vi "results_interface.vi"() -> ()   [LabVIEW 2015]
panel:
  out "Exerimement List by Group":string[](array[string])
  out "List of experiments":string[](array[string])
  out "Exeperiments names":string[](array[string])
  out "Experiment Group Names List":string[](array[string])
  out "Batch List by Material":string[](array[string])
  out "Batch list without IDs":string[](array[string])
  out "List of material IDs":string[](array[string])
  out "Material Name List":string[](array[string])
  out "Delimited Input String":string
  in  "Tab Control":enum32{"Controls", "Insights", "Debug"}(tab)
  in  "Create Heatmap":bool
  in  "Maxiumum Mass (kg)":dbl=1.0000000000000113e-10 format="%#_4e"
  in  "Minimum Mass (kg)":dbl=1.000000000000002e-30 step=1.0 format="%#_6e"
  in  "Batches list":i32[](listbox)
  in  "Confirm Experiments":bool
  in  "Experiment Listbox":i32[](listbox)
  in  "Show expeirments":bool
  in  "Experiment ID":string="All"
  in  "Confirm Selection":bool
  out "Authentication Failure":bool
  in  "Authenticate":bool
  out "Numeric":dbl
  in  "Password":string="dust"
  in  "Username":string="root"
  in  "Server IP Address":string="localhost"
  out "Poor Rate":string
  out "Optimal Rate":string
  out "User warnings":string
  in  "Calculate Results":bool
  in  "End Program":bool
  in  "Velocity Minimun  (km/s)":dbl min=0.0 max=100.0
  in  "Dust Material":string(combo)="Any Material"
  in  "Estimate Session Quality":cluster{i32, i32}(slide)={3, 5} scale=0.0..5.0
  out "Valid Path":bool
  out "Finished Sessions":bool
  out "Calculating":bool
  in  "Estimate Dust Quality":cluster{i32, i32}(slide)={3, 5} scale=0.0..5.0
  in  "Dust ID":string="Any"
  in  "Lower Integer Timestamp":i64=1375737549000 min=1340137854565 max=2062085784667 step=10000000
  in  "Upper Integer Timestamp":i64=2225999960000 min=1340137854565 max=2040137854565 step=10000000
  in  "Upper Timestamp":timestamp=timestamp(4308844760.779092 s since 1904-01-01)
  in  "Lower Timestamp":timestamp=timestamp(3458582349.4224453 s since 1904-01-01)
  in  "Velocity Maximum (km/s)":dbl=100.0 min=0.0 max=100.0
  out "Average Rate of Particle Detection":string
  out "Calculating Sessions":bool
  out "Cleaning Up":bool
  out "Working Directory":path
  in  "List Batches":bool
  in  "Experiment Group":string(combo)
  out "Results Output":string
  in  "Tab Control 2":T1(tab)
  in  "Tab Control 4":T2(tab)
  out "avg rate":picture
  out "avg count":picture
  out "avg runtime":picture
  in  "Tab Control 5":T2(tab)
  out "optimal rates":picture
  out "optimal count":picture
  out "optimal runtime":picture
  in  "Tab Control 6":T2(tab)
  out "poor rates":picture
  out "poor counts":picture
  out "poor runtimes":picture
  in  "Tab Control 7":T3(tab)
  out "2D rates":picture
  out "2D particle distribution":picture
  out "2D runtime":picture
  in  "Tab Control 3":T4(tab)
  out "Session Quality Breakdown":picture
  out "Session Particle Quality Breakdown":picture
  out "Session Duration Breakdown":picture
  out "Session Dust Event Count Breakdown":picture
  out "Session Generator Output":string
  out "Results Error/Debug":string
  out "Rate Results Request":string
  # "Note: takes upwards of two minutes, placed in heatmap folder"
  # "To calculate the rate of dust detection over a velocty range, a set of histograms is made, with bins for each .1km/s. The total runtime, detections, and rate over each bin are then calculated. Keep in mind the graphs here while maintaining the trends seen, their values reflect the bin size."
  # "The sessions are designated a quality:\n1: Maintenance session\n2: Low number of particle detections <10\n3: Low runtime < 20 min\n4: Standard sessions\n5: High dust event count (productive session)"
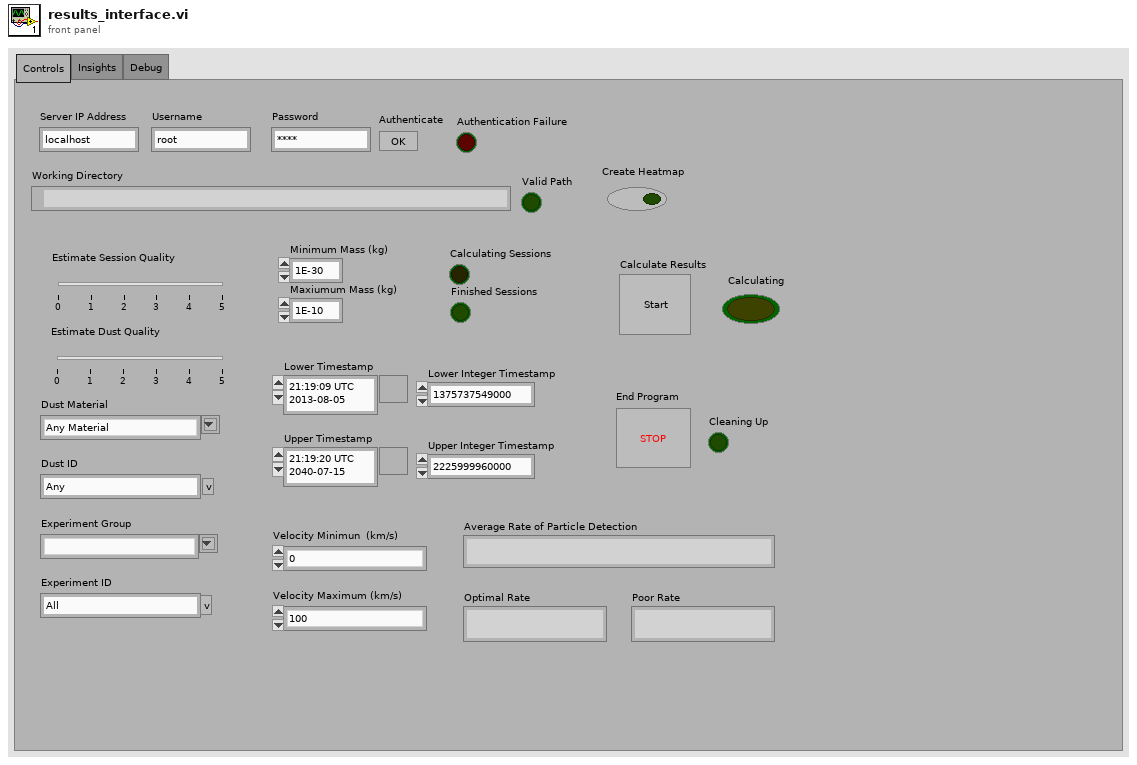
[diagram p1: front panel]
types:
  T1 = enum32{"Rate Insights - Average Results", "Rate Insights - Optimal Results", "Rate Insights - Poor Results", "Heatmaps", "Results Breakdown"}
  T2 = enum32{"Average Rates", "Average  Events", "Average Runtime"}
  T3 = enum32{"Particle Distribution", "Rate Distribution", "Runtime Distribution"}
  T4 = enum32{"Session Quality ", "Particle Quality", "Session Duration", "Session Event Counts"}
  T5 = cluster{string, string, string, string, string, string, string, string, string, string, string, string, string}
  T6 = cluster{"Velocity Minimun  (km/s)":dbl, "Velocity Maximum (km/s)":dbl}
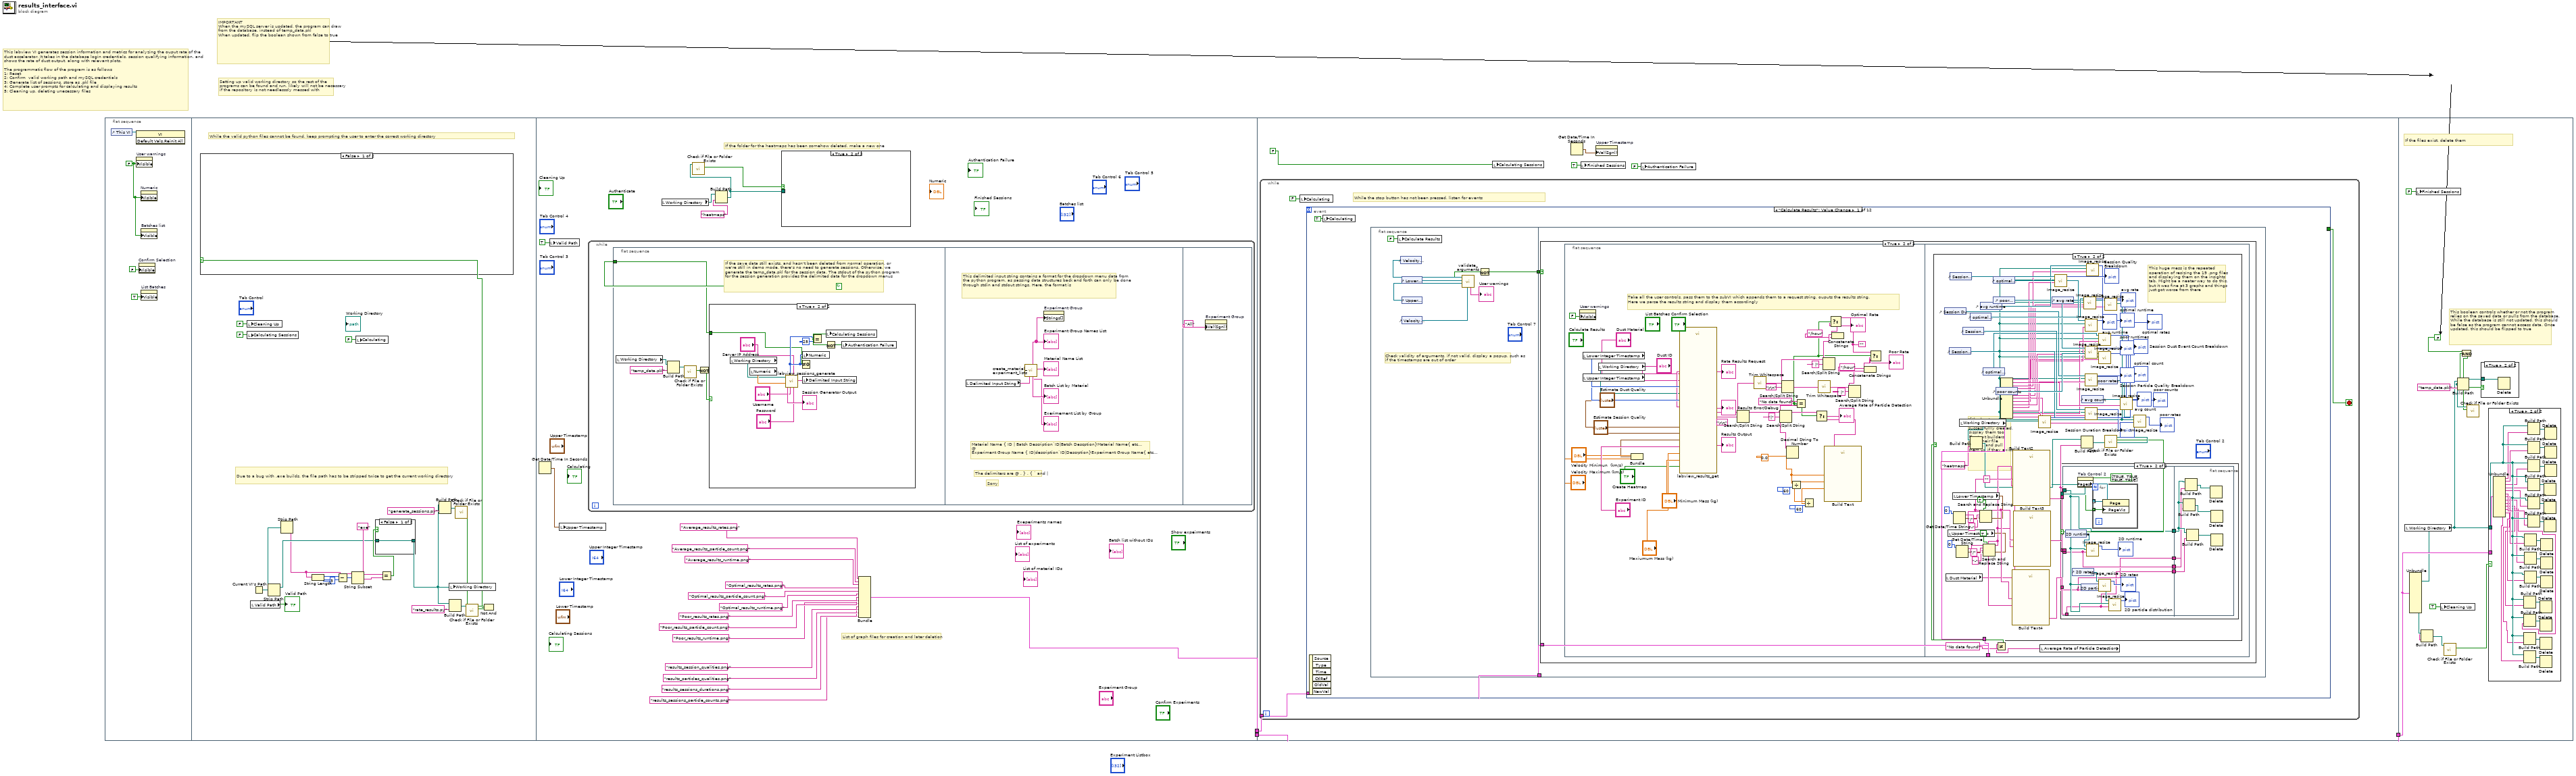
[diagram p0: block diagram]
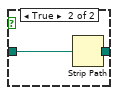
[diagram p2: hidden frame]
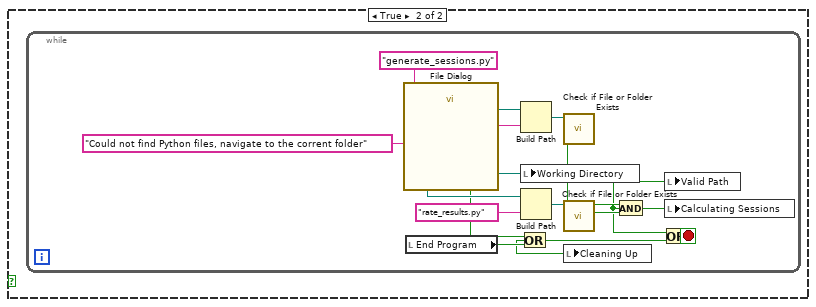
[diagram p3: hidden frame]
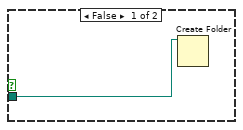
[diagram p4: hidden frame]
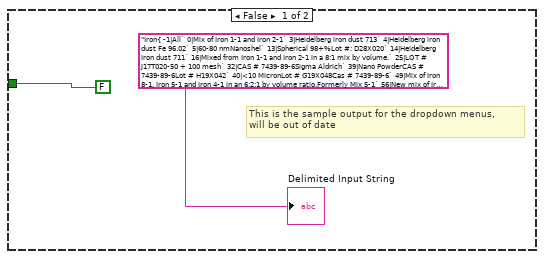
[diagram p5: hidden frame]
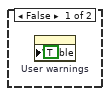
[diagram p6: hidden frame]
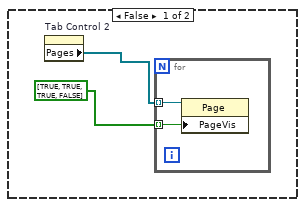
[diagram p8: hidden frame]
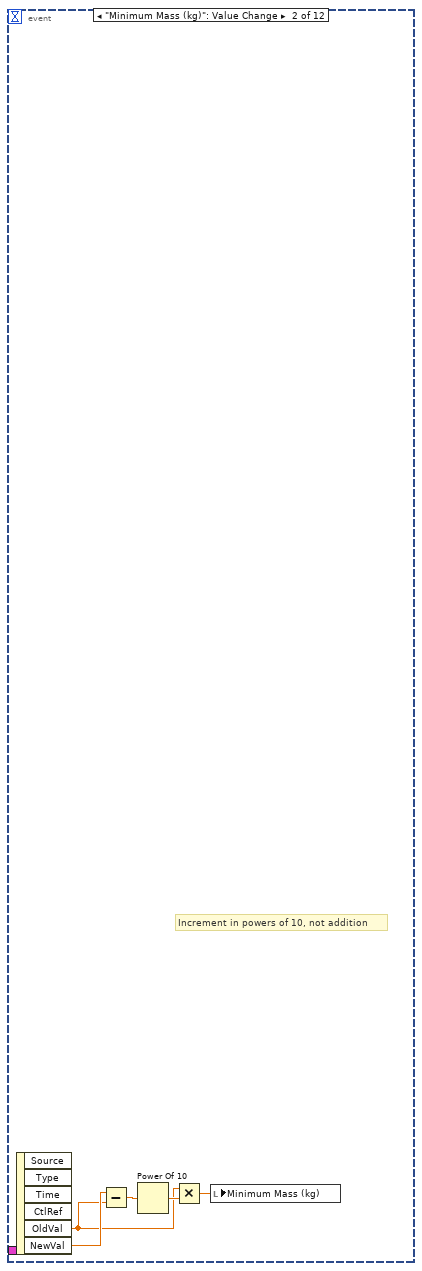
[diagram p9: hidden frame]
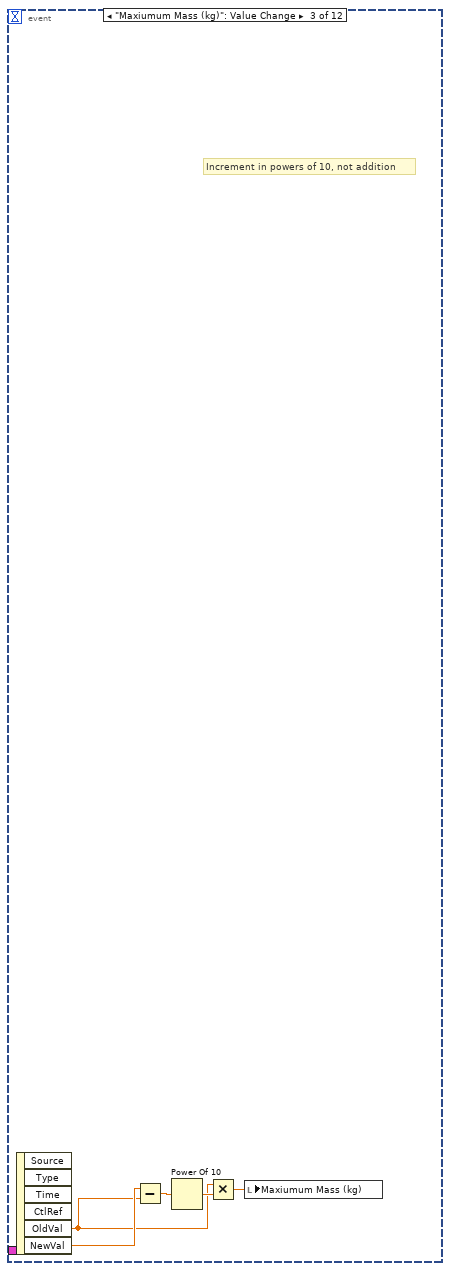
[diagram p10: hidden frame]
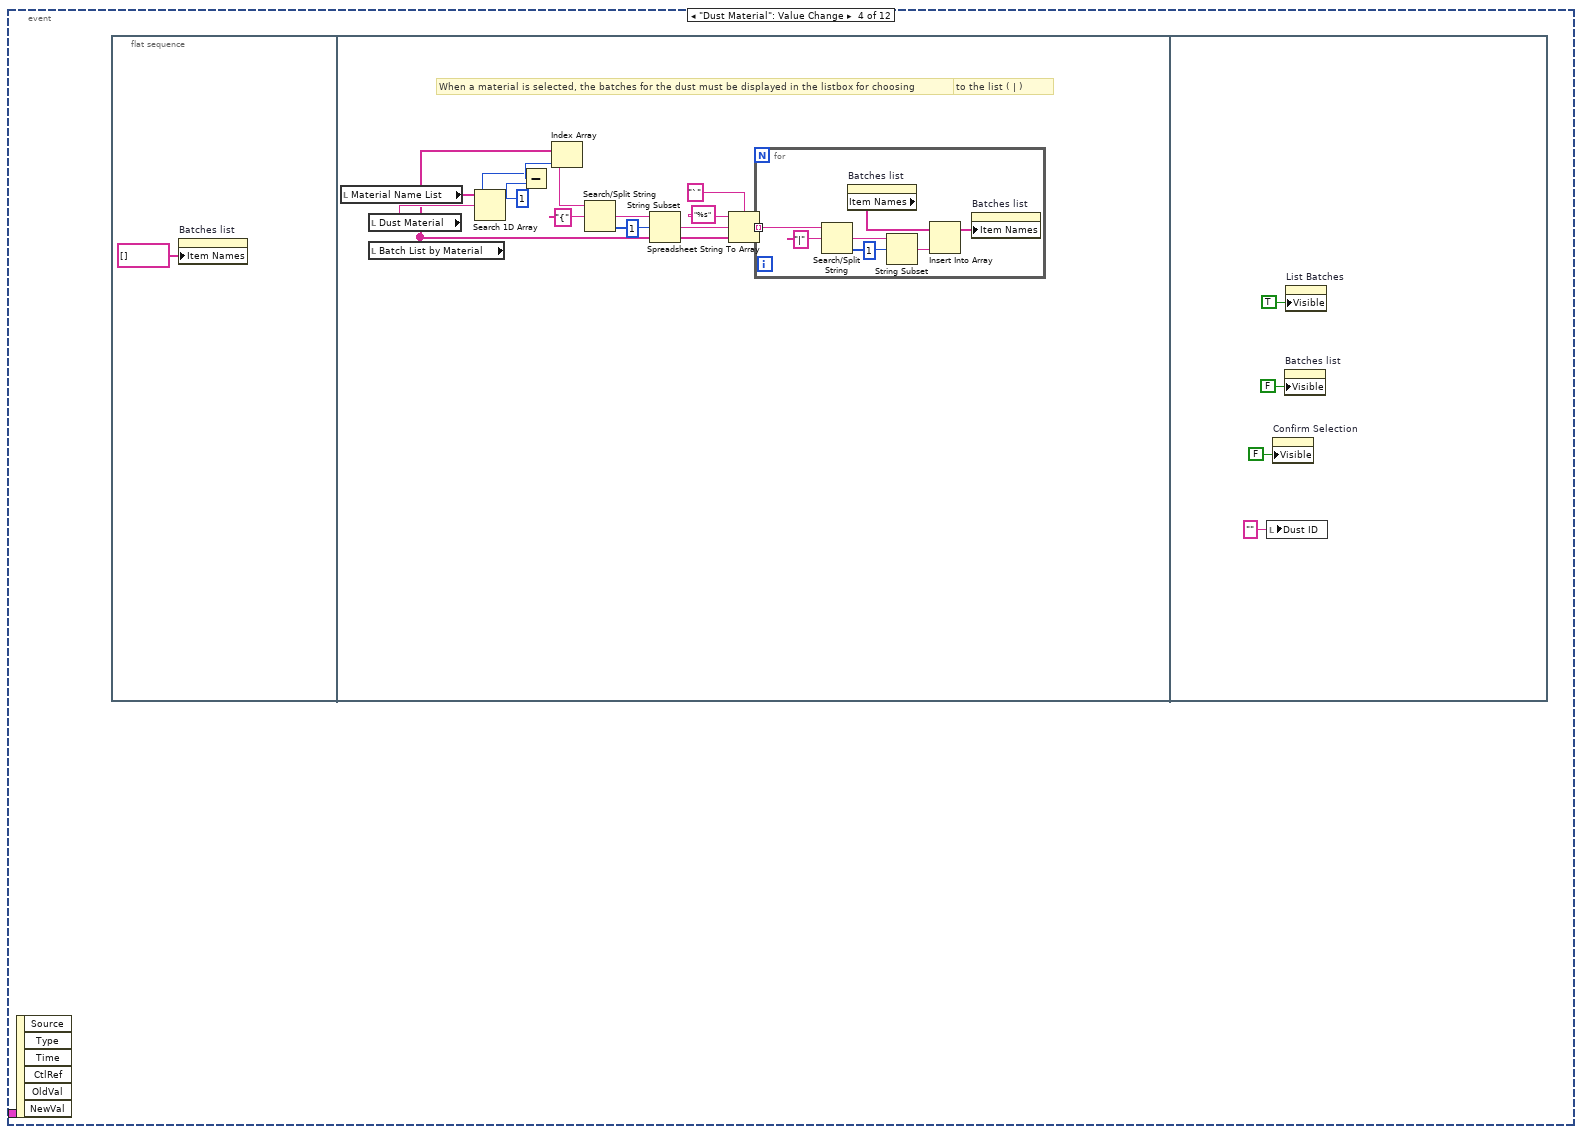
[diagram p11: hidden frame]
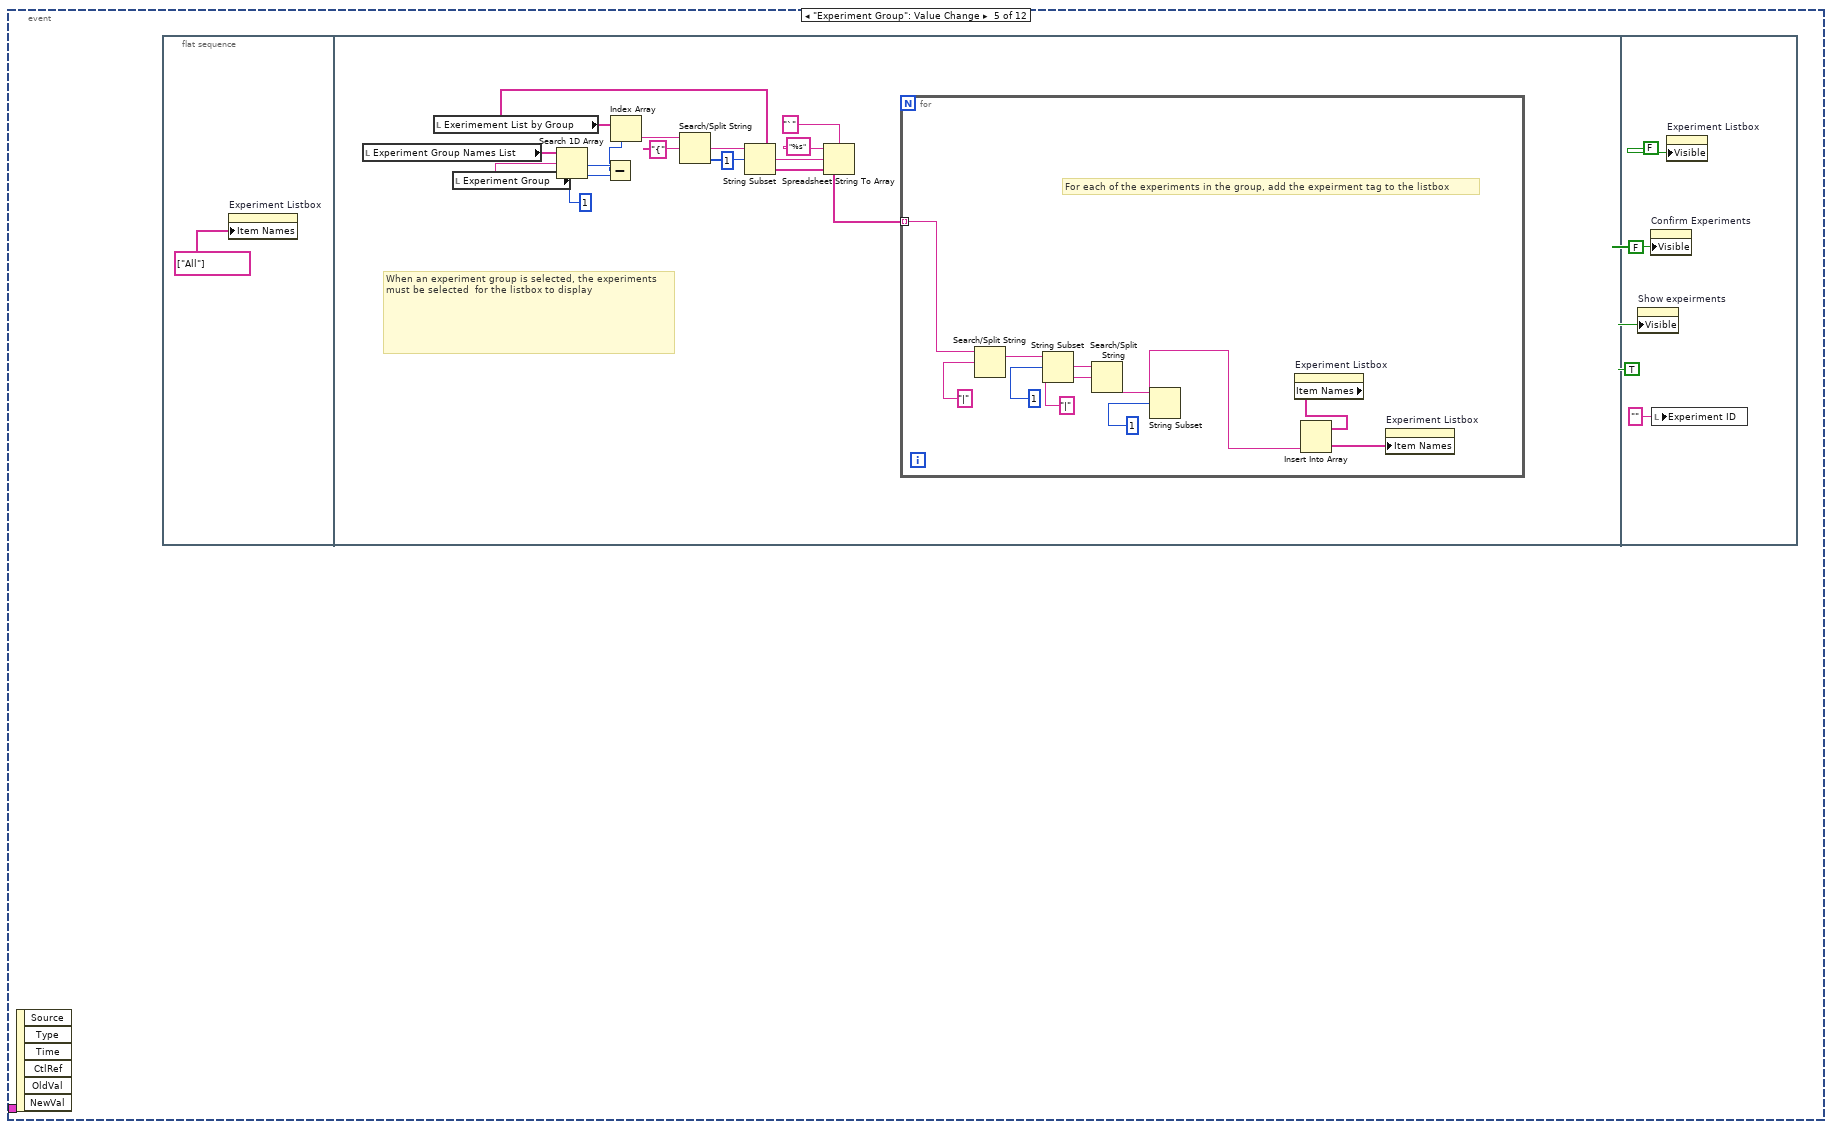
[diagram p12: hidden frame]
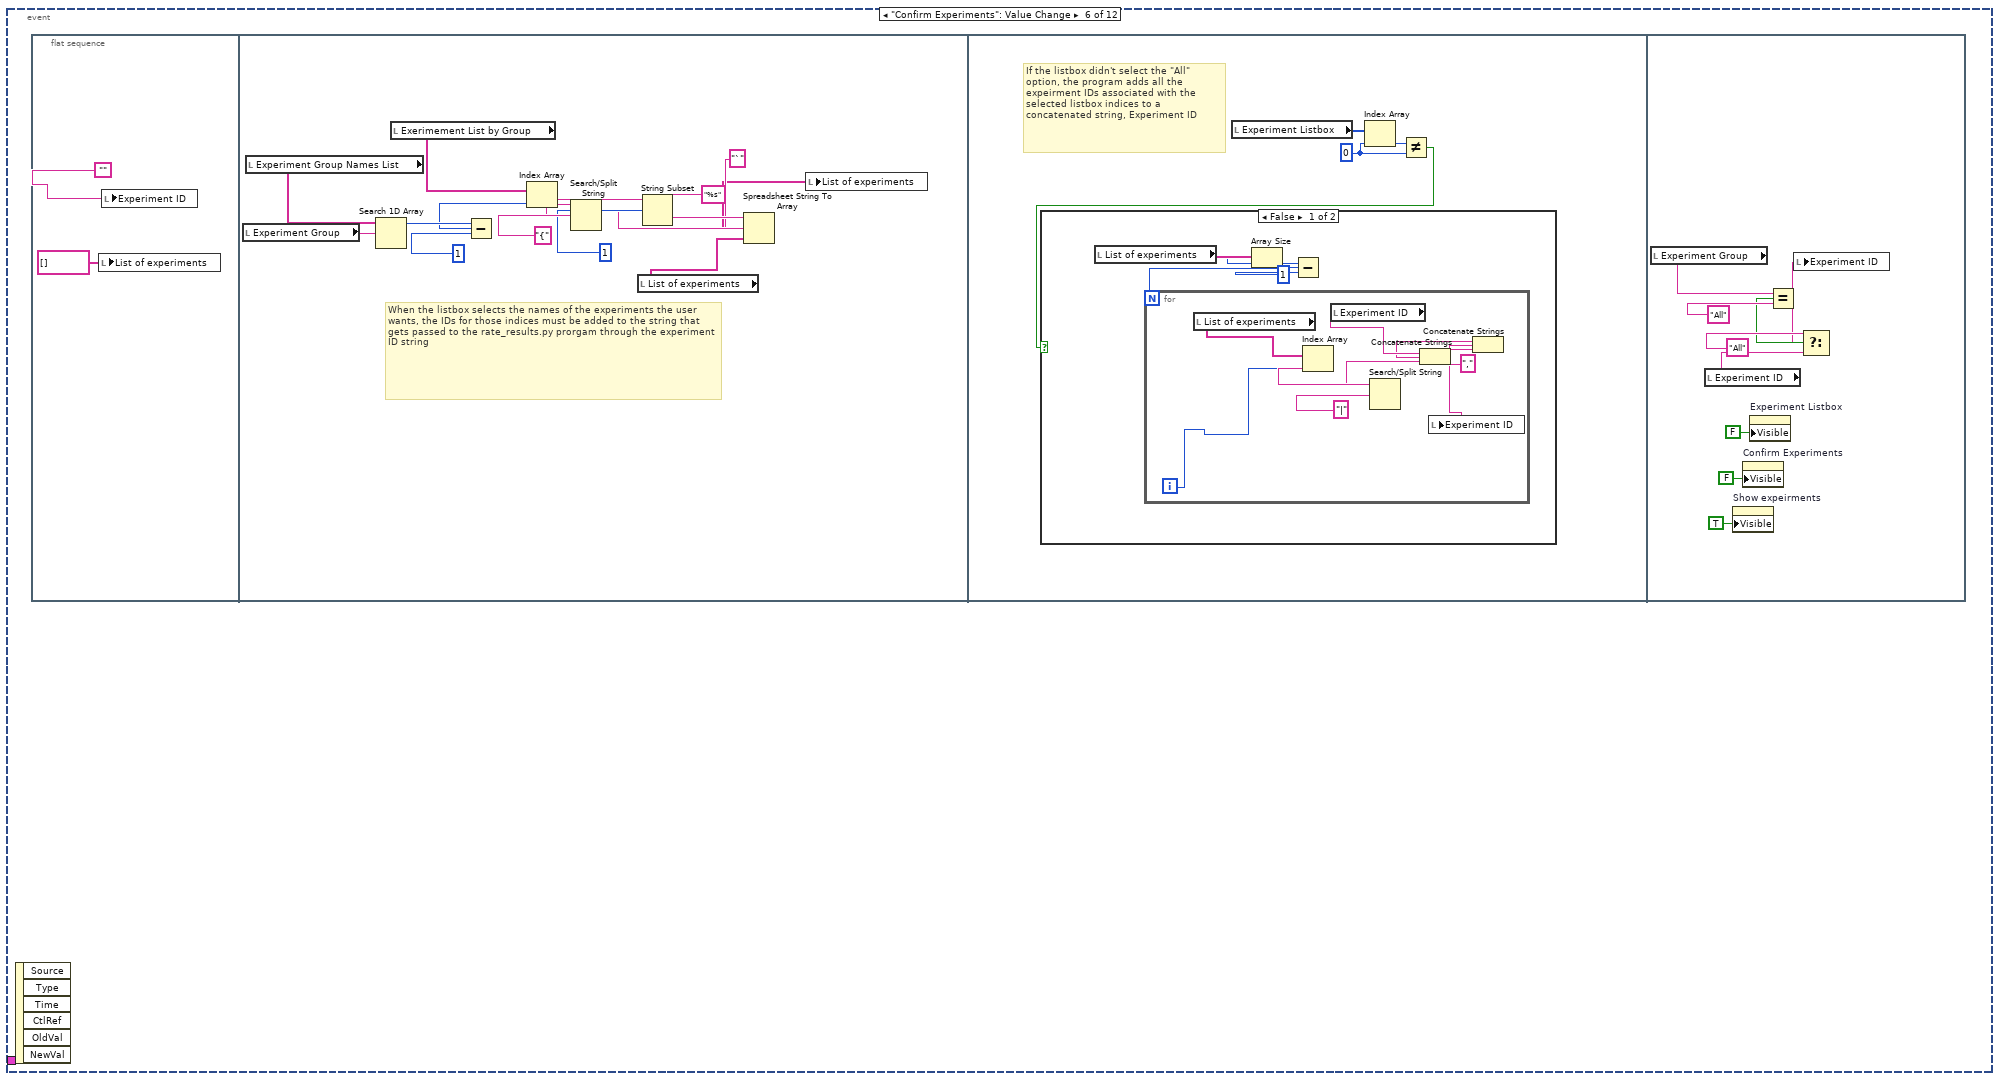
[diagram p13: hidden frame]
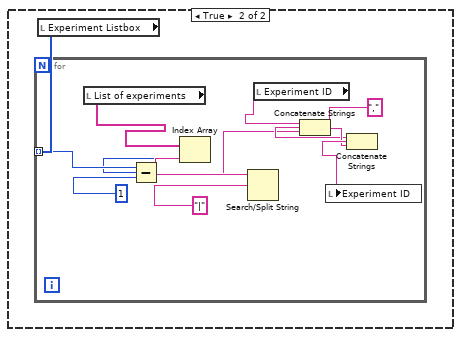
[diagram p14: hidden frame]
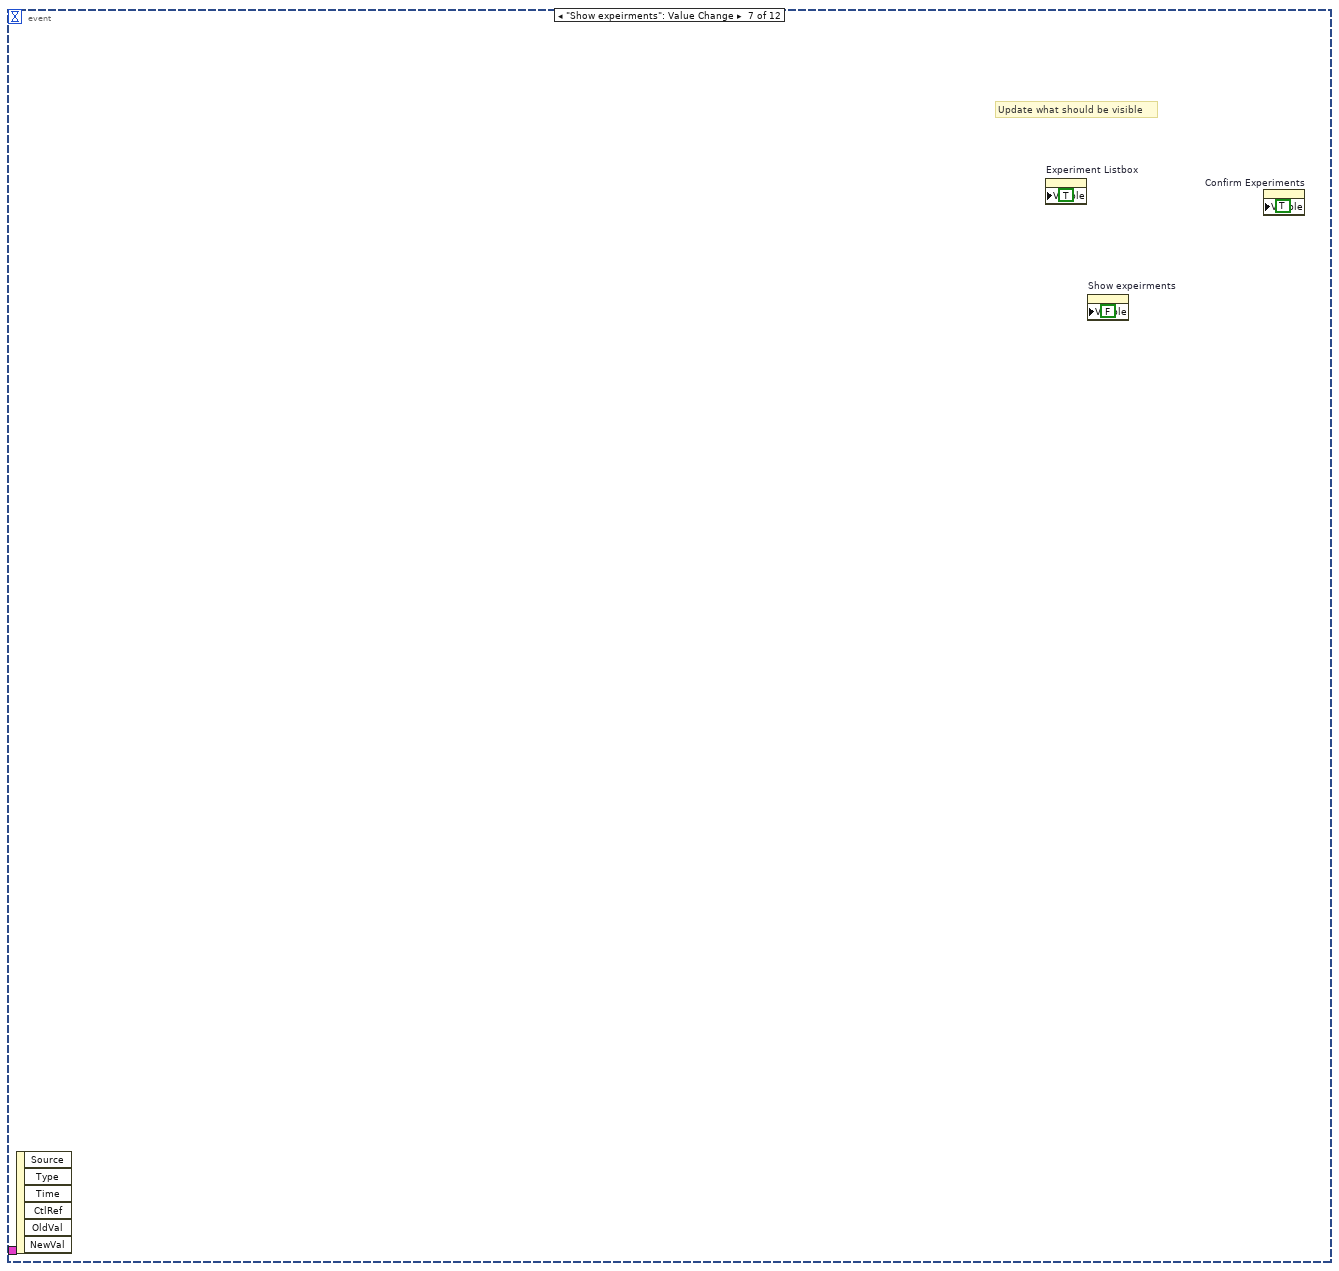
[diagram p15: hidden frame]
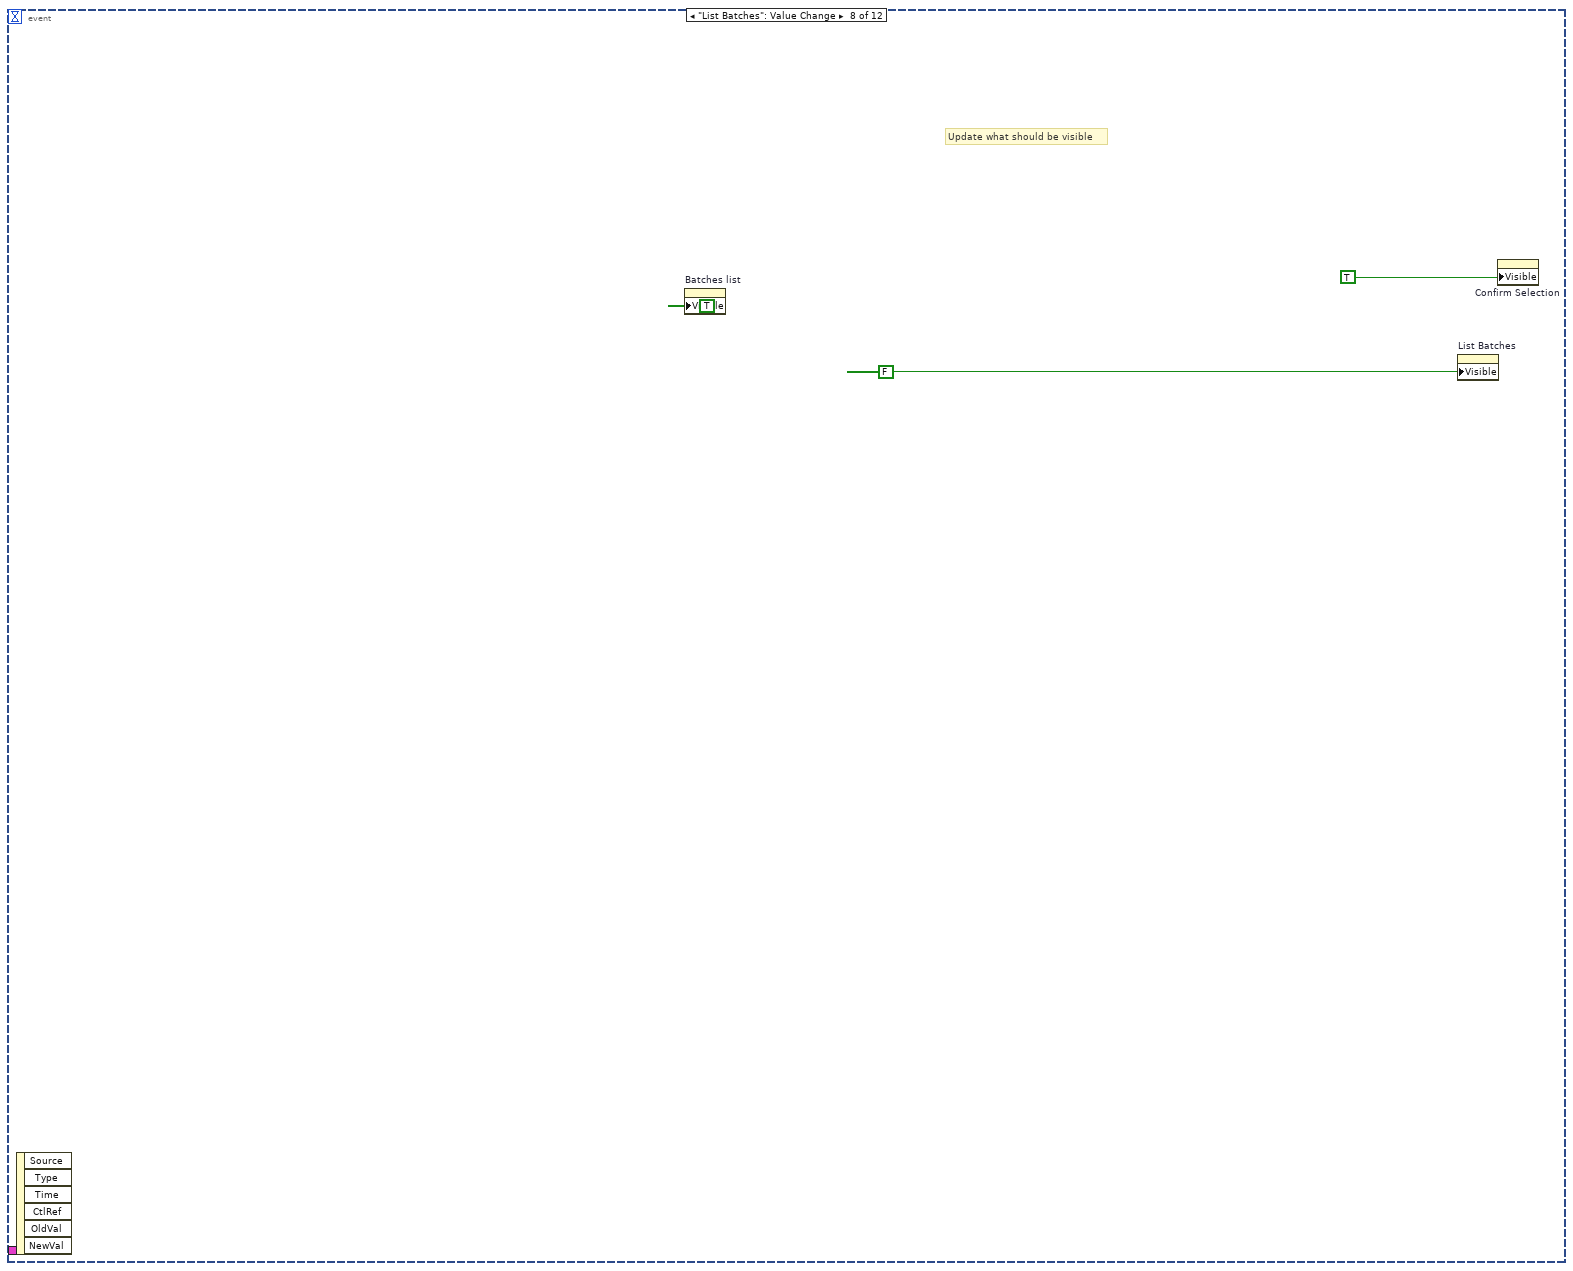
[diagram p16: hidden frame]
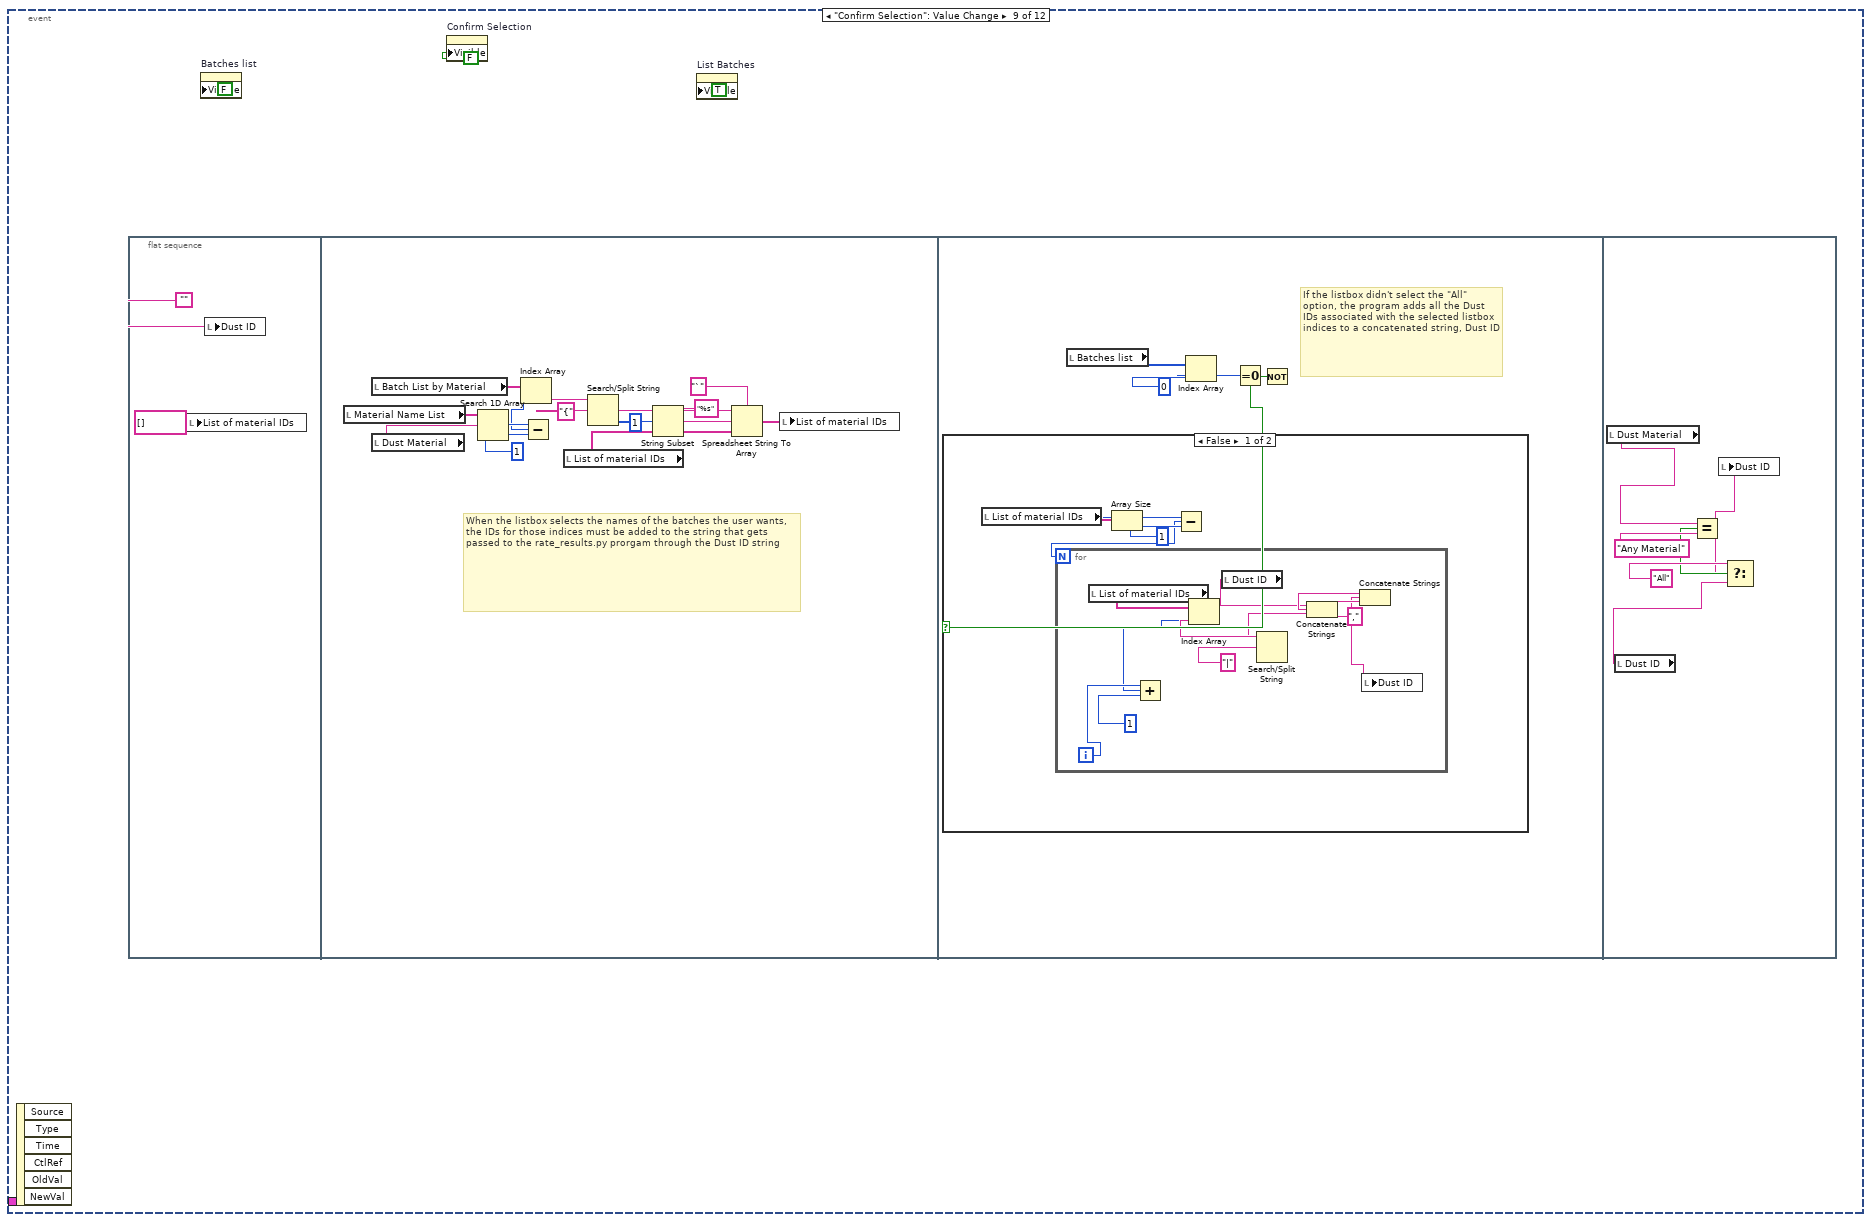
[diagram p17: hidden frame]
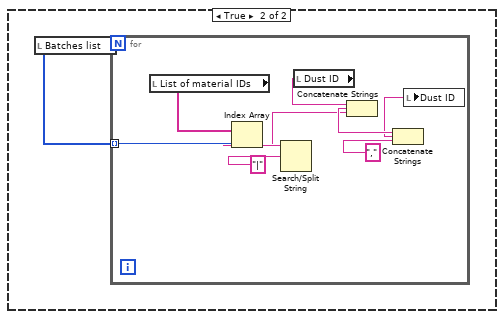
[diagram p18: hidden frame]
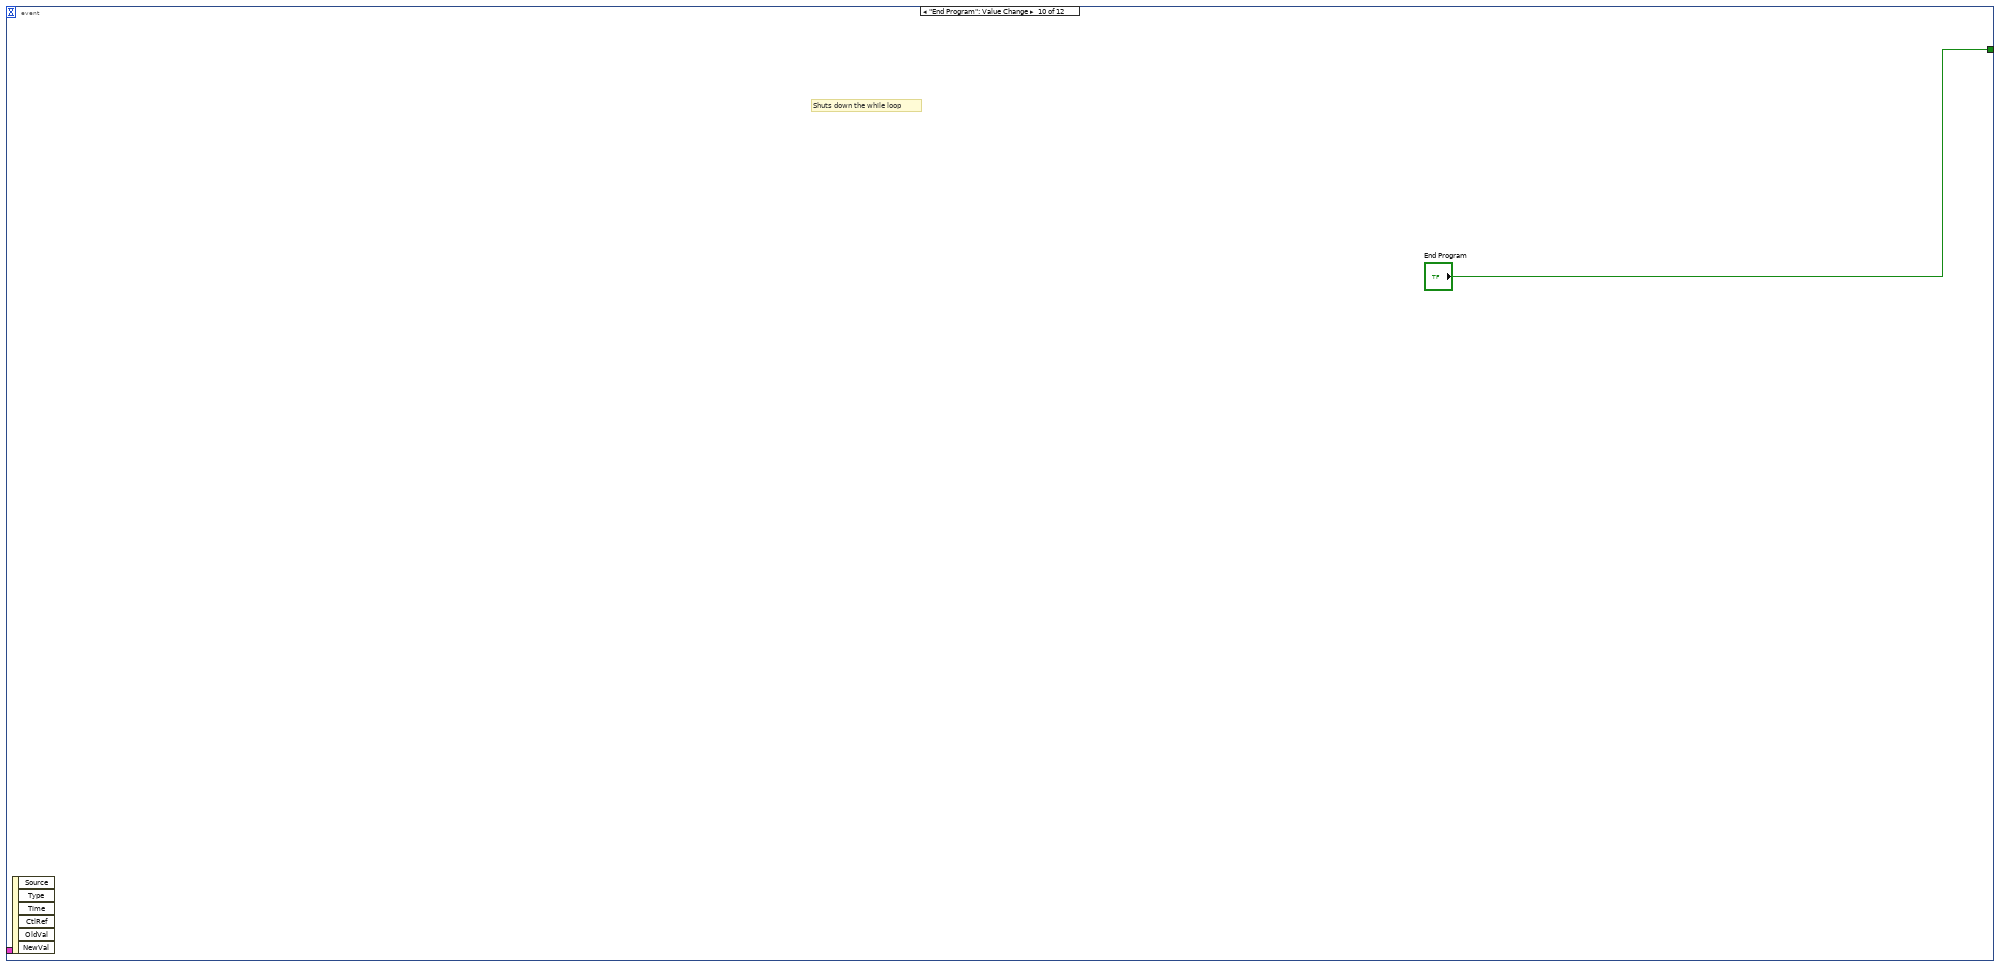
[diagram p19: hidden frame]
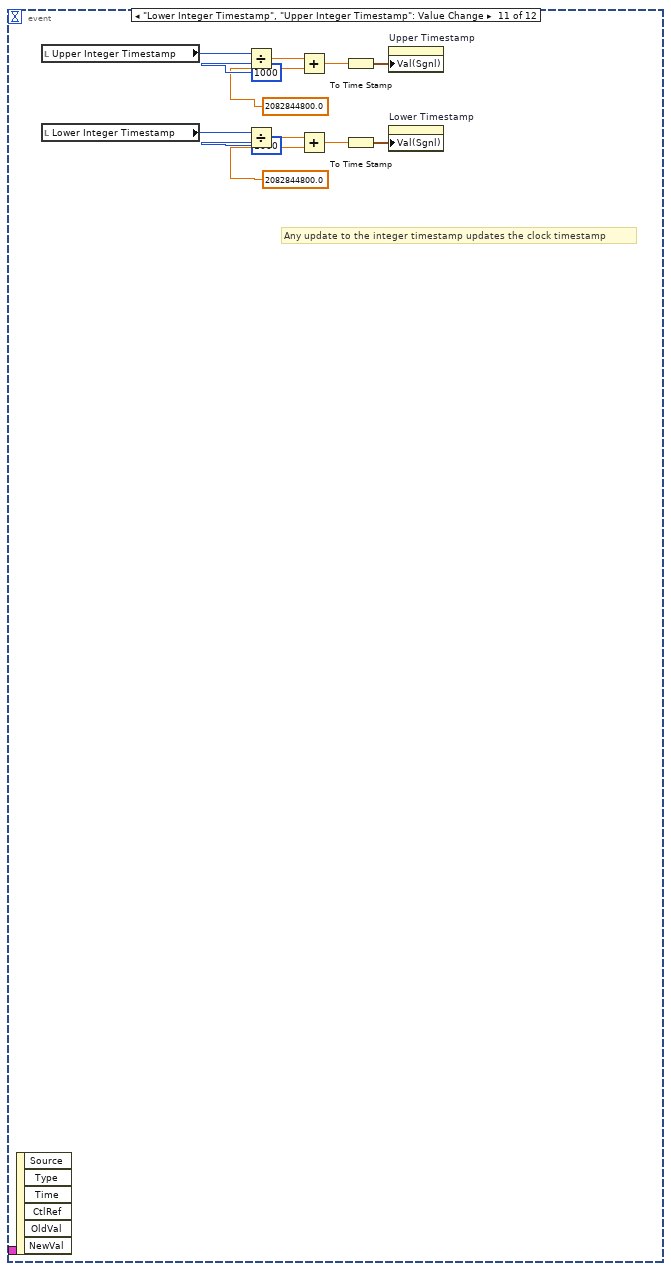
[diagram p20: hidden frame]
diagram:
  # "IMPORTANT\nWhen the mySQL server is updated, the program can draw from the database, instead of temp_data.pkl\nWhen updated, flip the boolean shown from false to true"
  # "Setting up valid working directory so the rest of the programs can be found and run, likely will not be necessary if the repository is not needlesssly messed with"
  # "This labview VI generates session information and metrics for analyzing the ouput rate of the dust accelerator. It takes in the database login credentials, session qualifying information, and shows the rate of dust output, along with relevant plots. \n\nThe programmatic flow of the program is as follows\n1: Reset\n2: Confirm  valid working path and mySQL credentials\n3: Generate list of sessions, store as .pkl file\n4: Complete user prompts for calculating and displaying results\n5: Cleaning up, deleting unecessary files"
  n1 = flat-sequence {
    tunnel: [w60] -> w3
    tunnel: [w60] -> w1
    tunnel: w3 -> [w98]
    tunnel: [w97] -> w2
    tunnel: w1 -> [w97]
    tunnel: w2 -> [w480]
    frame #0 {
      w6 = FALSE
      n2 = control-ref of="This VI"() -> (w7:refnum<vi>)
      n3 = invoke class="VI" method="Default Vals.Reinit All"(reference=w7) -> ()  [unwired: 2 in, 3 out]
      n4 = property on="User warnings" class="Str"("Visible"=w6) -> ()  [unwired: 2 in, 2 out]
      n5 = property on="Confirm Selection" class="Bool (strict)"("Visible"=FALSE) -> ()  [unwired: 2 in, 2 out]
      n6 = property on="Numeric" class="DigNum (strict)"("Visible"=w6) -> ()  [unwired: 2 in, 2 out]
      n7 = property on="Batches list" class="LstBox (strict)"("Visible"=w6) -> ()  [unwired: 2 in, 2 out]
      n8 = property on="List Batches" class="Bool (strict)"("Visible"=TRUE) -> ()  [unwired: 2 in, 2 out]
    }
    frame #1 {
      # "While the valid python files cannot be found, keep prompting the user to enter the correct working directory"
      # "Due to a bug with .exe builds, the file path has to be stripped twice to get the current working directory"
      n9 = local write "Cleaning Up"(FALSE ("Cleaning Up")) -> ()
      n10 = local write "Calculating Sessions"(FALSE ("Calculating Sessions")) -> ()
      n11 = local read "Valid Path"() -> (→"Valid Path":bool)
      n12 = Current VI's Path() -> (path=w18:path)
      n13 = Strip Path(path=w18) -> (stripped path=w13:path)  [unwired: 1 out]
      n14 = Strip Path(path=w13) -> (name=w8:string)  [unwired: 1 out]
      n15 = String Length(string=w8) -> (length=w11:i32)
      n16 = Subtract(x=w11, y=3) -> (x-y=w9:i32)
      n17 = String Subset(string=w8, offset (0)=w9) -> (substring=w16:string)  [unwired: 1 in]
      n18 = local write "Calculating"(FALSE) -> ()
      n19 = Equal?(x="exe", y=w16) -> (x = y?=w14:bool)
      n20 = case shown="False" w14 {
        tunnel: w13 -> [w29 w31]
        tunnel: [w29 w30] -> w12
        frame False {
        }
        frame True {
          n21 = Strip Path(path=w31) -> (stripped path=w30:path)  [unwired: 1 out]
        }
      }
      n22 = Build Path(base path=w12, name or relative path="generate_sessions.py") -> (appended path=w20:path)
      n23 = local write "Working Directory"(w12) -> ()
      n24 = Build Path(base path=w12, name or relative path="rate_results.py") -> (appended path=w19:path)
      n25 = call <vilib>:"Check if File or Folder Exists.vi"("path"=w20) -> ("file or folder exists?"=w24:bool)  [unwired: 8 in, 2 out]
      n26 = call <vilib>:"Check if File or Folder Exists.vi"("path"=w19) -> ("file or folder exists?"=w23:bool)  [unwired: 8 in, 2 out]
      n27 = Not And(1:w23, 2:w24) -> (0:w22:bool)
      n28 = case shown="False" w22 {
        frame False {
        }
        frame True {
          n29 = while {
            stop <- w38 stop-if-true
            n30 = call "File Dialog"("prompt"="Could not find Python files, navigate to the corrent folder") -> ("selected path"=w36:path, "cancelled"=w34:bool)  [unwired: 11 in, 2 out]
            n31 = local read "End Program"() -> (w35:bool)
            n32 = Or(x=w34, y=w35) -> (x .or. y?=w33:bool)
            n33 = Build Path(base path=w36, name or relative path="generate_sessions.py") -> (appended path=w43:path)
            n34 = local write "Working Directory"(w36) -> ()
            n35 = Build Path(base path=w36, name or relative path="rate_results.py") -> (appended path=w42:path)
            n36 = call <vilib>:"Check if File or Folder Exists.vi"("path"=w43) -> ("file or folder exists?"=w40:bool)  [unwired: 8 in, 2 out]
            n37 = call <vilib>:"Check if File or Folder Exists.vi"("path"=w42) -> ("file or folder exists?"=w39:bool)  [unwired: 8 in, 2 out]
            n38 = local write "Cleaning Up"(w33) -> ()
            n39 = And(x=w40, y=w39) -> (x .and. y?=w37:bool)
            n40 = Or(x=w37, y=w33) -> (x .or. y?=w38:bool)
            n41 = local write "Valid Path"(w37) -> ()
            n42 = local write "Calculating Sessions"(w37) -> ()
          }
        }
      }
    }
    frame #2 {
      # "List of graph files for creation and later deletion"
      # "If the folder for the heatmaps has been somehow deleted, make a new one"
      n43 = Get Date/Time In Seconds() -> (seconds since 1Jan1904=w59:timestamp)
      n44 = local write "Valid Path"(TRUE) -> ()
      n45 = local write "Upper Timestamp"(w59) -> ()
      n46 = while {
        stop <- w66 continue-if-true
        n47 = flat-sequence {
          tunnel: [w72] -> w66
          frame #0 {
            # "If the save data still exists, and hasn't been deleted from normal operation, or we're still in demo mode, there's no need to generate sessions. Otherwise, we generate the temp_data.pkl for the session data. The stdout of the python program for the session generation provides the delimited data for the dropdown menus"
            n48 = local read "Working Directory"() -> (w70:path)
            n49 = Build Path(base path=w70, name or relative path="temp_data.pkl") -> (appended path=w69:path)
            n50 = call <vilib>:"Check if File or Folder Exists.vi"("path"=w69) -> ("file or folder exists?"=w67:bool)  [unwired: 8 in, 2 out]
            n51 = Not(x=w67) -> (.not. x?=w68:bool)
            n52 = case shown="True" w68 {
              tunnel: [FALSE w76] -> w72
              frame False {
                # "This is the sample output for the dropdown menus, \nwill be out of date"
                "Delimited Input String" <- "Iron{ -1|All` 0|Mix of Iron 1-1 and Iron 2-1` 3|Heidelberg iron dust 713` 4|Heidelberg iron dust Fe 96.02` 5|60-80 nmNanoshel` 13|Spherical 98+%Lot #: D28X020` 14|Heidelberg Iron dust 711` 16|Mixed from Iron 1-1 and Iron 2-1 in a 8:1 mix by volume.` 25|LOT # J17T020-50 + 100 mesh` 32|CAS # 7439-89-6Sigma Aldrich` 39|Nano PowderCAS # 7439-89-6Lot # H19X042` 40|<10 MicronLot # G19X048Cas # 7439-89-6` 49|Mix of Iron 8-1, Iron 5-1 and Iron 4-1 in an 6:2:1 by volume ratio.Formerly Mix 5-1` 56|New mix of Iron 10` 59|First time we have used the big scoop.` 97|Large Iron, 6-10 micron.`}Olivine{ -1|All` 1|Shot very well and got fastest particle seen so far at 69 km/s` 67|PPY-Coated Olivine. (lee Fielding V. Shezzield) 8/2014` 68|PPY-Coated SYNTHETIC Olivine.  (Lee Fielding V. Shezzield)` 78|Unlabed blue lid bottle` 79|PPy coated (20%) olivine` 80|PPy (2%) coated Olivine` 81|Olivine Powder, not ground. Natural History museum, UK` 87|Pt coated Olivine. From John Hillier  from England. Freeze dried`}Nickel{ -1|All` 2|NanoshelIs very clumpy.  After shooting, much of the dust was stuck together in sheets.  Particle size range appears to be much larger than indicated, but could be caused by clumped together dust.` 33|CAS # 7440-02-0` 45|NanoshelNanoPowder` 46|Alfa Aesar Nickel PowderLot: D06X023` 47|Alfa Aesar Nickel PowderLot: H10X012`}Graphite{ -1|All` 6|` 7|` 18|`}Silver{ -1|All` 8|` 60|Silver Nanopowder from Nanoshell. 80-100nm. NS6130-01-101  7440-22-4` 84|Silver coated SiO2 particles. From: Jung-Hyun Lee & Carson Meredith. ~300nm`}Latex{ -1|All` 9|Coated with PolypyrroleSample 3` 10|PPY Coated, SP Armes` 22|PPY coated sulfur rich PMPV` 52|PEDOT coated Latex` 53|Polyaniline Coated` 54|PPY Coated` 55|PPY coated: PBnS` 70|PPy coated sulfur rich (PMPV) latex,  9/2008`}Mix{ -1|All` 11|Mix 5:8 ratio of Graphite 1-1 and 2-1.` 12|Mix 3:8 ratio of Graphite 1-1 and 2-1.` 37|8:1 mix of Iron-8-1 and Iron-4-1.  Seems to have a lack of large and/or slow particles` 41|Mix of 711 and 96.02 (6-1 and 2-1)Does not form homogenous mix` 42|Now FE 10-1Mix of Iron 8-1, Iron 5-1 and Iron 4-1 in an 6:2:1 by volume ratio.` 48|8:1 Mixture of Ni 1-1 and 3-1 respectivly`}Moly{ -1|All` 15|`}Tungsten{ -1|All` 17|WC 59/6`}Silica{ -1|All` 19|PPY coated nanocomposite APS` 20|PPY coated nanocomposite FeCl3` 36|PPY coated SIlicaVeerle's Dust` 38|PPY coated silica made by Prof. Armes for Zoltan` 43|PPY coated Silica made by Prof. Armes` 44|PPU coated silica made with APS by Prof. ArmesNano-composites` 69|PEDOT coated silica particles made with APS. 100nm. 9/2008` 71|PPY nanocomposites made with FeCl3` 74|PPy coated, 5% PPy giving a shell of 12nm thickness`}PvA{ -1|All` 21|PPY coated` 72|PVA stabilized PPY coated` 75|PvA (9000) PPy coated CL doped` 76|` 77|PvA(9000) PPy coated Tosylate doped.`}Pyrhotite{ -1|All` 23|PPY coated`}JSC 1{ -1|All` 24|25 um`}ACS{ -1|All` 26|Cas # 100-97-0`}Stainless Steel{ -1|All` 27|53-63` 29|` 30|45-53`}Flurothane{ -1|All` 28|CAS # 206-44-0`}Perylene{ -1|All` 31|Batch# 04215PY`}Anthracene{ -1|All` 34|LOT # G4455A`}Meteor Simulant{ -1|All` 35|`}Carbon Aerogel{ -1|All` 50|Carbon Aerogel from Veerle` 85|New Carbon Aerogel from Veerle, waiting to see if she is coming back to boulder.`}Polystyrene{ -1|All` 51|PPY coated: 20 nm coating thickness` 103|SAW 3T \"5.04um\" 7.3% PPy coated polystyrene.  John Mathies.  Looks more like 2-9um diameter particles`}Carbon Nanotube{ -1|All` 57|Avg. Length: 1-10 MicronAvg. Diam: 3.5 nmPN#: 755168` 58|Avg. Length: 3 micronAvg. Diam: 3.5 nmPN# 755141`}Calcium Carbonate (Albaglos){ -1|All` 61|ALBAGLOS calcum carbonate. PPY coated. mean particle size: .8 micron. 4% PPY coated.` 62|ALBAGLOS calcum carbonate. PPY coated. mean particle size: .8 micron. 8% PPY coated.` 63|ALBAGLOS calcum carbonate. PPY coated. mean particle size: .8 micron. 12% PPY coated.` 64|ALBAFIL calcum carbonate. PPY coated. median particle size: .7 micron. 4% PPY coated.` 65|ALBAFIL calcum carbonate. PPY coated. median particle size: .7 micron. 8% PPY coated.` 66|ALBAFIL calcum carbonate. PPY coated. median particle size: .7 micron. 12% PPY coated.`}PMMA{ -1|All` 73|PPy coated PMMA`}Pyrrhotite{ -1|All` 82|PPy Coated`}Alumina{ -1|All` 83|PPy coated (21%) Alumina`}Orthopyrexene{ -1|All` 86|Pt coated Orthopyresene dust for Ralf Srama, from Heidelberg`}Aluminum{ -1|All` 88|Mix AL 1-1: parts: (1-2-1-1) <5micron, 800nm, 500nm, 60-80nm (spherical)` 89|Mix AL 1-2: parts: (1-3-2) 10-14 micron, 3-4.5 micron, 4.5-7 micron` 90|50 50 mix, did not work` 91|mix 4: 90% mix 2, 5% 40-60nm, 10% 80-100nm` 102|mix 4: 90% mix 2, 5% 40-60nm, 10% 80-100nm`}San Carlos Olivine{ -1|All` 92|From Anton Kearsley, formerly of the natural history muesum, London`}Antigorite{ -1|All` 93|from Jon Hillier. Sample A from Mario. Rock forming hydrous magnesium ironphyllosilicate`}Saponite{ -1|All` 94|From Jon Hillier. Sample A from Mario.`}Saponite Iron Mix{ -1|All` 95|65% Iron (10>micron) 35% Saponite by volume. 10% Saponite by weight`}San Carlos Olivine Iron Mix{ -1|All` 96|San Carlos Olivine from John Huller. Olivine from Anton Kearsley, formerly NHMuseum, London. 1g Iron (10>um), 0.1g Olivine. Volume: 2:1 Iron to Olivne.`}Carbon Nanotube Mix{ -1|All` 98|Mix of double walled carbon nanotubes and large iron. Iron is 6-10 micron. Mix (weight) Iron: .51g, CnT: .04g 1:1 volume.`}Iron Sulfide{ -1|All` 99|SigAld: 268704: Iron Sulfide. cas-no: 1317-37-9. PPY coated by Armes for B. Farcy: NASA-GSFC`}Caco3 Cc2{ -1|All` 100|CaCo3 Iron mix. 1g iron (6-10um spherical) .25g CaCo3 (8% PPy coated ABAFIL)`}Tin{ -1|All` 101|Tin mix 1-1. 5g (45um) 1.3g (150um) Stock #US5001`}Indium Tin Oxide{ -1|All` 104|Less than 50 nm ITO. Greenish/plastic bottle`}@June Lightflash{3|1340137854565|Run 4.1`4|1340371855957|Run 12`}Anna Spectrometer{5|1349981735953|10-11`6|1349985613309|10-11 (10 and above)`7|1349985953948|10-11 (5 and above)`8|1350320678212|Open`9|1350324177150|5+ kms`10|1350399106565|open2`11|1350658222228|Alignment Testing`12|1350659007269|Alignment Testing 5+`13|1350675260142|Alignment Testing 5+ v2`14|1350675915189|Alignment Testing v2`15|1350919929794|Open 3`16|1350920178699|1.5+`17|1350920389614|5+ km/s 2`18|1350924305552|1+ km/s `19|1350924904821|5+ km/s `20|1350934504803|5+ km/s  3`21|1350938373024|1+ km/s  3`22|1350939192742|5+ km/s  4`23|1351003950828|5+ km/s 5`24|1351017706010|1+ km/s 5`25|1351092614663|Test6`26|1351111812025|Test7`27|1351113588699|Test8`28|1351177408411|Test9`29|1351181836487|Test10`30|1351183903829|Test11`31|1351198020885|Test12`32|1351198186258|Test12`33|1351266651057|Test12`34|1351270300998|Test13`35|1351271914223|Test14`36|1351277620410|Test15`37|1351524747978|Test16`38|1351626222403|Test1`79|1353348115144|Run 1 11/19`80|1353355731177|Run 2 11/19`81|1353434169850|Run 3 11/20`185|1361987988557|ANNA`189|1362158072692|ANNA2`190|1362170143460|ANNA2 MANANA`192|1362592740488|ANNA4 MANANA`193|1362674949243|ANNA5 MANANA`}NDA{39|1351626891706|Test1`40|1351627047629|Test1`41|1351873055449|Test1`42|1351874245476|Test1`139|1357582333966|test1`140|1357668281927|test2`141|1357845624455|test3`401|1385573319415|2013_11_27_test1`402|1385583531861|2013_11_27_test2`403|1385588567674|2013_11_27_test3`404|1385997950292|2013_12_02_test4`405|1386011221532|2013_12_02_test5`407|1386265180242|2013_12_05_test6`408|1386272505532|2013_12_05_test7`409|1386274806702|2013_12_05_test8`486|1396638344190|2014_04_04-NDA`487|1396641250299|2014_04_04-NDA2`488|1396642346896|2014_04_04-NDA3`489|1396644475531|2014_04_04-NDA4`490|1396647411727|2014_04_04-NDA5`491|1396647966793|2014_04_04-NDA6`492|1396648271002|2014_04_04-NDA7`493|1396650078010|2014_04_04-NDA7`494|1396650146339|2014_04_04-NDA8`687|1424194400637|2015_02_17-Test1`688|1424280410490|2015_02_18-Test2`689|1424284608723|2015_02_18-Test3`690|1424373702888|2015_02_19-Test1`691|1424547456909|2015_02_21-Test1`}Throop Foils{43|1352148187456|Test1`44|1352157954229|Test2`45|1352214744457|Test3`46|1352214831451|Test3`47|1352214866099|Test3`48|1352219122359|Test3`49|1352219186751|Test4`50|1352219202651|Test4`51|1352247672178|Test5`52|1352301848320|Test6`53|1352306010826|Test7`54|1352306045899|Test7`55|1352310272403|Test8`56|1352311799119|Test8`57|1352391736109|Test8`58|1352391793553|Test9`59|1352395335123|Test10`60|1352395368180|Test10`61|1352395377853|Test10`342|1381266809306|2013_10_09_test0`343|1381757233978|2013_10_14_test1`344|1381766221040|2013_10_14_test2`345|1381777410501|2013_10_14_test3`346|1381940722656|2013_10_16_test1`347|1381960904570|2013_10_16_test2`348|1382020385028|2013_10_17_test1`627|1416248172821|2014_11_17_test0`628|1416262110938|2014_11_17_test1`629|1416338814684|2014_11_18_test0`630|1416424093655|2014_11_19_test0`631|1416427877351|2014_11_19_test1`632|1416505749844|2014_11_20_test1`633|1416523363953|2014_11_20_test2`634|1416595704834|2014_11_21_test1`1408|1475967180450|2016_10_08_First_Foil_1`1409|1476117658204|2016_10_08_First_Foil_2`1411|1476241184618|10_08_2016_Throop_3`}November Lightflash{62|1352828561104|Source Testing`63|1352829245042|Source Testing`64|1352829315596|Source Testing (5+)`65|1352829964046|Source Testing (5+2)`66|1352830671032|Run1`67|1352836327304|Run2`68|1352839790796|Run3`69|1352844695231|Run4`70|1352911058990|Iridium initial tests`71|1352911217088|run5`72|1352916718809|Run6`73|1352926182955|Run7`74|1352932537538|Run8`75|1352933159018|Run9`76|1352999357125|Run10`77|1353012692164|Run11`78|1353085050742|Run12`}David Malaspina{82|1353948203208|Run1`83|1353952089669|Run2`84|1353966288977|Run3`85|1353969771586|Run4`86|1354035652963|Run5`87|1354046539507|Run6`88|1354119766986|Run7`89|1354132811267|Run8`90|1354207033284|Run9`91|1354215706374|Run10`92|1354227376014|Run11`}Keith the Drake{93|1354560941900|test1`94|1354574268279|test2`95|1354638563912|test3`96|1354644758848|test4`97|1354645526155|test5`98|1354725051316|test1`99|1354728602205|test6`100|1354731262190|test7`101|1354827506595|test8`102|1354906291376|test9`103|1355420090756|test10`104|1355860976101|test11`105|1355871301949|test12`106|1355873187514|test13`107|1355873434669|test14`108|1355876013804|test15`109|1355876507055|test99no`110|1355876733392|test16`111|1355939068132|test17`115|1355951742992|test18`116|1355965694602|test19`117|1355968209266|test20`118|1355968471078|test21`119|1355968861064|test22`120|1355969109587|test23`121|1355969450544|test24`122|1355969683618|test25`123|1356030886324|test26`124|1356036859810|test27`125|1356037791915|test28`126|1356038172458|test29`127|1356040666921|test30`128|1356115072590|test31`129|1356144314407|test32`165|1360859939436|Foil1`166|1360867928287|Foil2`194|1362788249977|ANNA5 test546`}Evans little thingy{112|1355944071932|FPGA1to3`113|1355945886508|FPGA3to5`114|1355947872834|FPGA5plus`164|1360605733467|Test1`167|1361209223972|FPGAcheck`168|1361297572405|NDA check`169|1361384083594|1_3kms at threshold 3`170|1361391901124|1_3kms at threshold 2`171|1361394846387|database test`172|1361399476301|1_3kms at threshold 2`173|1361400097188|test database error`174|1361402240795|1_3thres2_second`175|1361406242429|1_3thres1_5`176|1361465218455|3_5thres3`177|1361466469675|MCPtest`178|1361467305171|3_5thres3_second`179|1361469756270|3_5thres3_nomcp`180|1361483560648|5plusthres3`181|1361557433130|5plusthres2`182|1361567149399|5plusthres1_5`183|1361633260967|3_5thres2_nomcp`184|1361639750530|3_5thres1_5_nomcp`186|1362090150122|1_3thres3_nomcp`187|1362093527364|1_3thres2_nomcp`188|1362094994752|1_3thres1_5_nomcp`233|1369237649447|FPGAcheck_5plus_thres1_5`234|1369242965905|FPGAcheck_5plus_thres2`235|1369245345802|FPGAcheck_5plus_thres3`236|1369258862410|FPGAcheck_3_5_thres1_5`237|1369262187352|FPGAcheck_3_5_thres2`244|1369344194134|FPGAcheck_3_5_thres2`245|1369345846869|FPGAcheck_3_5_thres3`246|1369348300285|FPGAcheck_1_3_thres1_5`247|1369349310970|FPGAcheck_1_3_thres2`248|1369350101251|FPGAcheck_1_3_thres3`304|1375370530794|08_01_2013_masstest1`305|1375372551834|08_01_2013_masstest2`317|1378219975785|FPGA_masstest1_9_03_13`318|1378222125079|FPGA_masstest2_9_03_13`319|1378223179327|FPGA_masstest3_9_03_13`530|1401984924265|Testing Delay Trigger (Inital position)`531|1402006356571|Testing Delay Trigger (Inital position 2)`532|1402069659401|Testing Delay Trigger (Inital position 3)`533|1402073603402|Testing Delay Trigger (modified mult)`534|1402075309995|Testing Delay Trigger (modified beamlin measurements)`535|1402075970240|Testing Delay Trigger (modified beamlin measurements 2)`536|1402076346550|Testing Delay Trigger (playing around with divisor)`538|1403553004148|Delay Testing with delays output`539|1403559457391|Delay Testing with 0.5m delay`540|1403559826719|Delay Testing with 1.4m delay`541|1403560135382|Delay Testing with 1.5m delay`542|1403560360652|Delay Testing with 50m delay`543|1403891949645|Delay Testing (updated code)`544|1404234306082|Delay Testing 1-2 kms 0.945`545|1404236384643|Delay Testing 2-4 kms 0.945`546|1404237354012|Delay Testing 4-6 kms 0.945`547|1404237988742|Delay Testing 6-10 kms 0.945`548|1404238671277|Delay Testing 10+ kms 0.945`550|1404336410272|Delay Testing (fine tuing divisor)`551|1404339845563|Delay Testing 1-2 kms 093`552|1404341340851|Delay Testing 2-4 kms 093`553|1404341665626|Delay Testing 4-6 kms 093`554|1404341944936|Delay Testing 6-10 kms 093`555|1404342387492|Delay Testing 10+ kms 093`556|1404424356384|Testing New One Shot Mode`}Maintenance{130|1357145974437|Counter Testing`131|1357149510577|Counter Testing 2`132|1357150030152|Counter Testing 3`133|1357150480988|Counter Testing 4`134|1357150708758|Counter Testing 5`135|1357151087530|Counter Testing 6`136|1357151673351|Counter Testing 7`137|1357152013348|Counter Testing 8`138|1357153106752|Counter Testing 9`142|1358447643297|testing dust`195|1363203396199|Counter1`196|1363207832693|Counter2`197|1363208216846|Counter3`198|1363209389005|Focus1`199|1363211664302|Focus2`200|1363812044888|Counter_database1`201|1363812841521|Counter_database2`202|1363894076748|Counter_database3`203|1363895067167|Counter_database4`204|1363895921974|Counter_database5`205|1363896999698|Counter_database6`206|1364482410289|Source Testing1`207|1364488419864|Source Testing2`208|1364490275357|Source Testing3`212|1364493595938|Source Testing5`213|1367246475029|DCS Testing1`214|1367855782912|DCS Testing2`215|1367878364893|DCS Testing3`216|1367879176806|DCS Testing4`217|1367879993406|DCS Testing5`218|1367959784540|DCS Testing6`219|1368028542281|DCS Testing7`220|1368049130812|DCS Testing8`221|1368052951873|DCS Testing9`222|1368219672789|Program Testing 1`223|1368477578618|Program Testing 2`224|1369069797415|Aiming 01`225|1369085979597|Aiming 02`226|1369086342941|Aiming 03`227|1369148440606|Aiming 04`228|1369155665259|Aiming 05`229|1369158362144|Aiming 06`230|1369166392141|Aiming 07`231|1369170588662|Aiming 08`232|1369171161279|Aiming 09`238|1369326038912|Aiming 10`239|1369329749474|Aiming 11`240|1369334723786|Aiming 12`241|1369336371241|Aiming 13`242|1369340055237|Aiming 14`243|1369341682548|Aiming 15`249|1369416781590|Aiming 15`250|1369416888191|Aiming 16`251|1369419288881|Aiming 17`252|1369426105594|Aiming 18`253|1369426775796|Aiming 19`254|1369428457045|Aiming 20`255|1369429119488|Aiming 21`256|1369429450933|Aiming 22`257|1369429664403|Aiming 23`268|1370036419622|Query test`400|1385406561707|2013_11_25_test0`406|1386263120267|2013_12_05_test0`410|1389299137936|2014_01_09-small graphite test`411|1389634313837|2014_01_13-small graphite test`412|1389718238402|2014_01_14-small graphite test`485|1394492568067|2014_03_10_test0`507|1398178686154|2014_04_22_Mix3-1_test1`508|1398182165459|2014_04_22_Mix3-1_test2`526|1400086815884|2014_05_14_test0`560|1405437454463|2014_0715-Test0`561|1408396439261|2014_0818 - Test0`566|1409676607293|2014_09_02-DCS_I_Test`578|1411060150100|2014_09_18_DCS`581|1412116026579|FPGA Testing`620|1415031927488|2014_11_03_Batch_Processor_testing`622|1415650494135|2014_11_10_test0`623|1415660506968|2014_11_10_test1`624|1415991762683|2014_11_10_test1`625|1415995571824|2014_11_14_test1`626|1415996817471|2014_11_14_test2`636|1417029541215|2014_11_26_test0`637|1417112132612|2014_11_27_test0`638|1417195717188|2014_11_28_test0`639|1417198491583|2014_11_28_test1`640|1417380945782|2014_11_30_test0`641|1417469616540|2014_12_01_test0`642|1417471425280|2014_12_01_test1`643|1417626513761|2014_12_03_test0`644|1417628955048|2014_12_03_test1`645|1417632154080|2014_12_03_test2`646|1417632518923|2014_12_03_test3`647|1417885808793|2014_12_06_test0`648|1417886376709|2014_12_06_test1`649|1417886840907|2014_12_06_test2`650|1417978793410|2014_12_07_test0`651|1418048080797|2014_12_08_test0`654|1418921907093|2014_12_18_test1`655|1418933424585|2014_12_18_test2`656|1418952749170|2014_12_18_test3`663|1421028563489|2015_01_11`664|1421249440831|2015_01_14`665|1421272181969|2015_01_14_test1`683|1423063206208|2015_02_04_test1`686|1424014941546|2_15_2015_Mirror_pre_ND2_15_2015_Mirror_pre_NDA`701|1425934916817|DCS Testing March 9`702|1426007788554|Beam Allignment March 10`703|1426112438556|Beam Allignment March 11`727|1429048970200|Testing CAMAC and database 3rd detector`728|1429054334238|Testing CAMAC and database 3rd detector (2)`731|1429216335809|test1_4_16_2015`732|1429544649336|test1_4_20_2015`733|1429549552415|test2_4_20_2015`734|1429550869164|test3_4_20_2015`735|1429562102400|test4_4_20_2015`736|1429562721236|test5_4_20_2015`740|1430412719249|2015_0430 - test1`763|1433285557201|Mirror Test 6_02_2015`765|1433449373283|DAQ Iron 6_04_2015`766|1433531706077|DAQ Iron 6_05_2015`767|1433780082195|DAQ Iron 6_08_2015`768|1433974234145|Batch_testing_6_10_2015`770|1434403406334|Test_6_15_2015`772|1434639574892|Data_Test0_6_18_2015`773|1435009045279|Data_Test0_6_22_2015`774|1435165273470|2015_06_24_test0`775|1435597475590|2015_06_29_test0`776|1436200774816|2015_07_06_test0`777|1436204371575|2015_07_06_test1`778|1436978407014|2015_07_15_test1`791|1438448736370|Riley_Detector_Test`792|1438452079334|Riley_Detector_Test`803|1438956743163|8_7_2015 DCS Test`805|1439239925046|2015_08_09_test1`809|1440192467677|2015_8_21_Alignment`812|1440534107824|2015_8_25_test1`838|1441313919094|2015_9_03_Run0`846|1441723832191|2015_09_08_run1`847|1441726615208|2015_09_08_run2`848|1441807147490|2015_09_09_run1`849|1441828265095|2015_09_09_run2`850|1441904208977|2015_09_10_run1`851|1441907742000|2015_09_10_run2`852|1441910545911|2015_09_10_run3`853|1441914252008|2015_09_10_run4`854|1441925467375|2015_09_10_run5`855|1441981605699|2015_09_11_run1`856|1441985830448|2015_09_11_run2`857|1441990662728|2015_09_11_run3`858|1442008098330|2015_09_11_run4`859|1442239928306|2015_09_14_run1`860|1442244004165|2015_09_14_run2`861|1442249644910|2015_09_14_run3`862|1442254768028|2015_09_14_run4`863|1442261294172|2015_09_14_run5`864|1442265404953|2015_09_14_run6`865|1442326150688|2015_09_15_run1`866|1442330062533|2015_09_15_run2`867|1442340779980|2015_09_15_run3`868|1442348222034|2015_09_15_run4`869|1442354454808|2015_09_15_run5`870|1442356450916|2015_09_15_run6`871|1442411901532|2015_09_16_run1`872|1442417244702|2015_09_16_run2`873|1442419298688|2015_09_16_run3`874|1442421201881|2015_09_16_run4`875|1442423429745|2015_09_16_run5`876|1442426914689|2015_09_16_run6`877|1442431631161|2015_09_16_run7`878|1442434936106|2015_09_16_run8`879|1442442096773|2015_09_16_run9`880|1442503929839|2015_09_17_run1`881|1442509606487|2015_09_17_run2`882|1442513316198|2015_09_17_run3`883|1442514354263|2015_09_17_run4`884|1442522624844|2015_09_17_run5`885|1442522866768|2015_09_17_run`886|1442523048595|2015_09_17_run6`887|1442525752182|2015_09_17_run7`888|1442536139753|2015_09_17_run8`889|1442853892363|2015_09_20_run1`890|1442859147131|2015_09_20_run2`891|1442859612370|2015_09_20_run3`892|1442860162321|2015_09_20_run4`935|1446153602207|10_29_2015_DCS_New_Filter`943|1447180218151|11_10_2015_run_1`944|1449768644351|12_10_2015_run_1`946|1449877376456|12_11_2015_run_1`947|1451421589965|12_29_2015_test_0`948|1451427740154|12_29_2015_test_1`955|1453493635027|2015_01_22_TestingAlignment`956|1453748621682|2015_01_25_TestingAlignment2`960|1454265112713|2016_01_31_slow_tests`966|1455150194810|2016_02_10_light_test1`967|1455575452831|2016_02_10_light_test2`968|1455576800215|2016_02_10_light_test3`969|1455820169012|2016_02_18_DCS_FPGATest`973|1456173891755|2016_2_22_test0`974|1456176491188|2016_2_22_test1`975|1456178161765|2016_2_22_test2`976|1456179275373|2016_2_22_test3`977|1456181099681|2016_2_22_test4`1009|1456773058799|2016_2_29_test0`1010|1456777475151|2016_2_29_test1`1011|1456779920191|2016_2_29_test2`1012|1456780966854|2016_2_29_test3`1013|1456782026812|2016_2_29_test4`1014|1456784049151|2016_2_29_test5`1015|1456851425909|2016_3_1`1016|1456851588750|2016_03_01test1`1017|1456875778001|2016_03_01mirrorTest1`1018|1456937021614|2016_03_02MirrorTest1`1019|1456958113382|2016_03_02_SlowParticles`1020|1457129860574|2016_03_04_SlowParticles`1021|1457287632758|2016_03_06_SlowParticles`1022|1457291559458|2016_03_06_Wafer`1061|1458660275329|2016_03_22_Pre_acc`1085|1459438796673|2016_3_30_CPD_test0`1086|1459870400177|2016_4_5_Steerer_Test`1135|1462900955198|2016_5_10_test0`1175|1463698960137|2016_5_19_run_10`1201|1464817011005|2016_6_1`1207|1464890578969|2016_6_2_run_0`1305|1468965528550|2016_07_19_test0`1318|1470339594226|2016_08_04_test1`1369|1471973182087|2016_08_23_test0`1370|1472220830421|2016_08_26_test0`1395|1473955963512|2016_09_15_ConstExpRun0`1396|1473957917441|2016_09_15_ConstExpRun1`1397|1473981873621|2016_09_15_aniya_impact_test0`1398|1474059965255|2016_09_16_FPGAtest1`1401|1474645044445|2016_09_23_test0`1402|1474649446422|2016_09_23_test1`1407|1475878527103|2016_10_07_Mirror_test`1410|1476203871957|2016_11_08_mirror_2`1414|1477002683382|10_20_2016_test_0`1478|1479151165166|11_14_2016_test0`1510|1483031401024|12_29_2016_Carbon_NanaTube_IronMix`1511|1483043050723|12_29_2016_Carbon_NanaTube_IronMix_run2`1512|1483114464730|12_30_2016_Carbon_NanaTube_IronMix_run3`1513|1484688088463|1_17_2017_Iron`1514|1485811852014|1_30_2017_Iron`1564|1490888829455|3_30_2017_Run0`1575|1492536924804|4_18_2017_Run0`1576|1492544412823|4_18_2017_Run1`1577|1492545340023|4_18_2017_Run2`1578|1492545937502|4_18_2017_Run3`1579|1492546768655|4_18_2017_Run4`1580|1492547329886|4_18_2017_Run5`1581|1492547792168|4_18_2017_Run6`1582|1492549465098|4_18_2017_Run7`1583|1492550048056|4_18_2017_Run8`1584|1492550580547|4_18_2017_Run9`1585|1492551035542|4_18_2017_Run10`1586|1492704296895|4_20_2017_Run0`1587|1492706471631|4_20_2017_Run1`1588|1492707650835|4_20_2017_Run2`1589|1492708434611|4_20_2017_Run3`1590|1492709614148|4_20_2017_Run4`1591|1492712917471|4_20_2017_Run5`1592|1492714390305|4_20_2017_Run6`1593|1492715325067|4_20_2017_Run7`1594|1492716183403|4_20_2017_Run8`1595|1492717600761|4_20_2017_Run9`1596|1492719531712|4_20_2017_Run10`1597|1492720547345|4_20_2017_Run11`1598|1492721846156|4_20_2017_Run12`1599|1493222457266|4_26_2017_Run0`1623|1495819187068|5_26_2017_Run0`1642|1500313529019|2017_07_17_Run_0`1643|1500319972812|2017_07_17_Run_1`1644|1500401186213|2017_07_18_test1`1645|1500406875023|2017_07_18_test2`1646|1500410426443|2017_07_18_test3`1647|1500412989980|2017_07_18_test4`1648|1500415025264|2017_07_18_test5`1649|1500418069305|2017_07_18_test6`1650|1500475509858|2017_07_18_test0`1651|1500478302402|2017_07_18_test01`1652|1500482422312|2017_07_19_test2`1653|1500483627204|2017_07_19_test3`1654|1500484782848|2017_07_19_test4`1655|1500486189988|2017_07_19_test5`1656|1500491294184|2017_07_19_test6`1657|1500493780100|2017_07_19_test7`1658|1500495271127|2017_07_19_test8`1659|1500496554393|2017_07_19_test9`1660|1500497499625|2017_07_19_test10`1661|1500498615900|2017_07_19_test11`1662|1500499666811|2017_07_19_test02`1663|1500563640792|2017_07_20_test1`1664|1500569364765|2017_07_20_test2`1665|1500578478950|2017_07_20_test3`1666|1500998200159|2017_07_25_test0`1667|1501002574181|2017_07_25_test1`1668|1501005402089|2017_07_25_test2`1669|1501007421549|2017_07_25_test3`1670|1501011482007|2017_07_25_test4`1671|1502398213352|2017_08_10_test0`1676|1503608429908|2017_08_24_Run0`1704|1505768052598|2017_09_18_`1756|1509563031605|2017_11_1_run0`1857|1514917809467|2018_01_02_run0`1929|1518462533188|2018_02_12_run1`1959|1519317451929|2018_02_22_test0`1960|1519324842175|2018_02_22_test1`1961|1519329950191|2018_02_22_test2`1962|1519333863426|2018_02_22_test3`1963|1519671547918|2018_02_26_test0`1964|1519675366140|2018_02_26_test1`1965|1519749650631|2018_02_27_test0`1966|1519753976057|2018_02_27_test1`2022|1527270985634|2018_05_25_test0`2023|1527272938559|2018_05_25_test1`2024|1527273229780|2018_05_25_test2`2025|1527274116276|2018_05_25_test3`2026|1527274767068|2018_05_25_test4`2027|1527275953146|2018_05_25_test5`2028|1527276765228|2018_05_25_test6`2029|1527277398414|2018_05_25_test7`2030|1527278313369|2018_05_25_test8`2031|1527278857303|2018_05_25_test9`2032|1527279452026|2018_05_25_test10`2033|1527279876258|2018_05_25_test11`2034|1527280086703|2018_05_25_test12`2035|1527281081506|2018_05_25_test13`2036|1527615354325|2018_05_29_test0`2037|1527616611170|2018_05_29_test1`2038|1527617752436|2018_05_29_test2`2039|1527619637414|2018_05_29_test3`2040|1527621356547|2018_05_29_test4`2041|1527622138857|2018_05_29_test5`2042|1527622850495|2018_05_29_test6`2043|1527623682313|2018_05_29_test7`2044|1527624362223|2018_05_29_test8`2045|1527625062558|2018_05_29_test9`2046|1527625580576|2018_05_29_test10`2047|1527784073179|2018_05_31_test0`2048|1527789844223|2018_05_31_test1`2049|1527792416055|2018_05_31_test2`2050|1527794145270|2018_05_31_test3`2051|1527795192616|2018_05_31_test4`2052|1527797094910|2018_05_31_test5`2053|1527798111033|2018_05_31_test6`2054|1527798730856|2018_05_31_test7`2055|1527799749808|2018_05_31_test8`2056|1527862302627|2018_06_01_test0`2145|1531765302862|2018_07_16`2148|1532448695580|2018_07_24`2162|1533851613278|2018_08_9_alex`2185|1536088957631|2018_09_04_run0`2186|1536090100367|2018_09_04_run1`2191|1536257392562|2018_09_06_run0`2247|1542662932170|2018_11_19_run0`2248|1542663655326|2018_11_19_run1`2249|1542663860923|2018_11_19_run2`2250|1542664198857|2018_11_19_run3`2361|1553013885483|2019_03_19_run0`2362|1553018572090|2019_03_19_run1`2363|1553020220762|2019_03_19_run2`2368|1553881964099|2019_03_29_run0`2390|1555344825862|2019_04_15_run0`2394|1555431978302|2019_04_16_run0`2444|1557767340727|2019_05_13_run0`2445|1557872983492|2019_05_14_run0`2446|1557875098637|2019_05_14_run1`2447|1557929373228|2019_05_15_runA1`2451|1557960450810|2019_05_15_charge_test`2452|1557960841297|2019_05_15_charge_test2`2453|1558019827505|2019_05_16_charge_test3`2459|1558124030448|source problems`2492|1558549996212|2019_05_22_run0`2524|1558654349454|2019_05_23_run0`2538|1559245269256|2019_05_30_test0`2539|1559246320949|2019_05_30_test1`2540|1559668629693|2019_06_04_test0`2564|1561590072521|2019_06_26_run2`2568|1561993060296|2019_07_01_testing`}Neutral Gas{143|1359149327372|Setup Testing`144|1359151278463|Run1`145|1359157953586|Run2`146|1359395484659|Run3`147|1359410008410|Run4`148|1359411750175|Run4`149|1359411899950|Run4`150|1359481725574|Run5`151|1359486241588|Run6`152|1359497086951|Run7`153|1359565130147|Run8`154|1359655321294|Run9`155|1360002606243|Run10`156|1360012770971|Run11`157|1360020048138|Run12`158|1360087086547|Run13`159|1360168099439|Run14`160|1360181677261|Run15`161|1360188501583|Run16`162|1360259455725|Run17`163|1360278118980|Run18`191|1362588888068|ANNA3 MANANA`209|1364491803098|Source Testing4`210|1364492150535|Source Testing4`211|1364493438668|Source Testing5`562|1408554902871|2014_0820 - Initial`563|1409166097247|2014_0827 - Iron`564|1409249991598|2014_0828 -Testing`565|1409329723497|2014_0829 - Gold`601|1412971190105|2014_10_10_test`602|1413399547497|2014_10_15_gold`603|1413403289506|2014_10_15_align`604|1413577108038|2014_10_17_iron`605|1413582822995|2014_10_17_iron_control`606|1413585714841|2014_10_17_O2`607|1413587873832|2014_10_17_O`608|1413590074906|2014_10_17_Ti`609|1413591119381|2014_10_17_FeO`}STEREO{258|1369759830522|Test0`259|1369761633567|Test1`260|1369762722506|Test0_1`261|1369763303114|Test1`262|1369764160079|Test0_1`263|1369764471170|Test1`264|1369773738244|Test2`265|1369775218091|Test3`266|1369777143278|Test4`267|1369781517265|Test5`269|1370463157197|test0_2`270|1370464191145|test0_3`271|1370464999933|test0_4`272|1370465336852|test0_5`273|1370468878892|test0_6`274|1370549706872|newsetuptest1`275|1370552152132|newsetuptest1_1`276|1370552448332|06_06_test1`277|1370554190720|06_06_test2`278|1370559407081|06_06_test2_0`279|1370970511249|06_11_TEST1`280|1371154868086|06_13_TEST0`281|1371155541330|06_13_TEST1`282|1371158796490|06_13_TEST2`283|1371160890191|06_13_TEST3`284|1371162572299|06_13_TEST4`285|1371229618145|06_14_TEST0`286|1371490646207|06_17_TEST0`287|1371506980562|06_17_TEST1`288|1371596329372|06_18_TEST0`289|1371686426959|06_19_TEST0`290|1371745380752|06_20_TEST0`291|1371759845826|06_20_TEST1`292|1371833194953|06_21_TEST0`293|1371853942185|06_21_TEST1`294|1372347369678|06_27_TEST0`295|1372355323579|06_27_TEST1`296|1372436243866|06_28_TEST1`297|1372439599534|06_28_TEST0`298|1373928552424|07_15_TEST0`299|1374002951905|07_16_TEST0`300|1374079841308|07_17_TEST0`301|1374102023454|07_17_TEST1_ionon`302|1374103278184|07_17_TEST1_ionoff`303|1374264097296|07_19_TEST0`306|1375384387881|08_01_2013_TEST0`307|1377027809824|08_20_2013_TEST0`308|1377098473042|08_20_2013_TEST1`309|1377113925609|08_20_2013_TEST2`310|1377271377433|08_23_2013_TEST0`311|1377545325412|08_23_2013_TEST0`349|1382369309729|2013_10_21_test0`350|1382373967629|2013_10_21_test1`351|1382629906710|2013_10_24_test0`352|1382636503727|2013_10_24_test1`353|1382642621582|2013_10_24_test2`354|1382642752376|2013_10_24_test3`355|1382722884019|2013_10_25_test`356|1382732845177|2013_10_25_run_1_2`357|1382734374430|2013_10_25_run_2_5`358|1382734870012|2013_10_25_run_5_10`359|1382738001028|2013_10_25_run_10+`360|1382970944413|2013_10_28_test1`361|1382971262586|2013_10_28_10_plus_2`362|1383058042976|2013_10_29_silver_normal`363|1383063978433|2013_10_29_silver_angle_test1`364|1383064362364|2013_10_29_silver_angle_60`365|1383079474556|2013_10_29_silver_angle_40`366|1383145276987|2013_10_30_silver_angle_20`367|1383162219022|2013_10_30_mli_test`368|1383162753538|2013_10_30_mli_2_5`369|1383163912515|2013_10_30_mli_test1`370|1383164177175|2013_10_30_mli_5_10`371|1383168157381|2013_10_30_mli_hispeed_test`372|1383168746915|2013_10_30_mli_10_plus`373|1383249115599|2013_10_30_mli_angle_60`374|1383251886950|2013_10_30_mli_angle_40`375|1383254154493|2013_10_30_mli_angle_20`376|1383315934147|2013_10_31_BeCu_test`377|1383316402785|2013_10_31_becu_2_5`378|1383317357138|2013_10_31_becu_5_10`379|1383321105942|2013_10_31_becu_10_plus`380|1383578728175|2013_11_5_kapton_test`381|1383579350015|2013_11_5_kapton_2_5`382|1383580018092|2013_11_5_kapton_5_10`383|1383582818642|2013_11_5_kapton_10_plus`384|1383666193966|2013_11_5_solarcell_test`385|1383666675751|2013_11_5_solarcell_2_5`386|1383667810090|2013_11_5_solarcell_5_10`387|1383671504902|2013_11_5_solarcell_10_plus`388|1383753532638|2013_11_6_energy_tests`389|1383756663385|2013_11_6_energy_10V`390|1383762317524|2013_11_6_energy_5V`391|1383771831214|2013_11_6_energy_1V`392|1383777926358|2013_11_6_energy_0.5V`393|1383842184670|2013_11_6_energy_2V`394|1383855805980|2013_11_6_energy_0.25V`395|1383862609473|2013_11_6_energy_1V_B`396|1383866941815|2013_11_6_energy_5V_B`469|1393260443828|2014_02_24-test`470|1393261370451|2014_02_24-MLI-2-5-test`471|1393263617156|2014_02_24-MLI-2-5`472|1393265956620|2014_02_24-MLI-5-10`473|1393272496716|2014_02_24-MLI-10-plus`474|1393359981659|2014_02_24-MLI-angle-0`475|1393361706520|2014_02_24-MLI-angle-20`476|1393363434681|2014_02_24-MLI-angle-40-broken`477|1393364976043|2014_02_24-MLI-angle-40`478|1393366803691|2014_02_24-MLI-angle-60`479|1393433075050|2014_02_24-kapton-angle-0`480|1393437278549|2014_02_24-kapton-angle-20`481|1393445686927|2014_02_24-kapton-angle-40`482|1393448028260|2014_02_24-kapton-angle-60`483|1393543542663|2014_02_24-antenna-test-1`484|1393608247730|2014_02_24-antenna-test-2`496|1397502088746|2014_4_14_grounded`497|1397577564932|2014_4_14_bias_pos_10`498|1397588594018|2014_4_14_bias_neg_10`499|1397662153865|2014_4_14_bias_pos_2`500|1397680624068|2014_4_14_bias_neg_2`518|1398808099960|2014_04_29_grid_minus_50`612|1413839129338|2014_10_20_test`613|1414434999334|2014_10_27_run1`614|1414436681385|2014_10_27_run2`615|1414437795645|2014_10_27_run3`616|1414438013448|2014_10_27_allruns`617|1414603342254|2014_10_29_allruns`618|1414685087926|2014_10_30_allruns`619|1414769367327|2014_10_31_allruns`621|1415294094671|2014_11_06_reverse`660|1420566116398|Georg_1_6`661|1420739149768|Georg_1_8`662|1420819252588|Georg_1_9`725|1428338441851|tests_4_6_15`779|1437426021106|2015_07_20_tests`780|1437431680913|2015_07_20_tests2`781|1437435289080|2015_07_20_tests3`782|1437495836570|2015_07_20_tests4`783|1437496762213|2015_07_20_mli`784|1437675031562|2015_07_23_mli2`785|1437682088636|2015_07_23_mli`893|1442861481097|2015_09_21_test`928|1445459979271|10_21_2015_test`1134|1462899673005|2016_5_10_run0`1136|1462908745727|2016_5_10_test1`1137|1462909516911|2016_5_10_test2`1138|1462912636845|2016_5_10_test3`1139|1462913697799|2016_5_10_test4`1140|1462916520861|2016_5_10_test5`1141|1462918453788|2016_5_10_test6`1142|1462983315045|2016_5_11_run0`1143|1462985915549|2016_5_11_run1`1144|1462988890680|2016_5_11_run2`1145|1462991611167|2016_5_11_run3`1146|1462995533593|2016_5_11_run4`1147|1463162019850|2016_5_13_run0`1148|1463164808583|2016_5_13_run1`1149|1463426661872|2016_5_16_run0`1150|1463430585257|2016_5_16_run1`1151|1463502438142|2016_5_17_run 0`1152|1463518834124|2016_5_17_run 1`1153|1463521737499|2016_5_17_run 2`1154|1463524545795|2016_5_17_run 3`1155|1463526081736|2016_5_17_run 4`1156|1463583820196|2016_5_18_run 0`1157|1463586769102|2016_5_18_run 1`1158|1463599844752|2016_5_18_run 2`1159|1463603402777|2016_5_18_run 3`1160|1463606265606|2016_5_18_run 4`1161|1463608070155|2016_5_18_run 5`1162|1463609833171|2016_5_18_run 6`1163|1463610393295|2016_5_18_run 7`1164|1463611320956|2016_5_18_run 8`1165|1463687599555|2016_5_19_run_0`1166|1463688538085|2016_5_19_run_1`1167|1463689782066|2016_5_19_run_2`1168|1463690974670|2016_5_19_run_3`1169|1463692871933|2016_5_19_run_4`1170|1463693918145|2016_5_19_run_5`1171|1463695268125|2016_5_19_run_6`1172|1463696260754|2016_5_19_run_7`1173|1463697253941|2016_5_19_run_8`1174|1463698391234|2016_5_19_run_9`1176|1463768762941|2016_5_20_run_0`1177|1463771243036|2016_5_20_run_1`1178|1463772672830|2016_5_20_run_2`1179|1463774143123|2016_5_20_run_3`1180|1463775146158|2016_5_20_run_4`1181|1463776404748|2016_5_20_run_5`1182|1463778155684|2016_5_20_run_6`1183|1463779421311|2016_5_20_run_7`1184|1463780910896|2016_5_20_run_8`1185|1463782626756|2016_5_20_run_9`1186|1463783862588|2016_5_20_run_10`1187|1463784728176|2016_5_20_run_11`1188|1464108577099|2016_5_24_run_0`1189|1464112112245|2016_5_24_run_1`1190|1464116181643|2016_5_24_run_2`1191|1464121423844|2016_5_24_run_3`1192|1464125572377|2016_5_24_run_4`1193|1464129698321|2016_5_24_run_5`1194|1464297624133|2016_5_26_run_0`1195|1464362402835|2016_5_27_run_0`1196|1464372708606|2016_5_27_run1`1197|1464378170981|2016_5_27_run2`1198|1464382283778|2016_5_27_run3`1199|1464385296440|2016_5_27_run4`1200|1464388911461|2016_5_27_run5`}Eric Christian{312|1377617872196|Aiming Test`313|1377789613489|Sample 2`314|1377795249711|Sample 1`315|1377803713832|Sample 3`316|1377875500700|Sample 3_2`592|1412782552190|2014_10_08_pre_test`593|1412788869057|2014_10_08_test1`594|1412792215674|2014_10_08_test2`595|1412797834764|2014_10_08_test3`596|1412800893465|2014_10_08_test4`597|1412802988055|2014_10_08_test5`598|1412868212349|2014_10_09_test1`599|1412870344362|2014_10_09_test2`600|1412873772538|2014_10_09_test3`}Solar Cell{320|1379426002245|2013_09_17_test1`}LDEX{321|1379959877155|2013_09_23_test1`322|1380127002836|2013_09_25_test1`323|1380131385841|2013_09_25_test2`324|1380140753844|2013_09_25_test0`325|1380554282569|2013_09_30_test`326|1380569224638|2013_09_30_test1`327|1380572269337|2013_09_30_test3`328|1380573080182|2013_09_30_test4`329|1380575727685|2013_09_30_test5`330|1380637339279|2013_10_01_test1`331|1380650188247|2013_10_01_test2`332|1380723689671|2013_10_02_test1`333|1380726650606|2013_10_02_test2`334|1380728111358|2013_10_02_test3`335|1380745385355|2013_10_02_test4`336|1380809896388|2013_10_03_test1`337|1380812704015|2013_10_03_test2`338|1380896719238|2013_10_04_test`339|1380896806977|2013_10_04_test1`340|1380902776947|2013_10_04_test2`341|1380908903798|2013_10_04_test3`413|1390238400054|2014_01_20 test0`414|1390242439748|2014_01_20_test1`415|1390322107639|2014_01_21_test3`416|1390328314558|2014_01_21_test4`417|1390345649131|2014_01_21_test5`418|1390492635063|2014_01_23_test1`419|1390509271693|2014_01_23_test2`420|1390578953917|2014_01_24_test1`421|1390581320320|2014_01_24_test2`422|1390584341491|2014_01_24_test3`423|1390588084520|2014_01_24_test4`424|1390839244730|2014_01_27_test1`425|1390843631582|2014_01_27_test2`426|1390845733402|2014_01_27_test3`427|1390853845003|2014_01_27_test4`428|1390855284152|2014_01_27_test5`429|1390923721505|2014_01_28_test1`430|1390929198936|2014_01_28_test2`431|1390940860822|2014_01_28_test3`432|1390944289053|2014_01_28_test4`433|1390947593397|2014_01_28_test5`434|1391095454062|2014_01_30_test1`435|1391098808598|2014_01_30_test2`436|1391106767436|2014_01_30_test3`437|1391122731843|2014_01_30_test4`438|1391445515889|2014_02_03_test1`439|1391452289261|2014_02_03_test2`440|1391458448590|2014_02_03_test3`441|1391461517447|2014_02_03_test4`442|1391466383375|2014_02_03_test5`443|1391469342831|2014_02_03_test6`444|1391530898282|2014_02_04_test1`445|1391535294825|2014_02_04_test2`446|1391539554045|2014_02_04_test3`447|1391555438336|2014_02_04_test4`448|1391558246419|2014_02_04_test5`449|1391615074256|2014_02_05_test1`450|1391617907954|2014_02_05_test2`451|1391620422443|2014_02_05_test3`452|1391623487055|2014_02_05_test4`453|1391626782955|2014_02_05_test5`454|1391638892548|2014_02_05_test6`455|1391641316388|2014_02_05_test7`456|1391704800761|2014_02_06_test1`457|1391706500017|2014_02_06_test2`458|1391709425568|2014_02_06_test3`459|1391712489902|2014_02_06_test4`460|1391724104836|2014_02_06_test4`461|1391724195338|2014_02_06_test5`462|1391726560232|2014_02_06_test6`463|1391785977094|2014_02_07_test1`464|1391788198696|2014_02_07_test2`465|1391789812697|2014_02_07_test3`519|1399492127261|2014_05_07_test1`520|1399500885923|2014_05_07_test2`521|1399656657690|2014_05_09_test1`522|1399670015629|2014_05_09_test2`523|1399915372876|2014_05_12_test1`524|1399929313193|2014_05_12_test2`525|1400013912817|2014_05_13_test1`557|1404589105296|test0`558|1404743676435|test0`559|1404833204910|test0`}Mehoke Foils{397|1384214819661|2013_11_11_test0`398|1384268757108|2013_11_12_test0`399|1384440555822|2013_11_14_test1`466|1392074469237|2014_02_10-Pointing test`467|1392842587396|2014_02_19-Foil A`468|1392936011565|2014_02_20-Foil A 2`}Ejecta Experiments 2014{495|1397247607500|2014_4_11_testing`509|1398184283647|2014_04_22_initial`510|1398186141100|2014_04_22_initial_1500`511|1398186495383|2014_04_22_initial_2500_2`512|1398270625858|2014_04_22_grids_test`513|1398354982054|2014_04_22_grid_window`514|1398368003731|2014_04_22_grid_window_2`515|1398439600446|2014_04_22_angle_22_5`516|1398459993655|2014_04_22_angle_45_closer`517|1398785509153|2014_04_22_angle_45_closer_window`}ODINSun{501|1397745104933|2014_4_17_test1`502|1397750441848|2014_4_17_test2`503|1397753795053|2014_4_17_test3`504|1397754652973|2014_4_17_test4`505|1397770088324|2014_4_17_test5`506|1397771150370|2014_4_17_test6`}HyperSuda{527|1401308553750|2014_05_28_test0`528|1401369947318|2014_05_29_test0`529|1401854643753|2014_06_03_testrun`549|1404245445252|Testing Mass Spectra with Darren`610|1413729877426|2014_10_19_test1`611|1413737391066|2014_10_19_test2`692|1424803067999|2015_02_24-Test0`693|1424876228832|2015_02_25-Test0`694|1425055136250|2015_02_27-Test0`760|1432846817427|test0_suda_5_24_2015`761|1432926565269|test1_5_29_2015`762|1433169440791|test1_6_01_2015`764|1433344977301|SUDA Iron 6_03_2015`940|1446585981253|11_03_2015_run1`941|1446831042077|11_06_2015_run1`942|1446836417430|11_06_2015_run2`970|1455899842948|2016_2_19_test0`971|1455916102436|2016_2_19_test1`972|1455926544674|2016_2_19_test2`}Todd Bradley Florida Group{537|1403017709394|Labradorite test 1`}Zoltan Dust Detectors{567|1410277374050|2014_09_09-Piezo_test1`568|1410278843152|2014_09_09-Piezo_test2`569|1410279058323|2014_09_09-Piezo_test3`570|1410279992099|2014_09_09-pvdf_loop_test1`571|1410280999086|2014_09_09-pvdf_loop_test2`572|1410448785565|2014_09_11_piezo_test1`573|1410451249334|2014_09_11_pvdf_test1`574|1410453604535|2014_09_11_pvdf2_test1`575|1410464900037|2014_09_11_pvdf2_test2`576|1410880982725|2014_09_16-pvdf1_test1`577|1410883364670|2014_09_16-pvdf1_test2`1492|1479847102520|11_22_2016_test0`1493|1479851279726|11_22_2016_test1`1494|1480437097514|11_29_2016_test0`1495|1480441559122|11_29_2016_test1_p50v_3kmsAbove`1496|1480444728948|11_29_2016_test2_p50v_8kmsAbove`1497|1480457617186|11_29_2016_test3_p50v_15kmsAbove`1498|1480459479919|11_29_2016_test4_N50v_1kmsAbove`1499|1480460863377|11_29_2016_test5_N50v_3kmsAbove`1500|1480461726254|11_29_2016_test6_N50v_8kmsAbove`1501|1480462976198|11_29_2016_test7_N50v_15kmsAbove`1502|1480541839574|11_30_2016_test8_N50v_1kmsAbove`1503|1480543796874|11_30_2016_test9_N50v_3kmsAbove`1504|1480544724746|11_30_2016_test10_N50v_8kmsAbove`1505|1480545955433|11_30_2016_test11_N50v_15kmsAbove`1506|1480546337071|11_30_2016_test12_P50v_1kmsAbove`1507|1480547643402|11_30_2016_test13_P50v_3kmsAbove`1508|1480548090772|11_30_2016_test14_P50v_8kmsAbove`1509|1480548511168|11_30_2016_test15_P50v_15kmsAbove`}Ablation Exp{579|1412103065751|First run`580|1412111574909|Testing Impact`582|1412190287266|Image Charge testing`583|1412264919202|2014_10_02_Image_Charge_setup`587|1412358032777|2014_10_03_Gas_test4`588|1412364889232|2014_10_03_Gas_test5`589|1412370360388|2014_10_03_Gas_test6`590|1412372448687|2014_10_03_Gas_test7`591|1412375318996|2014_10_03_Gas_test8`894|1443561508926|2015_09_29_impact_run1`949|1451593686248|2015_12_31_AbExp6_run1`950|1452019499879|2015_01_05_PrelimTests`951|1452027879671|2015_01_05_AbExp6_run1`952|1452107115387|2015_01_06_AbExp6_run2`953|1452191713012|2015_01_07_AbExp6_run3`954|1452287144334|2015_01_08_AbExp6_run4`957|1453751016924|2016_01_25_AbExp6_Run5`958|1453834139288|2016_01_26_AbExp6_Run6`959|1454101274254|2016_01_29_AbExp6_Run7`961|1454352345910|2016_02_01_Ab6Run8`962|1454523635726|2016_02_03_Ab6Run9`963|1454607099148|2016_02_04_Ab6Run10`964|1454691678360|2016_02_05_Ab6Run11`965|1454955639161|2016_02_08_Ab6Run12`1208|1465238553238|2016_06_06_Ab7Run1`1209|1465241067365|2016_06_06_AlignmentTest1`1210|1465244269537|2016_06_06_Run2`1211|1465331038901|2016_06_07_Ab7Run3`1212|1465489482245|2016_06_09_Ab7Run4`1213|1465499455549|2016_06_09_Ab7Run5`1214|1465506289091|2016_06_09_Ab7Run6`1215|1465576973185|2016_06_10_Ab7Run7`1216|1465849178776|2016_06_13_Ab7Run8`1217|1466093340414|2016_06_16_Ab7Run9`1218|1466103606825|2016_06_16_Ab7Run10`1219|1466107591174|2016_06_16_Ab7Run11`1220|1466176816784|2016_06_17_Ab7Run12`1221|1466182144527|2016_06_17_Ab7Run12`1222|1466182427602|2016_06_17_Ab7Run13`1228|1467226789507|2016_06_29_Ab8Run1`1229|1467233678604|2016_06_29_Ab8Run2`1230|1467238214452|2016_06_29_Ab8Run3`1231|1467304012438|2016_06_30_Ab8Run4`1232|1467330210070|2016_06_30_Ab8Run5`1233|1467336685730|2016_06_30_Ab8Run6`1234|1467387148183|2016_07_1_Ab8Run7`1235|1467391486230|2016_07_1_Ab8Run8`1307|1469564122362|2016_07_26_Run1`1308|1469633708183|2016_07_27_Ab9Run2`1309|1469818183176|2016_07_29_Ab9Run3`1310|1469908607147|2016_07_30_Ab9Run4`1311|1470070273723|2016_08_01_Ab9Run5`1312|1470087231474|2016_08_01_Ab9Run6`1313|1470156687979|2016_08_02_Ab9Run7`1314|1470162132269|2016_08_02_Ab9Run8`1315|1470176969061|2016_08_02_Ab7Run14`1316|1470245439864|2016_08_03_Ab7Run15`1317|1470266146063|2016_08_03_Ab7Run16`1371|1472589085445|2016_08_30_AbExp9Run1`1372|1472662655825|2016_08_31_AbExp9Run2`1373|1472667860832|2016_08_31_AbExp9Run3`1374|1472677361187|2016_08_31_AbExp9Run4`1375|1472747328479|2016_08_31_AbExp10Run5`1376|1472754783033|2016_09_31_AbExp10Run6`1377|1472769212870|2016_09_1_AbExp10Run7`1378|1473353426046|2016_09_08_AbExp10Run8`1379|1473364014741|2016_09_08_AbExp10Run9`1380|1473365577736|2016_09_08_AbExp10Run10`1381|1473368724940|2016_09_08_AbExp10Run11`1382|1473370567606|2016_09_08_AbExp10Run12`1383|1473373497614|2016_09_08_AbExp10Run13`1384|1473447280577|2016_09_09_AbExp10Run14`1385|1473449292421|2016_09_09_AbExp10Run15`1386|1473452295206|2016_09_09_AbExp10Run16`1387|1473713310686|2016_09_12_AbExp10Run17`1388|1473781365384|2016_09_13_AbExp10Run18`1389|1473786234090|2016_09_13_AbExp10Run19`1390|1473796283184|2016_09_13_AbExp10Run20`1391|1473803177719|2016_09_13_AbExp10Run21`1392|1473805872013|2016_09_13_AbExp10Run22`1393|1473872889180|2016_09_14_AbExp10Run23`1394|1473884014526|2016_09_14_AbExp10Run24`1525|1487286890711|2_16_2017_AbExp11_Run1`1526|1487352351608|2_17_2017_AbExp11_Run2`1527|1487358396875|2_17_2017_AbExp11_Run3`1528|1487362354475|2_17_2017_AbExp11_Run4`1529|1487364208654|2_17_2017_AbExp11_Run5`1530|1487368708540|2_17_2017_AbExp11_Run6`1531|1487616733063|2_20_2017_AbExp11_Run7`1532|1487703708718|2_21_2017_AbExp11_Run8`1533|1487791354130|2_22_2017_AbExp11_Run9`1534|1487873233422|2_23_2017_AbExp11_Run10`1535|1487960965740|2_24_2017_AbExp11_Run11`1536|1487976563506|2_24_2017_AbExp11_Run12`1537|1488218408728|2_27_2017_AbExp11_Run13`1538|1488230484023|2_27_2017_AbExp11_Run14`1539|1488303826437|2_28_2017_AbExp11_Run15`1540|1488314248749|2_28_2017_AbExp11_Run16`1541|1488656380024|3_04_2017_AbExp12_Run1`1542|1488908191052|3_07_2017_AbExp12_Run2`1543|1488922528641|3_07_2017_AbExp12_Run3`1544|1488937891352|3_07_2017_AbExp12_Run4`1545|1488994275114|3_08_2017_AbExp12_Run5`1546|1489017465985|3_08_2017_AbExp12_Run6`1547|1489024278955|3_08_2017_AbExp12_Run7`1912|1517334275522|2018_01_30_exp13_run1`1913|1517353829660|2018_01_30_exp13_run2`1914|1517418178709|2018_01_30_exp13_run3`1915|1517422081390|2018_01_30_exp13_run4`1916|1517431074961|2018_01_30_exp13_run5`1917|1517436629462|2018_01_30_exp13_run6`1918|1517439039588|2018_01_30_exp13_run7`1919|1517444426762|2018_01_30_exp13_run8`1920|1517502400313|2018_01_30_exp13_run9`1921|1517509182433|2018_01_30_exp13_run10`1922|1517854107468|2018_02_05_exp13_run11`1923|1517861842738|2018_02_05_exp13_run12`1924|1517936086325|2018_02_06_exp13_run13`1925|1517957266744|2018_02_06_exp13_run14`1926|1518023140794|2018_02_07_exp13_run15`1927|1518035311188|2018_02_07_exp13_run16`1928|1518112349721|2018_02_08_exp13_run17`}Ablation Exp 2{584|1412271419350|2014_10_02_Gas_test1`585|1412281055180|2014_10_02_Gas_test2`586|1412284978144|2014_10_02_Gas_test3`}PVDF{635|1416772171377|2014_11_23_test0`657|1419185357548|2014_12_21_test0`658|1419265951852|2014_12_22_test0`659|1419354448096|2014_12_23_test0`699|1425862499909|Test run`700|1425916820454|Test run 2`737|1429635730039|test0_4_21_2015`738|1429802910173|test0_4_23_2015`739|1429990410422|test0_4_25_2015`769|1434395310728|Test0_6_15_2015`771|1434473511653|Test0_6_16_2015`1851|1513632770345|2017_12_18_run0`1930|1518472962031|2018_02_12_test1`1931|1518539375027|2018_02_13_test1`1932|1518556123702|2018_02_13_test3`1991|1523379793961|2018_04_10_test0`1992|1523389870459|2018_04_10_test1`1993|1523393033435|2018_04_10_test2`1994|1523395363159|2018_04_10_test3`1995|1523464913979|2018_04_11_test4`1996|1523468438522|2018_04_11_test5`1997|1523477196410|2018_04_11_test6`1998|1523478631345|2018_04_11_test7`1999|1523480341673|2018_04_11_test8`2000|1523551575330|2018_04_12_test9`2001|1523554257554|2018_04_12_test10`2002|1523555727049|2018_04_12_test11`2397|1555528631321|2019_04_17_run0`2398|1555949427232|2019_04_22_run0`2399|1555954524725|2019_04_22_run1`2400|1555957180727|2019_04_22_run2`}Ice Target{652|1418337491310|2014_12_11_test`653|1418421239768|2014_12_12_test1`811|1440527421063|2015_8_25_Run1`813|1440542104301|2015_8_25_Run2`814|1440609195989|2015_8_26_Run1`815|1440624012435|2015_8_26_Run2`816|1440698949339|2015_8_27_Run1`817|1440700382936|2015_8_27_Run2`818|1440705633733|2015_8_27_Run3`819|1440707474407|2015_8_27_Run4`820|1440781834985|2015_8_28_Run1`821|1440784652277|2015_8_28_Run2`822|1440786564057|2015_8_28_Run3`823|1440793558608|2015_8_28_Run4`824|1441130778728|2015_9_01_Run1`825|1441134694991|2015_9_01_Run2`826|1441136853821|2015_9_01_Run3`827|1441214583641|2015_9_02_Run1`828|1441215928915|2015_9_02_Run2`829|1441217033356|2015_9_02_Run3`830|1441219829845|2015_9_02_Run4`831|1441301061560|2015_9_03_Run1`832|1441302250920|2015_9_03_Run2`833|1441306343065|2015_9_03_Run3`834|1441311793131|2015_9_03_Run4`835|1441312489578|2015_9_03_Run5`836|1441312842705|2015_9_03_Run6`837|1441313474667|2015_9_03_Run7`839|1441389137441|2015_9_04_Run1`840|1441390332513|2015_9_04_Run2`841|1441390884265|2015_9_04_Run3`842|1441391430420|2015_9_04_Run4`843|1441391894892|2015_9_04_Run5`844|1441392123145|2015_9_04_Run6`845|1441392430381|2015_9_04_Run7`895|1444152529115|2015_10_6_test0`896|1444163372297|2015_10_6_test1`897|1444237311865|2015_10_7_run1`898|1444238632089|2015_10_7_run2`899|1444240047903|2015_10_7_run3`900|1444242071385|2015_10_7_run4`901|1444252041770|2015_10_7_run6`902|1444328040979|2015_10_8run1`903|1444331964748|2015_10_08_2015_10_8run2`904|1444407824472|10_09_2015_Run1`905|1444413708307|10_09_2015_Run2`906|1444414205369|10_09_2015_Run3`907|1444414950912|10_09_2015_Run4`908|1444416144556|10_09_2015_Run5`909|1444416396148|10_09_2015_Run6`910|1444417051532|10_09_2015_Run7`911|1444417444719|10_09_2015_Run8`912|1444418165518|10_09_2015_Run9`913|1444418785577|10_09_2015_Run10`914|1444682642320|10_12_2015_Run1`915|1444689979921|10_12_2015_Run2`916|1444743792110|10_13_2015_Run1`917|1444757709600|10_13_2015_DCS`918|1444758475171|10_13_2015_run_1`919|1444771184841|10_13_2015_run_2`920|1444772449620|10_13_2015_run_3`924|1445348607308|10_20_2015_run_1`925|1445369410558|10_20_2015_run_2`927|1445438165426|10_21_2015_Run_1`929|1446053149874|10_28_2015_run1`930|1446057607692|10_28_2015_run2`931|1446062278155|10_28_2015_run3`932|1446140214700|10_29_2015_run1`933|1446144400195|10_29_2015_run2`934|1446147574798|10_29_2015_run3`936|1446224717016|10_30_2015_run1`937|1446227539849|10_30_2015_run2`938|1446229378924|10_30_2015_run3`939|1446238828447|10_30_2015_run4`945|1449787380934|12_10_2015_run_one`1024|1457726475936|2016_03_11_2016_test0`1025|1457983982207|2016_03_11_2016_test1`1026|1457993137601|2016_03_11_2016_test2`1027|1457993734941|2016_03_11_2016_test3`1028|1458058637579|2016_03_15_test1`1029|1458062894614|2016_03_15_test2`1030|1458064206782|2016_03_15_test3`1031|1458065127981|2016_03_15_test4`1032|1458065945720|2016_03_15_test5`1033|1458072187548|2016_03_15_test6`1034|1458073810487|2016_03_15_test7`1035|1458075146446|2016_03_15_test8`1036|1458076273975|2016_03_15_test9`1037|1458077393218|2016_03_15_test10`1038|1458079128176|2016_03_15_test11`1039|1458079734795|2016_03_15_test12`1040|1458080908419|2016_03_15_test13`1041|1458148013746|2016_03_16_test1`1042|1458150134089|2016_03_16_test2`1043|1458151251835|2016_03_16_test3`1044|1458152664662|2016_03_16_test4`1045|1458153278382|2016_03_16_test5`1046|1458154675856|2016_03_16_test6`1047|1458156639098|2016_03_16_test7`1048|1458234673129|2016_03_17_test0`1049|1458236495722|2016_03_17_test1`1050|1458237733617|2016_03_17_test2`1051|1458244612616|2016_03_17_test3`1052|1458245976361|2016_03_17_test4`1053|1458248741220|2016_03_17_test5`1054|1458249912089|2016_03_17_test6`1055|1458250733404|2016_03_17_test7`1056|1458252061738|2016_03_17_test8`1087|1460142183389|2016_4_8_Steerer_Test_Run1`1088|1460143498053|2016_4_8_Steerer_Test_Run2`1089|1460145055880|2016_4_8_Steerer_Test_Run3`1090|1460146380887|2016_4_8_Steerer_Test_Run4`1091|1460148876112|2016_4_8_Steerer_Test_Run5`1092|1460151563493|2016_4_8_Steerer_Test_Run6`1093|1460155952172|2016_4_8_Steerer_Test_Run7`1094|1460665170027|2016_4_14_Steerer_Test_Run1`1095|1460668071034|2016_4_14_Steerer_Test_Run2`1096|1460669534138|2016_4_14_Steerer_Test_Run3`1097|1460670872139|2016_4_14_Steerer_Test_Run4`1098|1460749244584|2016_4_15_Steerer_Test_Run1`1099|1460751171123|2016_4_15_Steerer_Test_Run2`1100|1460752787506|2016_4_15_Steerer_Test_Run3`1101|1460753910578|2016_4_15_Steerer_Test_Run4`1102|1460755184300|2016_4_15_Steerer_Test_Run5`1103|1460756317005|2016_4_15_Steerer_Test_Run6`1104|1460756832697|2016_4_15_Steerer_Test_Run7`1105|1460757391088|2016_4_15_Steerer_Test_Run8`1106|1460758050985|2016_4_15_Steerer_Test_Run9`1107|1460758593033|2016_4_15_Steerer_Test_Run10`1128|1461270475168|2016_4_21_run1`1129|1461271973837|2016_4_21_run2`1130|1461273106398|2016_4_21_run3`1131|1461274067596|2016_4_21_run4`1132|1461275086406|2016_4_21_run5`1133|1461878536718|2016_5_05_run0`1202|1464881529309|2016_06_02_2016_6_2`1203|1464883680004|2016_6_2_run_1`1204|1464885379806|2016_6_2_run_2`1205|1464887640067|2016_6_2_run_3`1206|1464888861889|2016_6_2_run_4`1319|1470432660690|2016_08_05_test1`1320|1470775399214|2016_08_09_test1`1321|1470845985726|2016_08_10_test0`1322|1470929971070|2016_08_11_test0`1399|1474574830920|2016_09_22_test0`1400|1474577428285|2016_09_22_test1`1403|1475162668898|2016_09_29_test0`1404|1475183905814|2016_09_29_test1`1405|1475601047628|2016_10_04_test0`1406|1475857731475|2016_10_07_test0`1412|1476742092566|10_17_2016_Test_0`1413|1476812718362|10_18_2016_Test_0`1515|1485888991645|1_31_2017_New_Target_Silver_Foil`1516|1485893350731|1_31_2017_New_Target_Steering_tests`1517|1485893837610|1_31_2017_New_Target_Steering_tests2`1518|1485973217535|2_1_2017_New_Target_Steering_tests3`1519|1486144924413|2_3_2017_New_Target_Steering_tests4`1520|1486491114613|2_7_2017_Test0`1521|1486493163152|2_7_2017_Test1`1522|1487097541900|2_14_2017_Test0`1523|1487181361834|2_15_2017_Test0`1524|1487194601117|2_15_2017_Test1`1548|1489608886371|3_15_2017_Run1`1549|1489686271856|3_16_2017_Run1`1550|1489700338702|3_16_2017_Run2`1551|1489702912301|3_16_2017_Run3`1552|1489768639011|3_17_2017_Run0`1553|1489778816552|3_17_2017_Run1`1554|1490026466115|3_20_2017_Run0`1555|1490028539062|3_20_2017_Run1`1556|1490030448187|3_20_2017_Run2`1557|1490043616373|3_20_2017_Run3`1558|1490045916076|3_20_2017_Run4`1559|1490047361482|3_20_2017_Run5`1560|1490117308922|3_21_2017_Run0`1561|1490131123193|3_21_2017_Run1`1562|1490211762853|3_22_2017_Run0`1563|1490376164052|3_24_2017_Run0`1565|1490986952843|3_31_2017_Run0`1566|1491237683544|4_3_2017_Run0`1567|1491238689221|4_3_2017_Run1`1568|1491239783607|4_3_2017_Run2`1569|1491241472730|4_3_2017_Run3`1570|1491325716745|4_4_2017_Run0`1571|1491330553544|4_4_2017_Run1`1572|1491331931603|4_4_2017_Run2`1573|1491420931243|4_5_2017_Run0`1574|1491491793665|4_6_2017_Run0`1600|1493740926183|5_03_2017_Run0`1601|1494004809462|5_05_2017_Run0`1602|1494020524197|5_05_2017_Run1`1626|1496856583117|6_7_2017_Run0`1635|1499036396505|7_2_17_Run0`1672|1502399131380|2017_08_10_test0`1705|1505772787049|2017_09_18_run0`1706|1506368979437|2017_09_25_run0`1707|1506532737120|2017_09_27_run0`1708|1506624343839|2017_09_28_run0`1736|1507577405227|2017_10_09_0`1737|1507661247837|2017_10_10_0`1738|1507744615184|2017_10_11_0`1739|1507790168061|2017_10_12_0`1740|1507795478470|2017_10_12_1`1741|1507796372354|2017_10_12_2`1742|1507798058686|2017_10_12_3`1743|1507800390881|2017_10_12_4`1744|1507868371411|2017_10_12_5`1745|1507881931245|2017_10_13_0`1746|1507882883211|2017_10_13_1`1747|1508182977022|2017_10_16_0`1748|1508273997460|2017_10_17_0`1749|1508354870590|2017_10_18_0`1750|1508434427905|2017_10_19_0`1751|1508448516990|2017_10_19_run1`1858|1515098837085|2018_01_04_run0`1859|1515529852292|2018_01_09_run0`1860|1515615198077|2018_01_10_run0`1861|1515627595108|2018_01_10_run2`1862|1515709504007|2018_01_11_run0`1863|1515725022038|2018_01_11_run1`1864|1515880435432|2018_01_13_run1`1865|1515880797578|2018_01_13_run1a`1866|1515880989634|2018_01_13_run1a2`1867|1515882956314|2018_01_13_run2`1868|1515884876292|2018_01_13_run3`1869|1515886836108|2018_01_13_run4`1870|1515888786745|2018_01_13_run5`1871|1515890637146|2018_01_13_run6`1872|1515892500167|2018_01_13_run7`1873|1515894366379|2018_01_13_run8`1874|1515896223354|2018_01_13_run9`1875|1515898270164|2018_01_13_run10`1876|1515900380956|2018_01_13_run11`1877|1515902284443|2018_01_13_run12`1878|1515904147173|2018_01_13_run13`1879|1515906007994|2018_01_13_run14`1880|1515907918619|2018_01_13_run15`1881|1515909919820|2018_01_13_run16`1882|1515910850505|2018_01_13_run17`1883|1515912692253|2018_01_13_run18`1884|1515969349113|2018_01_14_run0`1885|1515970327685|2018_01_14_run0a`1886|1515972518150|2018_01_14_run1`1887|1515974419498|2018_01_14_run3`1888|1515976446633|2018_01_14_run4`1889|1515978317693|2018_01_14_run5`1890|1515980219588|2018_01_14_run6`1891|1515982134893|2018_01_14_run7`1892|1516390462754|2018_01_19_run0`1893|1516392048264|2018_01_19_run1`1894|1516395370447|2018_01_19_run2`1895|1516409670742|2018_01_19_slow_run1`1896|1516409990536|2018_01_19_slow_run2`1897|1516411565065|2018_01_19_dcs_tests_run1`1898|1516652948160|2018_01_22_run0_calibration`1899|1516658118420|2018_01_22_run1_calibration`1900|1516670086639|2018_01_22_run3_second_surface_calibration`1901|1516670855677|2018_01_22_run4_second_surface_calibration`1902|1516671297935|2018_01_22_run5_second_surface_calibration`1903|1516682780506|2018_01_22_run6_third_surface_calibration`1904|1516688028159|2018_01_22_run7_third_surface_calibration`1905|1516689313065|2018_01_22_run8_third_surface_dcs_run1`1906|1516689530072|2018_01_22_run9_third_surface_water_run`1907|1516750549354|2018_01_23_run0`1908|1516835277599|2018_01_24_run0`1909|1516863133421|2018_01_24_run1_arg`1910|1516928367046|2018_01_25_run0_lys-gly`1911|1516952748318|2018_01_25_run1_lys`1967|1520455887631|2018_03_07_test0`1968|1520465354602|2018_03_07_test1`1969|1520536235347|2018_03_08_test0`1970|1520891237628|2018_03_12_test0`1971|1521142261410|2018_03_15_test0`1972|1521168001547|2018_03_15_test1`1973|1521241239782|2018_03_16_test0`1974|1521493784710|2018_03_19_test0`1975|1521568757701|2018_03_20_test0`1976|1521657853600|2018_03_21_test0`1977|1521745550655|2018_03_22_test0`1978|1521821193869|2018_03_23_test0`1979|1522095708913|2018_03_26_test0`1980|1522100744314|2018_03_26_test1`1981|1522175399366|2018_03_27_test0`1982|1522176039979|2018_03_27_run1`2154|1533430674819|2018_08_4_sanity_check`2165|1534184411779|2018_08_13_run0`2166|1534448030778|2018_08_16_run0`2167|1534451670556|2018_08_16_run1`2168|1534531135633|2018_08_17_run0`2181|1535272204924|2018_08_26_run0`2182|1535400448193|2018_08_27_run0`2183|1535666602553|2018_08_30_run0`2184|1535756234899|2018_08_31_run0`2214|1538083525029|2018_09_27_run0`2215|1538429718154|2018_10_1_run0`2216|1538603007659|2018_10_3_run0`2217|1538684744954|2018_10_4_run0`2218|1538768365391|2018_10_5_run0`2219|1539715781435|2018_10_16_run0`2220|1539813060818|2018_10_17_run0`2243|1541542485229|2018_11_06_run0`2244|1541631569914|2018_11_07_run0`2251|1543453436284|2018_11_28_run0`2252|1543521533920|2018_11_29_run0`2254|1544047152788|2018_12_05_run0`2266|1545854700790|2018_12_26_run0`2267|1545857787562|2018_12_26_run1`2268|1545860581418|2018_12_26_run2`2269|1545860929895|2018_12_26_run3`2270|1546031613038|2018_12_28_run0`2277|1546975563005|2019_01_08_run1`2278|1547506589941|2019_01_14_run0`2279|1548742847291|2019_01_28_run0`2280|1548745596406|2019_01_28_run1`2281|1548747461355|2019_01_28_run2`2288|1550912547284|2019_02_23_run0`2289|1551323763979|2019_02_27_run0`2290|1551332432015|2019_02_27_run1`2291|1551333737744|2019_02_27_run2`2292|1551338145094|2019_02_27_run3`2360|1552602944970|2019_03_14_run0`2364|1553106881267|2019_03_20_run1`2365|1553127223714|2019_03_20_run2`2366|1553196310445|2019_03_21_run0`2367|1553280892289|2019_03_22_run0`2403|1556211829962|2019_04_25_run0`2407|1556741730784|2019_05_1_run0`2408|1556749270226|2019_05_1_run2`2409|1556888589272|2019_05_3_run0`2441|1557443415272|2019_05_9_run_ice_0`2442|1557445109049|2019_05_9_run_ice_1`2443|1557454725421|2019_05_9_run_ice_2`2527|1559147370730|2019_05_29_run0`2528|1559147518059|2019_05_29_run1`2529|1559148351208|2019_05_29_run2`2530|1559151487656|2019_05_29_run3`2531|1559155205780|2019_05_29_run4`2541|1559757520450|2019_07_05_test0`}Stanford{666|1421681801360|2015_01_19_test1`667|1421773371266|2015_01_20_test1`668|1421776346870|2015_01_20_test2`669|1421781220800|2015_01_20_test3`670|1421782740494|2015_01_20_test4`671|1421789697241|2015_01_20_test5`672|1421857846995|2015_01_21_test1`673|1421951323128|2015_01_22_test1`674|1422033067123|2015_01_23_test1`}Ejecta{675|1422310398247|2015_01_26_test`676|1422470542310|2015_01_26_control`677|1422484753229|2015_01_26_run1`678|1422560334946|2015_01_26_run2`679|1422567015845|2015_01_26_run3`680|1422646458948|2015_01_26_run4`681|1422894046324|2015_01_26_run5`682|1422907457323|2015_01_26_run6`726|1428597228565|tests_4_9_15`729|1429112535221|run3`730|1429113107080|tests_4_15_15`2240|1541173313608|2018_11_02_run0`2241|1541178960239|2018_11_02_run1`2242|1541462087429|2018_11_05_run0`2245|1541778415720|2018_11_09_run0`2246|1541883955464|2018_11_10_run0`}Ablation Exp 3{684|1423679352816|First Tests`685|1423754577687|Beam Finding`695|1425338533559|Second Tests`696|1425340285124|Second Beam Finding`697|1425487567029|Run1`698|1425503042460|Run2`704|1426620090217|Run3`705|1426623577075|Run4`706|1426716471683|Run5`707|1426793528453|Run6`708|1426800561731|Run7`709|1426871474810|Run8`710|1426877499185|Run9`711|1426884078906|Run10`712|1427131596754|Run11`713|1427218665764|Run12`714|1427299802049|Run13`715|1427302797902|Run14`716|1427306270787|Run15`717|1427317410627|Run16`718|1427320997551|Run17`719|1427471888905|Run17 Redo`720|1427489862958|Run18`721|1427493028958|Run19`722|1427730657485|Run20`723|1427735825748|Run21`724|1427739801028|Run22`}Ablation Exp 4{741|1430775548599|run1`742|1430854076047|run2`743|1430857014056|run3`744|1430943547433|run4`745|1430945291485|run5`746|1430949079038|run6`747|1430951715538|run7`748|1431022119620|run8`749|1431029450393|run9`750|1431031165748|run10`751|1431034981217|run10`752|1431035013032|run11`753|1431037275038|run12`754|1431460292362|run13`755|1431641537468|run14`756|1431710553916|run15`757|1431985485396|run16`758|1432055748800|run17`759|1432064467363|run18`}Ablation Exp 5{786|1438110926491|Run1`787|1438115789474|AlignmentTest`788|1438287973948|AlignmentTest2`789|1438291706836|AlignmentTest3`790|1438380812597|MirrorTest1`793|1438461700395|MirrorTest2`794|1438616853467|test0`795|1438621757751|AlignmentTest4`796|1438632037481|Run1New`797|1438719976837|2015_8_4Run2`798|1438725426579|2015_8_4Run3`799|1438795991644|2015_8_5Run4`800|1438808246348|2015_8_5Run5`801|1438880082287|2015_8_6Run6`802|1438891110177|2015_8_6Run7`804|1438969288072|2015_8_7Run8`806|1439830877092|2015_8_17_Run9`807|1439915967708|2015_8_18_Run10`808|1440188662730|2015_8_21_Run11`810|1440194196367|2015_8_21_Run12`}Jim Andrew{921|1445023087374|10_16_2015_run_1`922|1445045031043|10_17_2015_run_2`923|1445291225782|10_19_2015_run_1`926|1445380883588|10_20_2015_Run_3`}Hyperdust{978|1456249823300|2016_2_23_test0`979|1456252149318|2016_2_23_test1`980|1456252772888|2016_2_23_test2`981|1456254292668|2016_2_23_test3`982|1456255186281|2016_2_23_test4`983|1456260302864|2016_2_23_test5`984|1456260879791|2016_2_23_test6`985|1456261417337|2016_2_23_test7`986|1456419021833|2016_2_25_test0`987|1456419592711|2016_2_25_test1`988|1456420238703|2016_2_25_test2`989|1456420551923|2016_2_25_test3`990|1456420960154|2016_2_25_test`991|1456421285217|2016_2_25_test7(missed last one) test(blank)`992|1456421681125|2016_2_25_test8`993|1456422125224|2016_2_25_test9`994|1456506894812|2016_2_26_test0`995|1456508862347|2016_2_26_test1`996|1456509459641|2016_2_26_test2`997|1456511242887|2016_2_26_test3`998|1456512546206|2016_2_26_test4`999|1456513309012|2016_2_26_test5`1000|1456514240949|2016_2_26_test6`1001|1456515656779|2016_2_26_test7`1002|1456521261948|2016_2_26_test8`1003|1456521985902|2016_2_26_test9`1004|1456522438583|2016_2_26_test10`1005|1456522828128|2016_2_26_test11`1006|1456523291909|2016_2_26_test12`1007|1456524007697|2016_2_26_test13`1008|1456524559573|2016_2_26_test14`1062|1458836243466|2016_3_28_HyperLin_test0`1063|1459205653954|2016_3_28_HyperLin_test1`1064|1459266456109|2016_3_29_HyperLin_test0`1065|1459267340226|2016_3_29_HyperLin_test1`1066|1459267982184|2016_3_29_HyperLin_test2`1067|1459268953031|2016_3_29_HyperLin_test3`1068|1459269569984|2016_3_29_HyperLin_test4`1069|1459270705529|2016_3_29_HyperLin_test5`1070|1459271221378|2016_3_29_HyperLin_test6`1071|1459272092920|2016_3_29_HyperLin_test7`1072|1459272588469|2016_3_29_HyperLin_test8`1073|1459273400665|2016_3_29_HyperLin_test9`1074|1459281372193|2016_3_29_HyperLin_test10`1075|1459282777088|2016_3_29_HyperLin_test11`1076|1459283352111|2016_3_29_HyperLin_test12`1077|1459284721953|2016_3_29_HyperLin_test13`1078|1459285053133|2016_3_29_HyperLin_test14`1079|1459285808010|2016_3_29_HyperLin_test15`1080|1459285982188|2016_3_29_HyperLin_test16`1081|1459286231995|2016_3_29_HyperLin_test17`1082|1459286568396|2016_3_29_HyperLin_test18`1083|1459286762186|2016_3_29_HyperLin_test19`1084|1459287171879|2016_3_29_HyperLin_test20`}SUDA{1023|1457539529063|2016_03_09_2016_test0`1108|1461166909011|2016_4_20_test0`1109|1461168753395|2016_4_20_test1`1110|1461169157026|2016_4_20_test2`1111|1461169350232|2016_4_20_test3`1112|1461169475292|2016_4_20_test4`1113|1461169853559|2016_4_20_test5`1114|1461170009272|2016_4_20_test6`1115|1461170216759|2016_4_20_test7`1116|1461192139060|2016_4_20_test8`1117|1461193069020|2016_4_20_test9`1118|1461193314941|2016_4_20_test10`1119|1461193701984|2016_4_20_test11`1120|1461193980648|2016_4_20_test12`1121|1461194254422|2016_4_20_test13`1122|1461248324452|2016_4_21_test1`1123|1461250151015|2016_4_21_test2`1124|1461250285461|2016_4_21_test3`1125|1461250463565|2016_4_21_test4`1126|1461250691970|2016_4_21_test5`1127|1461256689551|2016_4_21_test6`1306|1469052167780|2016_07_20_test0`1323|1471363428612|2016_08_16_test0`1324|1471367940933|2016_08_16_test1`1325|1471370372538|2016_08_16_test2`1326|1471374615140|2016_08_16_test3`1327|1471375654346|2016_08_16_test4`1328|1471377342978|2016_08_16_test5`1329|1471377934510|2016_08_16_test6`1330|1471378882611|2016_08_16_test7`1331|1471379640390|2016_08_16_test8`1332|1471380281937|2016_08_16_test9`1333|1471381453188|2016_08_16_test10`1334|1471382315954|2016_08_16_test11`1335|1471446677778|2016_08_17_test0`1336|1471447486525|2016_08_17_test1`1337|1471448351899|2016_08_17_test2`1338|1471448776735|2016_08_17_test3`1339|1471449278171|2016_08_17_test4`1340|1471453626927|2016_08_17_test5`1341|1471463769401|2016_08_17_test6`1342|1471468203636|2016_08_17_test7`1343|1471469147315|2016_08_17_test8`1344|1471469948023|2016_08_17_test9`1345|1471471080797|2016_08_17_test10`1346|1471472294054|2016_08_17_test11`1347|1471533580548|2016_08_18_test0`1348|1471534582638|2016_08_18_test1`1349|1471538210755|2016_08_18_test2`1350|1471538676805|2016_08_18_test3`1351|1471539122177|2016_08_18_test4`1352|1471539404288|2016_08_18_test5`1353|1471539733517|2016_08_18_test6`1354|1471540483573|2016_08_18_test7`1355|1471541281210|2016_08_18_test8`1356|1471541577095|2016_08_18_test9`1357|1471541823070|2016_08_18_test10`1358|1471542032683|2016_08_18_test11`1359|1471619664788|2016_08_19_test0`1360|1471620863079|2016_08_19_test1`1361|1471621312791|2016_08_19_test2`1362|1471621807318|2016_08_19_test3`1363|1471622251857|2016_08_19_test4`1364|1471622895000|2016_08_19_test5`1365|1471623570640|2016_08_19_test6`1366|1471624066836|2016_08_19_test7`1367|1471626303936|2016_08_19_test8`1368|1471627400531|2016_08_19_test9`1415|1477409782944|10_25_2016_test0`1416|1477414523343|10_25_2016_test1`1417|1477417018251|10_25_2016_test2`1418|1477494066406|10_26_2016_test0`1419|1477502169024|10_26_2016_test3`1420|1477583342084|10_27_2016_test0`1421|1477589883153|10_27_2016_test1`1422|1477596952562|10_27_2016_test2`1458|1478622961198|11_08_2016_test0`1459|1478626179420|11_08_2016_test1`1460|1478627061862|11_08_2016_test2`1461|1478716458098|11_09_2016_test0`1462|1478717994594|11_09_2016_test1`1463|1478720609439|11_09_2016_test2`1464|1478724126096|11_09_2016_test3`1465|1478726885420|11_09_2016_test4`1466|1478797046550|11_10_2016_test0`1467|1478809521118|11_10_2016_test1`1468|1478813033702|11_10_2016_test2`1469|1478814208440|11_10_2016_test3`1470|1478814790150|11_10_2016_test4`1471|1478815409226|11_10_2016_test5`1472|1478816196080|11_10_2016_test6`1473|1478816831817|11_10_2016_test7`1474|1478817208098|11_10_2016_test8`1475|1478817450443|11_10_2016_test`1476|1478817657930|11_10_2016_test10`1477|1478818038921|11_10_2016_test11`1479|1479156664650|11_14_2016_test0`1480|1479163289367|11_14_2016_test1`1481|1479225373657|11_15_2016_test0`1482|1479226671651|11_15_2016_test1`1483|1479227544669|11_15_2016_test2`1484|1479228138483|11_15_2016_test3`1485|1479230410908|11_15_2016_test4`1486|1479231126248|11_15_2016_test5`1487|1479231322360|11_15_2016_test6`1488|1479231748141|11_15_2016_test7`1489|1479232348482|11_15_2016_test8`1490|1479233582471|11_15_2016_test9`1491|1479234126027|11_15_2016_test10`1603|1494361989166|5_09_2017_Run0`1604|1494431737572|5_10_2017_Run0`1605|1494450519510|5_10_2017_Run1`1606|1494519785890|5_11_2017_Run0`1607|1494524043587|5_11_2017_Run1`1608|1494527957303|5_11_2017_Run2`1609|1494606563917|5_12_2017_Run0`1610|1494616620567|5_12_2017_Run1`1611|1494623890460|5_12_2017_Run2`1612|1494863928777|5_15_2017_Run0`1613|1494949899226|5_16_2017_Run0`1614|1494954585748|5_16_2017_Run1`1615|1494962056341|5_16_2017_Run2`1616|1495036296860|5_17_2017_Run0`1617|1495039523059|5_17_2017_Run1`1618|1495041761293|5_17_2017_Run12`1619|1495042341081|5_17_2017_Run2`1620|1495051212551|5_17_2017_Run3`1621|1495056151510|5_17_2017_Run4`1622|1495209004666|5_19_2017_Run0`1627|1497281694017|6_12_2017_Run0`1628|1497547252378|6_15_2017_Run0`1629|1497559789548|6_15_2017_Run1`1630|1497627072238|6_16_2017_Run0`1677|1504021096247|2017_08_29_Run0`1678|1504035738438|2017_08_29_Run1`1679|1504039515045|2017_08_29_Run2`1680|1504042828920|2017_08_29_Run3`1681|1504107446070|2017_08_30_Run0`1682|1504117454621|2017_08_30_Run1`1683|1504125128863|2017_08_30_Run2`1684|1504127650617|2017_08_30_Run3`1685|1504189646049|2017_08_31_Run0`1686|1504192583504|2017_08_31_Run1`1687|1504199678963|2017_08_31_Run2`1688|1504281675067|2017_09_1_Run0`1689|1504286077506|2017_09_1_Run1`1690|1504623429418|2017_09_5_Run0`1691|1504713400169|2017_09_6_Run0`1752|1508866050143|2017_10_24_run0`1753|1508878012777|2017_10_24_run1`1754|1508882864996|2017_10_24_run2`1755|1508949586958|2017_10_25_run0`1757|1510244682629|2017_11_09_run0`1758|1510264894293|2017_11_09_run1`1759|1510332229996|2017_11_10_run0`1760|1510333768241|2017_11_10_run1`1852|1513791386747|2017_12_20_run0`1853|1513871357950|2017_12_21_run0`1854|1514228374147|2017_12_25_run0`1855|1514327588787|2017_12_26_run0`1856|1514408252733|2017_12_27_run0`2003|1524672392922|2018_04_25_test0`2004|1524678080389|2018_04_25_test1`2005|1524842205645|2018_04_27_test0`2006|1524846598121|2018_04_27_test1`2007|1524848021258|2018_04_27_test2`2008|1524850349978|2018_04_27_test3`2009|1524853467997|2018_04_27_test4`2010|1525188248955|2018_05_1_test0`2011|1525191279138|2018_05_1_test1`2012|1525193850617|2018_05_1_test2`2013|1525195978274|2018_05_1_test3`2014|1525197283180|2018_05_1_test4`2015|1525198398917|2018_05_1_test5`2016|1525202973125|2018_05_1_test6`2017|1525205115118|2018_05_1_test7`2018|1525206580930|2018_05_1_test8`2019|1525209646327|2018_05_1_test9`2020|1525211085199|2018_05_1_test10`2021|1525213115756|2018_05_1_test11`2057|1528817798559|2018_06_12_test0`2058|1528820312085|2018_06_12_test1`2059|1528821084324|2018_06_12_test2`2060|1528821817390|2018_06_12_test3`2061|1528822448088|2018_06_12_test4`2062|1528824270632|2018_06_12_test5`2063|1528827763799|2018_06_12_test6`2064|1529424917483|2018_06_19_test0`2065|1529426773536|2018_06_19_test1`2066|1529428124694|2018_06_19_test2`2067|1529429346080|2018_06_19_test3`2068|1529430565513|2018_06_19_test4`2069|1529432887625|2018_06_19_test5`2070|1529434395590|2018_06_19_test6`2071|1529436570928|2018_06_19_test7`2225|1540827080205|2018_10_29_run0`2226|1540830742600|2018_10_29_run1`2227|1540834453239|2018_10_29_run2`2228|1540845689569|2018_10_29_run3`2229|1540912654908|2018_10_30_run1`2230|1540922747722|2018_10_30_run2`2231|1540933378551|2018_10_30_run3`2232|1540934993904|2018_10_30_run4`2233|1540937006286|2018_10_30_run5`2234|1540938995599|2018_10_30_run6`2369|1554823332513|2019_04_09_run0`2370|1554828046115|2019_04_09_run1`2371|1554833381566|2019_04_09_run2`2372|1554835854770|2019_04_09_run3`2373|1554839192372|2019_04_09_run4`2374|1554840729061|2019_04_09_run5`2375|1554841173480|2019_04_09_run6`2376|1554842942986|2019_04_09_run7`2377|1554844767387|2019_04_09_run8`2378|1554847487719|2019_04_09_run9`2379|1554847980462|2019_04_09_run10`2380|1554997203930|2019_04_11_run0`2381|1554998260093|2019_04_11_run1`2382|1554998599588|2019_04_11_run2`2383|1554999022039|2019_04_11_run3`2384|1554999512198|2019_04_11_run4`2385|1554999947512|2019_04_11_run5`2386|1555000226500|2019_04_11_run6`2387|1555000612161|2019_04_11_run7`2388|1555001676578|2019_04_11_run8`2389|1555002199687|2019_04_11_run9`2546|1560959101959|2019_06_19_run0`2547|1560961922595|2019_06_19_run1`2548|1560962655575|2019_06_19_run2`2549|1560963506847|2019_06_19_run3`2550|1560969347993|2019_06_19_run4`2551|1560970366371|2019_06_19_run5`2552|1560973847088|2019_06_19_run6`2553|1560974629089|2019_06_19_run7`2554|1560975083341|2019_06_19_run8`2555|1560976673271|2019_06_19_run9`}Orion Heat Shield{1057|1458314784136|2016_03_18_test1`1058|1458325023431|2016_03_18_test2`1059|1458332264679|2016_03_18_test3`1060|1458338456767|2016_03_18_test4`}Mark Loeffler{1223|1466452771480|2016_06_20_Run1`1224|1466520962535|2016_06_21_Run1`1225|1466693963581|2016_06_23_Run1`1226|1467211056221|2016_06_29_Run0`1227|1467214423547|2016_06_29_Run1`1639|1499717428234|SCDE717-2`1640|1499794219027|2017_07_11_SCDE717-3`1641|1499959687764|2017_07_13_SCDE717-1`}ENIJA{1236|1467652424940|2016_07_04_test0`1237|1467655681030|2016_07_04_test1`1238|1467660030502|2016_07_04_test2`1239|1467736400211|2016_07_05_test0`1240|1467737179512|2016_07_05_test1`1241|1467737580745|2016_07_05_test2`1242|1467737947538|2016_07_05_test3`1243|1467738708575|2016_07_05_test4`1244|1467740341877|2016_07_05_test5`1245|1467741676259|2016_07_05_test6`1246|1467742440249|2016_07_05_test7`1247|1467757777545|2016_07_05_test8`1248|1467758256441|2016_07_05_test9`1249|1467759025622|2016_07_05_test10`1250|1467760066352|2016_07_05_test11`1251|1467820018897|2016_07_06_test0`1252|1467821158800|2016_07_06_test1`1253|1467824233653|2016_07_06_test2`1254|1467825539322|2016_07_06_test3`1255|1467831747517|2016_07_06_test4`1256|1467834905319|2016_07_06_test5`1257|1467837844615|2016_07_06_test6`1258|1467839039287|2016_07_06_test7`1259|1467841336500|2016_07_06_test8`1260|1467907234621|2016_07_07_test0`1261|1467909098278|2016_07_07_test1`1262|1467910401195|2016_07_07_test2`1263|1467911447956|2016_07_07_test3`1264|1467913164832|2016_07_07_test4`1265|1467913925344|2016_07_07_test5`1266|1467915596588|2016_07_07_test6`1267|1467917350779|2016_07_07_test7`1268|1467921275261|2016_07_07_test8`1269|1467922932473|2016_07_07_test9`1270|1467924581828|2016_07_07_test10`1271|1467925301206|2016_07_07_test11`1272|1467926112300|2016_07_07_test12`1273|1467927280383|2016_07_07_test13`1274|1467993294871|2016_07_08_test0`1275|1467994675994|2016_07_08_test1`1276|1467995921288|2016_07_08_test2`1277|1468355975912|2016_07_13_test0`1278|1468431025706|2016_07_13_test1`1279|1468856963562|2016_07_18_test0`1280|1468859364471|2016_07_18_test1`1281|1468860191401|2016_07_18_test2`1282|1468861064168|2016_07_18_test3`1283|1468872357729|2016_07_18_test4`1284|1468872551831|2016_07_18_test5`1285|1468872835663|2016_07_18_test6`1286|1468873150233|2016_07_18_test7`1287|1468873422492|2016_07_18_test8`1288|1468873697287|2016_07_18_test9`1289|1468874270070|2016_07_18_test10`1290|1468874666450|2016_07_18_test11`1291|1468875247563|2016_07_18_test12`1292|1468875508770|2016_07_18_test13`1293|1468875781389|2016_07_18_test14`1294|1468876187458|2016_07_18_test15`1295|1468876510982|2016_07_18_test16`1296|1468876847063|2016_07_18_test17`1297|1468877121921|2016_07_18_test18`1298|1468877364501|2016_07_18_test19`1299|1468948368108|2016_07_19_test0`1300|1468949163363|2016_07_19_test1`1301|1468949489595|2016_07_19_test2`1302|1468949831965|2016_07_19_test3`1303|1468950294301|2016_07_19_test4`1304|1468950463975|2016_07_19_test5`}Cassini{1423|1477931275926|10_31_2016_test0`1424|1477944650511|10_31_2016_test1`1425|1477950990037|10_31_2016_test3`1426|1478013109533|11_01_2016_test0`1427|1478015780081|11_01_2016_test1`1428|1478020540789|11_01_2016_test2`1429|1478031428471|11_01_2016_test3`1430|1478036862803|11_01_2016_test4`1431|1478038966650|11_01_2016_test5`1432|1478041403609|11_01_2016_test6`1433|1478042681639|11_01_2016_test7`1434|1478043869140|11_01_2016_test8`1435|1478102338121|11_02_2016_test0`1436|1478105589298|11_02_2016_test1`1437|1478107259644|11_02_2016_test2`1438|1478110158120|11_02_2016_test3`1439|1478117387610|11_02_2016_test4`1440|1478121531987|11_02_2016_test5`1441|1478122725300|11_02_2016_test6`1442|1478123758287|11_02_2016_test7`1443|1478125824853|11_02_2016_test8`1444|1478184984740|11_03_2016_test0`1445|1478186309796|11_03_2016_test1`1446|1478187245589|11_03_2016_test2`1447|1478188219753|11_03_2016_test3`1448|1478189602914|11_03_2016_test4`1449|1478191299477|11_03_2016_test5`1450|1478193278771|11_03_2016_test6`1451|1478195027136|11_03_2016_test7`1452|1478204499803|11_03_2016_test8`1453|1478207162144|11_03_2016_test9`1454|1478211059493|11_03_2016_test10`1455|1478213779751|11_03_2016_test12`1456|1478214481236|11_03_2016_test13`1457|1478215170842|11_03_2016_test14`1709|1506974957174|2017_10_02_run0`1710|1507062576744|2017_10_03_run1`1711|1507063930513|2017_10_03_run1`1712|1507064810928|2017_10_03_run2`1713|1507067381988|2017_10_03_run3`1714|1507072338604|2017_10_03_run4`1715|1507223706941|2017_10_05_run5a`1716|1507228489604|2017_10_05_run6a`1717|1507237308401|2017_10_05_run7a`1718|1507244079202|2017_10_05_run7b`1719|1507299286325|2017_10_06_run5b`1720|1507301767265|2017_10_06_run6b`1721|1507305387983|2017_10_06_run8b`1722|1507307834595|2017_10_06_run8a`1723|1507314166225|2017_10_06_run9a`1724|1507320421697|2017_10_06_run9b`1725|1507322696834|2017_10_06_run10a`1726|1507325104760|2017_10_06_run11a`1727|1507326173956|2017_10_06_run12a`1728|1507328139241|2017_10_06_run13a`1729|1507329758609|2017_10_06_run14a`1730|1507331518715|2017_10_06_run15a`1731|1507480587392|2017_10_08_run16a`1732|1507485752470|2017_10_08_run16b`1733|1507491986275|2017_10_08_run16c`1734|1507500217500|2017_10_08_run17a`1735|1507504547663|2017_10_08_run18a`1822|1512061997601|2017_11_30_run0`1823|1512066849929|2017_11_30_run0b`1824|1512071418329|2017_11_30_run1a`1825|1512076613581|2017_11_30_run1b`1826|1512083443958|2017_11_30_run2a`1827|1512087485489|2017_11_30_run2b`1828|1512145449024|2017_12_1_run0a`1829|1512146286059|2017_12_01_run0a`1830|1512149594122|2017_12_1_run0b`1831|1512156990652|2017_12_1_run1a`1832|1512164033542|2017_12_1_run1b`1833|1512166884883|2017_12_1_run2a`1834|1512319421568|2017_12_3_run0a`1835|1512324854380|2017_12_3_run1a`1836|1512404756553|2017_12_4_run0a`1837|1512409629827|2017_12_4_run1a`1838|1512425725384|2017_12_4_run2a`1839|1512431893788|2017_12_4_run3a`1840|1512491392033|2017_12_5_run0a`1841|1512498101924|2017_12_5_run0b`1842|1512501872121|2017_12_5_run0c`1843|1512507070295|2017_12_5_run1`1844|1512578057239|2017_12_6_run0a`1845|1512583396229|2017_12_6_run0b`1846|1512586147127|2017_12_6_run1a`1847|1512595120629|2017_12_6_run2a`1848|1512600088702|2017_12_6_run2b`1849|1512601219433|2017_12_6_run3a`1850|1512604817939|2017_12_6_run4a`2072|1529943874089|2018_06_25_test0`2073|1529945796422|2018_06_25_test1`2074|1529946646567|2018_06_25_test2`2075|1529948056826|2018_06_25_test0a`2076|1529953874755|2018_06_25_test0b`2077|1529967090235|2018_06_25_test1a`2078|1530052589934|2018_06_26_run0a`2079|1530112574894|2018_06_27_run0a`2080|1530114707899|2018_06_27_run0b`2081|1530125470856|2018_06_27_run1a`2082|1530128494746|2018_06_27_run1b`2083|1530137278320|2018_06_27_run2a`2084|1530138626001|2018_06_27_run2b`2085|1530207274014|2018_06_27_run3a`2086|1530208913431|2018_06_27_run3b`2087|1530216556957|2018_06_27_run4a`2088|1530218943567|2018_06_27_run4b`2089|1530285874193|2018_06_28_run5a`2090|1530290557080|2018_06_28_run5b`2091|1530301275392|2018_06_28_run6a`2092|1530302649338|2018_06_28_run6b`2093|1530310206201|2018_06_28_run7a`2094|1530545103501|2018_06_28_run7b`2095|1530555331519|2018_07_02_run8a`2096|1530558227402|2018_07_02_run8b`2097|1530568872142|2018_07_02_run9a`2098|1530570279737|2018_07_02_run9b`2099|1530631720036|2018_07_03_run0a`2100|1530633126574|2018_07_03_run0b`2101|1530642860775|2018_07_03_run1a`2102|1530643789754|2018_07_03_run1b`2103|1530805664731|2018_07_05_run0a`2104|1530808806715|2018_07_05_run0b`2105|1530817579549|2018_07_05_run1a`2106|1530819306429|2018_07_05_run1b`2107|1530832352137|2018_07_05_run2a`2108|1530891391839|2018_07_06_run3a`2109|1530892960006|2018_07_06_run4a`2110|1530895462789|2018_07_06_run5a`2111|1530897172557|2018_07_06_run6a`2112|1530899319972|2018_07_06_run6b`2113|1530903720049|2018_07_06_run3b`2114|1530906314018|2018_07_06_run2b`2115|1530910071070|2018_07_06_run4b`2116|1530913898790|2018_07_06_run5b`2117|1531151096937|2018_07_09_run0a`2118|1531153563892|2018_07_09_run0b`2119|1531155162012|2018_07_09_run0c`2120|1531156391488|2018_07_09_run0d`2121|1531157471565|2018_07_09_run0e`2122|1531158735829|2018_07_09_run0f`2123|1531160197583|2018_07_09_run0g`2124|1531161488038|2018_07_09_run0h`2125|1531165728313|2018_07_09_run1a`2126|1531167762167|2018_07_09_run1b`2127|1531170254536|2018_07_09_run1c`2128|1531172494876|2018_07_09_run1d`2129|1531177783608|2018_07_09_run2a`2130|1531179023628|2018_07_09_run2b`2131|1531235889741|2018_07_10_run0a`2132|1531237634882|2018_07_10_run0b`2133|1531238854237|2018_07_10_run0c`2134|1531240022987|2018_07_10_run0d`2135|1531243433423|2018_07_10_run0f`2136|1531245516084|2018_07_10_run0g`2137|1531246871703|2018_07_10_run0h`2138|1531248773521|2018_07_10_run1a`2139|1531252034045|2018_07_10_run1b`2140|1531255791341|2018_07_10_run1c`2141|1531261125022|2018_07_10_run1d`2142|1531321601770|2018_07_11_run0a`2143|1531324902948|2018_07_11_run0b`2144|1531329497291|2018_07_11_run1b`2171|1534950848176|2018_08_22_run0a`2172|1534955236399|2018_08_22_run0aa`2173|1534957896727|2018_08_22_run0aaa`2174|1534970271062|2018_08_22_run0bbb`2175|1535039164280|2018_08_23_run1a`2176|1535050622464|2018_08_23_run1b`2177|1535060523110|2018_08_23_run1c`2178|1535134159062|2018_08_24_run1d`2179|1535146446627|2018_08_24_run0d`2180|1535150248188|2018_08_24_run2a`}Slowdown{1624|1496421124492|6_2_2017_Run1`1625|1496433825863|6_2_2017_Run2`1673|1502991349351|2017_08_17_Exp12_Run1`1674|1503440051694|2017_08_22_Exp12_Run2`1675|1503505207438|2017_08_23_Exp12_Run3`1692|1504820760524|2017_09_7_Run4`1693|1504823199207|2017_09_7_Run5`1694|1504826654542|2017_09_7_Run6`1695|1504829443003|2017_09_7_Run7`1696|1504880495379|2017_09_8_Run8`1697|1504885733193|2017_09_8_Run9`1698|1504899231250|2017_09_8_Run10`1699|1504904953925|2017_09_8_Run11`1700|1504908904138|2017_09_8_Run12`1701|1504911357395|2017_09_8_Run13`1702|1504913515604|2017_09_8_Run14`1703|1504914596523|2017_09_8_Run15`}SPECIES{1631|1498160673826|6_22_2017_Run0`1632|1498232799677|6_23_2017_Run0`1633|1498493755046|6_26_2017_Run0`1634|1498591059999|6_27_2017_Run1`}Tim Glotch Reflectance{1636|1499193846645|7_4_17_Run0`1637|1499293584352|7_5_17_Run1`1638|1499717145214|7_5_17_Run1`2194|1536604328771|2018_09_10_run0`2195|1536709968080|2018_09_12_run0`2196|1536791082945|2018_09_13_run0`2197|1536862724247|2018_09_13_run1`2198|1536868030355|2018_09_13_run2`2199|1536869620209|2018_09_13_run3`2200|1536872541377|2018_09_13_run4`2201|1537289464517|2018_09_18_run0`2202|1537300764237|2018_09_18_run1`2203|1537368009392|2018_09_19_run0`2204|1537461414912|2018_09_20_run0`2205|1537471810508|2018_09_20_run1`2206|1537482694213|2018_09_20_run2`2207|1537554985535|2018_09_21_run0`2208|1537562679780|2018_09_21_run1`2209|1537572191614|2018_09_21_run2`2210|1537828527029|2018_09_24_run0`}CASSINI_LEMMS{1761|1510695641407|2017_11_14_run0`1762|1510699517719|2017_11_14_run1`1763|1510701054538|2017_11_14_run2`1764|1510701986560|2017_11_14_run3`1765|1510702851455|2017_11_14_run4`1766|1510703503081|2017_11_14_run5`1767|1510704116452|2017_11_14_run6`1768|1510704978267|2017_11_14_run7`1769|1510766788736|2017_11_15_run8`1770|1510768120664|2017_11_15_run9`1771|1510768916886|2017_11_15_run10`1772|1510769596988|2017_11_15_run11`1773|1510770920583|2017_11_15_run13`1774|1510771950577|2017_11_15_run14`1775|1510778036866|2017_11_15_run16`1776|1510779104645|2017_11_15_run17`1777|1510779765349|2017_11_15_run18`1778|1510780163973|2017_11_15_run19`1779|1510780578089|2017_11_15_run20`1780|1510781385942|2017_11_15_run21`1781|1510786346812|2017_11_15_run24`1782|1510787073903|2017_11_15_run25`1783|1510787641808|2017_11_15_run26`1784|1510788730141|2017_11_15_run27`1785|1510789957060|2017_11_15_run28`1786|1510790914452|2017_11_15_run29`1787|1510850369676|2017_11_16_run31`1788|1510854430021|2017_11_16_run35`1789|1510855663239|2017_11_16_run36`1790|1510858121481|2017_11_16_run39`1791|1510861902516|2017_11_16_run40`1792|1510932984838|2017_11_16_run41`1793|1510934588313|2017_11_16_run42`1794|1510935279930|2017_11_16_run43`1795|1510937961596|2017_11_16_run44`1796|1510942499619|2017_11_16_run45`1797|1510943038428|2017_11_16_run46`1798|1510945043834|2017_11_16_run47`1799|1510945157038|2017_11_16_run48`1800|1510950344779|2017_11_16_run49`1801|1510950970288|2017_11_16_run50`1802|1510951708633|2017_11_16_run51`1803|1510953314911|2017_11_16_run52`}BMWS CZECH Inst{1804|1511196053193|2017_11_20_run0`1805|1511200263302|2017_11_20_run1`1806|1511201561364|2017_11_20_run2`1807|1511204319027|2017_11_20_run3`1808|1511297286637|2017_11_21_run0`1809|1511304288573|2017_11_21_run1`1810|1511369255391|2017_11_22_run0`1811|1511381884635|2017_11_22_run1`1812|1511540227829|2017_11_24_run0`1813|1511543808424|2017_11_24_run1`1814|1511545188612|2017_11_24_run2`1815|1511714385507|2017_11_26_run0`1816|1511720567351|2017_11_26_run2`2149|1533049815730|2018_07_31_run0a`2150|1533053628496|2018_07_31_run0b`2151|1533059422622|2018_07_31_run0c`2152|1533064703413|2018_07_31_run1a`2153|1533073114926|2018_07_31_run1b`}High Speed MCP{1817|1511894858131|2017_11_28_run0`1818|1511971071369|2017_11_29_run0`1819|1511975153057|2017_11_29_run1`1820|1511983873806|2017_11_29_run2`1821|1511985650221|2017_11_29_run3`}Masanori_Sensor{1933|1518722232343|2018_02_15_test0`1934|1518727198486|2018_02_15_test1`1935|1518731640052|2018_02_15_test2`1936|1518734924590|2018_02_15_test3`1937|1518796768650|2018_02_16_test0`1938|1518801552679|2018_02_16_test1`1939|1518804764368|2018_02_16_test2`1940|1518807112627|2018_02_16_test3`1941|1518809693042|2018_02_16_test5`1942|1518814446897|2018_02_16_test6`1943|1518818185354|2018_02_16_test7`1944|1519057747372|2018_02_19_test0`1945|1519062656776|2018_02_19_test1`1946|1519065695817|2018_02_19_test2`1947|1519068945081|2018_02_19_test3`1948|1519073523095|2018_02_19_test4`1949|1519141084555|2018_02_20_test0`1950|1519144821134|2018_02_20_test1`1951|1519161845811|2018_02_20_test2`1952|1519165149609|2018_02_20_test3`1953|1519229374597|2018_02_21_test0`1954|1519233261212|2018_02_21_test1`1955|1519237585931|2018_02_21_test2`1956|1519241692009|2018_02_21_test3`1957|1519246032622|2018_02_21_test4`1958|1519251278132|2018_02_21_test5`}Carbon Foils{1983|1522278819177|2018_03_28_run0`1984|1522352695851|2018_03_29_run0`1985|1522363455328|2018_03_29_run1`1986|1522436288992|2018_03_30_run0`1987|1522447942182|2018_03_30_run1`1988|1522699896596|2018_04_02_test0`1989|1522707234903|2018_04_02_test1`1990|1522942960616|2018_04_05_test0`}Ring Target{2146|1531932604945|2018_07_18_jack_run1`2147|1531935425156|2018_07_18_jack_run2`2187|1536165160256|2018_09_04_run1`2188|1536167283050|2018_09_04_run2`2189|1536182780555|2018_09_04_run3`2190|1536185326166|2018_09_04_run4`2192|1536258785775|2018_09_06_run5`2193|1536260854001|2018_09_06_run6`}Q Impact{2155|1533655031368|2018_08_7_run1`2156|1533657140239|2018_08_7_run2`2157|1533675626879|2018_08_7_run3`2158|1533742636516|2018_08_8_run4`2159|1533746925947|2018_08_8_run5`2160|1533749698871|2018_08_8_run6`2161|1533829758945|2018_08_9_run7`2163|1533918464765|2018_08_10_run8`2164|1533930224312|2018_08_10_run9`2169|1534779337741|2018_08_20_run0`2170|1534865479455|2018_08_21_run0`2542|1560266059655|2019_06_11_test0`2543|1560268611375|2019_06_11_test1`2544|1560270197260|2019_06_11_test2`2545|1560272065560|2019_06_11_test3`2556|1561475942901|2019_06_25_test0`2557|1561480022786|2019_06_25_test1`2558|1561482641093|2019_06_25_test2`2559|1561565438463|2019_06_26_test0`2560|1561567738978|2019_06_26_test1`2561|1561569452424|2019_06_26_test2`2569|1561994824779|2019_07_01_test3`2570|1561998966629|2019_07_01_test4`2571|1562000380357|2019_07_01_test5`2572|1562081615782|2019_07_02_EdgeTest`2573|1562082459936|2019_07_02_test6`2574|1562084283000|2019_07_02_test7`2575|1562085784667|2019_07_02_test8`}Dust Trajectory Sensor{2211|1538055009245|2018_09_27_run0`2212|1538061461287|2018_09_27_run1`2213|1538063266239|2018_09_27_run2`2235|1541091351791|2018_11_01_run0`2238|1541098284876|2018_11_01_run2`2239|1541100255920|2018_11_01_run3`}Fossil{2221|1540233946183|2018_10_22_run0`2222|1540236902903|2018_10_22_run1`2223|1540316281838|2018_10_23_run0`2224|1540317993869|2018_10_23_run1`2253|1543960441848|2018_12_04_run0`2255|1544137778245|2018_12_06_run0`2256|1544896850432|2018_12_14_run0`2257|1544989900999|2018_12_16_run0`2258|1545155065096|2018_12_18_run0`2259|1545157006435|2018_12_18_run1`2260|1545326886070|2018_12_20_run0`2261|1545328674002|2018_12_20_run1`2262|1545329179225|2018_12_20_run2`2263|1545411868574|2018_12_21_test0`2264|1545424603954|2018_12_21_test1`2265|1545430546576|2018_12_21_test2`2271|1546545827557|2019_01_03_run0`2272|1546551969749|2019_01_03_run1`2273|1546619736881|2019_01_04_run0`2274|1546638444623|2019_01_04_run1`2275|1546878655661|2019_01_07_run0`2276|1546975187427|2019_01_08_run0`2282|1548875963651|2019_01_30_run0`2283|1548971909030|2019_01_31_run0`2284|1548973903042|2019_01_31_run1`2285|1549069546924|2019_02_1_run0`2286|1549076286429|2019_02_1_run1`2287|1549079315269|2019_02_1_run2`2414|1557246312004|2019_05_7_run0`2415|1557253361273|2019_05_7_run1`2416|1557259277996|2019_05_7_run2`2417|1557335107741|2019_05_8_run0`2418|1557338777413|2019_05_8_run1`}DCS{2236|1541094735995|2018_11_01_run0`2237|1541097350715|2018_11_01_run1`}Mitchell_Cassini{2293|1551721553434|2019_03_04_test0`2294|1551724195349|2019_03_04_test1`2295|1551725404841|2019_03_04_test2`2296|1551728217638|2019_03_04_test3`2297|1551730179890|2019_03_04_test3f`2298|1551732155742|2019_03_04_test4`2299|1551734137478|2019_03_04_test4f`2300|1551736052294|2019_03_04_test5`2301|1551738548501|2019_03_04_test5f`2302|1551740971787|2019_03_04_test6`2303|1551743335724|2019_03_04_test6f`2304|1551801736355|2019_03_05_test7`2305|1551803968878|2019_03_05_test7f`2306|1551805861321|2019_03_05_test8`2307|1551808452544|2019_03_05_test8f`2308|1551811317139|2019_03_05_test9f`2309|1551816158373|2019_03_05_test10`2310|1551818065655|2019_03_05_test10f`2311|1551820258359|2019_03_05_test11`2312|1551821992694|2019_03_05_test11f`2313|1551824323433|2019_03_05_test12`2314|1551826151130|2019_03_05_test12f`2315|1551888470559|2019_03_06_test13`2316|1551893713257|2019_03_06_test13f`2317|1551896363619|2019_03_06_test14`2318|1551898445540|2019_03_06_test14f`2319|1551902349831|2019_03_06_test15`2320|1551905645955|2019_03_06_test15f`2321|1551907616622|2019_03_06_test16f`2322|1551909255392|2019_03_06_test17f`2323|1551974524734|2019_03_07_test18`2324|1551977644724|2019_03_07_test18f`2325|1551979801294|2019_03_07_test19`2326|1551982625240|2019_03_07_test19f`2327|1551985569076|2019_03_07_test20`2328|1551988750634|2019_03_07_test20f`2329|1551990840885|2019_03_07_test21f`2330|1551993105994|2019_03_07_test22f`2331|1552061088062|2019_03_08_test23`2332|1552063297577|2019_03_08_test23f`2333|1552066144589|2019_03_08_test24`2334|1552068744925|2019_03_08_test24f`2335|1552072951942|2019_03_08_test25`2336|1552075370084|2019_03_08_test25f`2337|1552077809080|2019_03_08_test26f`2338|1552080544449|2019_03_08_test27f`2339|1552316886295|2019_03_11_test28`2340|1552320829036|2019_03_11_test28f`2341|1552322948058|2019_03_11_test29`2342|1552325917161|2019_03_11_test29f`2343|1552327945762|2019_03_11_test30`2344|1552330139628|2019_03_11_test30f`2345|1552331744420|2019_03_11_test31f`2346|1552333229927|2019_03_11_test31`2347|1552335145520|2019_03_11_test32`2348|1552337354190|2019_03_11_test32f`2349|1552338567448|2019_03_11_test33`2350|1552403167594|2019_03_11_test34`2351|1552405444691|2019_03_11_test34f`2352|1552407374024|2019_03_11_test35`2353|1552409277571|2019_03_11_test35f`2354|1552411368428|2019_03_11_test36`2355|1552413256175|2019_03_11_test36f`2356|1552415223245|2019_03_12_test37`2357|1552417154425|2019_03_12_test37f`2358|1552419046125|2019_03_12_test38`2359|1552421354657|2019_03_12_test38f`}Impact Bonding{2391|1555345854121|2019_04_15_run0`2392|1555349639121|2019_04_15_run1`2393|1555357382627|2019_04_15_run2`2395|1555436706635|2019_04_16_run1`2396|1555440842003|2019_04_16_run2`2401|1556031199854|2019_04_23_run0`2402|1556121727928|2019_04_24_run0`2404|1556225162123|2019_04_25_run1`2405|1556292521574|2019_04_26_run0`2406|1556302122821|2019_04_26_run1`2410|1556895925882|2019_05_3_run1`2411|1556899296923|2019_05_3_run2`2412|1556902433880|2019_05_3_run3`2413|1556904767073|2019_05_3_run4`}Ash{2419|1557420462136|2019_05_9_run0`2420|1557421833149|2019_05_9_run1`2421|1557422928977|2019_05_9_run2`2422|1557423503586|2019_05_9_run3`2423|1557423963693|2019_05_9_run4`2424|1557424789725|2019_05_9_run5`2425|1557425359750|2019_05_9_run6`2426|1557426200817|2019_05_9_run7`2427|1557427215479|2019_05_9_run8`2428|1557427899292|2019_05_9_run9`2429|1557428651319|2019_05_9_run10`2430|1557429144199|2019_05_9_run11`2431|1557429802227|2019_05_9_run12`2432|1557430488949|2019_05_9_run13`2433|1557431156925|2019_05_9_run14`2434|1557431874586|2019_05_9_run15`2435|1557432940383|2019_05_9_run16`2436|1557434337683|2019_05_9_run17`2437|1557435693419|2019_05_9_run18`2438|1557436344773|2019_05_9_run19`2439|1557437473920|2019_05_9_run20`2440|1557438450678|2019_05_9_run21`2461|1558461239242|2019_05_21_run0`2462|1558463499557|2019_05_21_run1`2463|1558464261382|2019_05_21_run2`2464|1558464980411|2019_05_21_run3`2465|1558465483926|2019_05_21_run4`2466|1558465955655|2019_05_21_run5`2467|1558466421490|2019_05_21_run6`2468|1558466857740|2019_05_21_run7`2469|1558467569862|2019_05_21_run8`2470|1558468372532|2019_05_21_run9`2471|1558469057237|2019_05_21_run10`2472|1558469885386|2019_05_21_run11`2473|1558470639601|2019_05_21_run12`2474|1558471418255|2019_05_21_run13`2475|1558472192907|2019_05_21_run14`2476|1558473141881|2019_05_21_run15`2477|1558473922071|2019_05_21_run16`2478|1558474442654|2019_05_21_run17`2479|1558474967863|2019_05_21_run18`2480|1558475517556|2019_05_21_run19`2481|1558475906922|2019_05_21_run20`2482|1558476807799|2019_05_21_run21`2483|1558477443525|2019_05_21_run22`2484|1558478348182|2019_05_21_run23`2485|1558479359736|2019_05_21_run24`2486|1558479742562|2019_05_21_run25`2487|1558540163968|2019_05_22_run0`2488|1558543500000|2019_05_22_run1`2489|1558544838466|2019_05_22_run2`2490|1558546283631|2019_05_22_run3`2491|1558547828784|2019_05_22_run4`2493|1558552237242|2019_05_22_run5`2494|1558553586650|2019_05_22_run6`2495|1558554517451|2019_05_22_run7`2496|1558555404889|2019_05_22_run8`2497|1558556661624|2019_05_22_run9`2498|1558557838626|2019_05_22_run10`2499|1558558622846|2019_05_22_run11`2500|1558559239460|2019_05_22_run12`2501|1558559943599|2019_05_22_run13`2502|1558560565787|2019_05_22_run14`2503|1558561297397|2019_05_22_run15`2504|1558561999412|2019_05_22_run16`2506|1558644380934|2019_05_23_run0`2507|1558645285435|2019_05_23_run1`2508|1558645673344|2019_05_23_run2`2509|1558646628209|2019_05_23_run3`2510|1558647339311|2019_05_23_run4`2511|1558647828343|2019_05_23_run5`2512|1558648130948|2019_05_23_run6`2513|1558648866101|2019_05_23_run7`2514|1558649364740|2019_05_23_run8`2515|1558650023870|2019_05_23_run9`2516|1558650929987|2019_05_23_run10`2517|1558651570614|2019_05_23_run11`2518|1558652049511|2019_05_23_run12`2519|1558652277538|2019_05_23_run13`2520|1558652568647|2019_05_23_run14`2521|1558653008044|2019_05_23_run15`2522|1558653324228|2019_05_23_run16`2523|1558653757041|2019_05_23_run17`}Kevlar Tether 2{2448|1557937328917|2019_05_15_runA155`}Kevlar Tether{2449|1557937499735|2019_05_15_A1`2450|1557942127413|2019_05_15_A2`2454|1558020778913|2019_05_16_A1`2455|1558031426484|2019_05_16_A3`2456|1558039316218|2019_05_16_A4`2457|1558102499813|2019_05_17_A5`2458|1558107221848|2019_05_17_A2`2460|1558453748242|2019_05_21_B1`2505|1558627977052|2019_05_23_B1`2525|1558711911516|2019_05_24_B3`2526|1559060769466|2019_05_28_B2`2562|1561570906710|2019_06_26_run0`2563|1561579829609|2019_06_26_run1`2565|1561653302943|2019_06_27_run0`2566|1561657306407|2019_06_27_run1`2567|1561658629995|2019_06_27_run2`}FPGA Redesign{2532|1559160207014|2019_05_29_run0`2533|1559238021058|2019_05_30_run0`2534|1559239052083|2019_05_30_run1`2535|1559240403253|2019_05_30_run2`2536|1559241652739|2019_05_30_run3`2537|1559244423151|2019_05_30_run4`}"
              }
              frame True {
                n53 = local read "Working Directory"() -> (w77:path)
                n54 = local read "Numeric"() -> (w81:dbl)
                n55 = call "labview_sessions_generate.vi"("pswd"="Password", "ip"="Server IP Address", "user"="Username", "Numeric"=w81, "Path"=w77) -> ("Session Generator Output"=w75:string, "return code"=w83:i32, "error"=→"Session Generator Output":string)  [unwired: 4 in]
                n56 = Not Equal To 0?(x=w83) -> (x != 0?=w76:bool)
                n57 = local write "Numeric"(w83) -> ()
                n58 = local write "Delimited Input String"(w75) -> ()
                n59 = Equal?(x=w83, y=25) -> (x = y?=w84:bool)
                n60 = Not(x=w84) -> (.not. x?=w85:bool)
                n61 = local write "Calculating Sessions"(w84) -> ()
                n62 = local write "Authentication Failure"(w85) -> ()
              }
            }
          }
          frame #1 {
            # "Sorry"
            # "The delimiters are @ , } , { ` and |"
            # "Material Name { ID | Batch Description`ID|Batch Descption}Material Name{ etc...\n@\nExperiment Group Name { ID|description`ID|Descrption}Experiment Group Name{ etc..."
            # "This delimited input string contains a format for the dropdown menu data from the python program, as passing data structures back and forth can only be done through stdin and stdout strings. Here, the format is"
            n63 = local read "Delimited Input String"() -> (w88:string)
            n64 = call "create_material_experiment_lists.vi"("Delimited Input String"=w88) -> ("Batch List by Material"=→"Batch List by Material":string[], "Material Name List"=→"Material Name List":string[], "Experiment Group Names List"=w87:string[], "Exerimement List by Group"=→"Exerimement List by Group":string[])  [unwired: 7 in]
            "Experiment Group Names List" <- w87
            n65 = property on="Experiment Group" class="CmbBox"("Strings[]"=w87) -> ()  [unwired: 2 in, 2 out]
          }
          frame #2 {
            n66 = property on="Experiment Group" class="CmbBox"("Val(Sgnl)"="All") -> ()  [unwired: 2 in, 2 out]
          }
        }
      }
      n67 = local read "Working Directory"() -> (w45:path)
      n68 = Build Path(base path=w45, name or relative path="heatmaps") -> (appended path=w48:path)
      n69 = call <vilib>:"Check if File or Folder Exists.vi"("path"=w48) -> ("file or folder exists?"=w47:bool)  [unwired: 8 in, 2 out]
      n70 = case shown="True" w47 {
        tunnel: w48 -> [w65 _]
        frame False {
          n71 = Create Folder(path (use dialog)=w65) -> ()  [unwired: 2 in, 3 out]
        }
        frame True {
        }
      }
      n72 = Bundle("Average_results_rates.png", "Average_results_particle_count.png", "Average_results_runtime.png", "Optimal_results_rates.png", "Optimal_results_particle_count.png", "Optimal_results_runtime.png", "Poor_results_rates.png", "Poor_results_particle_count.png", "Poor_results_runtime.png", "results_session_qualities.png", "results_particles_qualities.png", "results_sessions_durations.png", "results_sessions_particle_counts.png") -> (w60:T5)  [unwired: 1 in]
    }
    frame #3 {
      n73 = while {
        tunnel: w98 -> [w100]
        stop <- w99 stop-if-true
        # "While the stop button has not been pressed, listen for events"
        n74 = local write "Calculating"(FALSE ("Boolean")) -> ()
        n75 = event shown="[0] \"Calculate Results\": Value Change" {
          selector: _ -> [_ _ _ _ _ _ _ _ _ _ _ _]
          dyn-events: _ -> [_ _ _ _ _ _ _ _ _ _ _ _]
          timeout: _ -> [_ _ _ _ _ _ _ _ _ _ _ _]
          tunnel: [_ _ _ _ _ _ _ _ _ "End Program" _ _] -> w99
          tunnel: w100 -> [w104 _ _ _ _ _ _ _ _ _ _ _]
          event "Calculate Results": Value Change {
            n76 = event-data() -> ()  [unwired: 1 in, 6 out]
            n77 = local write "Calculating"(TRUE ("Running")) -> ()
            n78 = flat-sequence {
              tunnel: [w107] -> w103
              tunnel: w104 -> [w114]
              tunnel: w103 -> [w113]
              frame #0 {
                # "Check validity of arguments, if not valid, display a popup, such as if the timestamps are out of order"
                n79 = local write "Calculate Results"(FALSE ("Calculate Results")) -> ()
                n80 = control-ref of="Velocity Maximum (km/s)"() -> (w112:refnum<vi>)
                n81 = control-ref of="Lower Integer Timestamp"() -> (w109:refnum<vi>)
                n82 = control-ref of="Upper Integer Timestamp"() -> (w110:refnum<vi>)
                n83 = control-ref of="Velocity Minimun  (km/s)"() -> (w111:refnum<vi>)
                n84 = call "validate_arguments.vi"("vmin"=w111, "upper time"=w110, "lower time"=w109, "vmax"=w112) -> ("Problem"=w108:bool, "String"=→"User warnings":string)  [unwired: 6 in]
                n85 = Not(x=w108) -> (.not. x?=w107:bool)
              }
              frame #1 {
                n86 = case shown="True" w113 {
                  tunnel: w114 -> [_ w116]
                  frame False {
                    n87 = property on="User warnings" class="Str"("Visible"=TRUE) -> ()  [unwired: 2 in, 2 out]
                  }
                  frame True {
                    n88 = flat-sequence {
                      tunnel: w116 -> [w169]
                      frame #0 {
                        w124 = ""
                        # "Take all the user controls, pass them to the subVI which appends them to a request string, ouputs the results string.\nHere we parse the results string and display them accordingly"
                        n89 = property on="User warnings" class="Str"("Visible"=FALSE) -> ()  [unwired: 2 in, 2 out]
                        n90 = local read "Lower Integer Timestamp"() -> (w164:i64)
                        n91 = local read "Upper Integer Timestamp"() -> (w163:i64)
                        n92 = local read "Working Directory"() -> (w157:path)
                        n93 = Bundle("Velocity Minimun  (km/s)"="Velocity Minimun  (km/s)", "Velocity Maximum (km/s)"="Velocity Maximum (km/s)") -> (w153:T6)  [unwired: 1 in]
                        n94 = call "labview_results_get.vi"("Path"=w157, "Dust ID"="Dust ID", "Upper Timestamp"=w163, "Velocity Limits"=w153, "Lower Timestamp"=w164, "Min mass"="Minimum Mass (kg)", "Particle Quality"="Estimate Dust Quality", "Max mass"="Maxiumum Mass (kg)", "Session Quality"="Estimate Session Quality", "Experiment ID"="Experiment ID", "Make heatmap"="Create Heatmap", "Dust Material"="Dust Material") -> ("Results Output"=w151:string, "Results Error/Debug"=→"Results Error/Debug":string, "Request"=→"Rate Results Request":string)  [unwired: 13 in]
                        "Results Output" <- w151
                        n95 = Search/Split String(string=w151, search string/char (-)="\r\n") -> (substring before match=w140:string, match + rest of string=w148:string)  [unwired: 1 in, 1 out]
                        n96 = call <vilib>:"Trim Whitespace.vi"("string"=w148) -> ("trimmed string"=w147:string)  [unwired: 1 in]
                        n97 = Search/Split String(string=w140, search string/char (-)="|") -> (substring before match=w136:string)  [unwired: 1 in, 2 out]
                        n98 = Search/Split String(string=w147, search string/char (-)="\r\n") -> (substring before match=w143:string, match + rest of string=w146:string)  [unwired: 1 in, 1 out]
                        n99 = Decimal String To Number(string=w136, default (0L)=0.0) -> (number=w133:dbl)  [unwired: 1 in, 1 out]
                        n100 = Divide(x=w133, y=60) -> (x/y=w131:dbl)
                        n101 = Equal?(x="No data found", y=w136) -> (x = y?=w125:bool)
                        n102 = Divide(x=w131, y=60) -> (x/y=w130:dbl)
                        n103 = call <vilib>:"Trim Whitespace.vi"("string"=w146) -> ("trimmed string"=w141:string)  [unwired: 1 in]
                        n104 = Search/Split String(string=w143, search string/char (-)=" |") -> (substring before match=w129:string)  [unwired: 1 in, 2 out]
                        n105 = call "Build Text"("hour_rate"=w133, "min_rate"=w131, "sec_rate"=w130) -> ("Result"=w135:string)  [unwired: 11 in, 1 out]
                        n106 = Select(t=w136, s=w125, f=w135) -> (s? t:f=→"Average Rate of Particle Detection":string)
                        n107 = Concatenate Strings(w129, "/hour") -> (w123:string)
                        n108 = Select(t=w124, s=w125, f=w123) -> (s? t:f=→"Optimal Rate":string)
                        n109 = Search/Split String(string=w141, search string/char (-)=" |") -> (substring before match=w126:string)  [unwired: 1 in, 2 out]
                        n110 = Concatenate Strings(w126, "/hour") -> (w121:string)
                        n111 = Select(t=w124, s=w125, f=w121) -> (s? t:f=→"Poor Rate":string)
                      }
                      frame #1 {
                        n112 = local read "Average Rate of Particle Detection"() -> (w167:string)
                        n113 = Not Equal?(x=w167, y="No data found") -> (x != y?=w166:bool)
                        n114 = case shown="True" w166 {
                          tunnel: w169 -> [_ w232]
                          frame False {
                          }
                          frame True {
                            (unwired) ""
                            # "If the heatmap graphs were successfullly created, display them too. The text builders build their file names, and pull them up if they exist"
                            # "This huge mess is the repeated operation of resizing the 19 .png files and displaying them on the insights tab. Might be a neater way to do this, but it was fine at 3 graphs and things just got worse from there"
                            n115 = control-ref of="Session Dust Event Count Breakdown"() -> (w209:refnum<vi>)
                            n116 = local read "Dust Material"() -> (w176:string)
                            n117 = local read "Upper Timestamp"() -> (w178:timestamp)
                            n118 = control-ref of="Session Particle Quality Breakdown"() -> (w207:refnum<vi>)
                            n119 = control-ref of="Session Quality Breakdown"() -> (w230:refnum<vi>)
                            n120 = local read "Lower Timestamp"() -> (w179:timestamp)
                            n121 = Get Date/Time String(date format (0)=0, seconds (now)=w179) -> (date string=w189:string)  [unwired: 1 in, 1 out]
                            n122 = Get Date/Time String(date format (0)=0, seconds (now)=w178) -> (date string=w184:string)  [unwired: 1 in, 1 out]
                            n123 = local read "Working Directory"() -> (w191:path)
                            n124 = control-ref of="Session Duration Breakdown"() -> (w208:refnum<vi>)
                            n125 = control-ref of="optimal runtime"() -> (w217:refnum<vi>)
                            n126 = Build Path(base path=w191, name or relative path="heatmaps") -> (appended path=w172:path)
                            n127 = Search and Replace String(replace all?=TRUE, input string=w189, search string="/", replace string="-") -> (result string=w180:string)  [unwired: 4 in, 3 out]
                            n128 = control-ref of="avg runtime"() -> (w213:refnum<vi>)
                            n129 = control-ref of="optimal count"() -> (w197:refnum<vi>)
                            n130 = Search and Replace String(replace all?=TRUE, input string=w184, search string="/", replace string="-") -> (result string=w177:string)  [unwired: 4 in, 3 out]
                            n131 = control-ref of="optimal count"() -> (w216:refnum<vi>)
                            n132 = control-ref of="poor runtimes"() -> (w210:refnum<vi>)
                            n133 = control-ref of="poor counts"() -> (w212:refnum<vi>)
                            n134 = Unbundle(w232) -> (w206:string, w205:string, w204:string, w203:string, w196:string, w195:string, w194:string, w193:string, w202:string, w201:string, w200:string, w199:string, w198:string)
                            n135 = call "Build Text4"("start"=w180, "end"=w177, "material"=w176) -> ("Result"=w170:string)  [unwired: 11 in, 1 out]
                            n136 = call "Build Text2"("start"=w180, "end"=w177, "material"=w176) -> ("Result"=w173:string)  [unwired: 11 in, 1 out]
                            n137 = call "Build Text3"("start"=w180, "end"=w177, "material"=w176) -> ("Result"=w171:string)  [unwired: 11 in, 1 out]
                            n138 = call "Image_resize.vi"("String"=w198, "stripped path"=w191, "Picture in"=w207) -> ("2D Picture"=→"Session Dust Event Count Breakdown":picture)  [unwired: 8 in]
                            n139 = control-ref of="avg rate"() -> (w215:refnum<vi>)
                            n140 = call "Image_resize.vi"("String"=w201, "stripped path"=w191, "Picture in"=w230) -> ("2D Picture"=→"Session Quality Breakdown":picture)  [unwired: 8 in]
                            n141 = Build Path(base path=w172, name or relative path=w173) -> (appended path=w175:path)
                            n142 = control-ref of="avg count"() -> (w214:refnum<vi>)
                            n143 = call "Image_resize.vi"("String"=w203, "stripped path"=w191, "Picture in"=w217) -> ("2D Picture"=→"optimal rates":picture)  [unwired: 8 in]
                            n144 = call "Image_resize.vi"("String"=w195, "stripped path"=w191, "Picture in"=w216) -> ("2D Picture"=→"optimal runtime":picture)  [unwired: 8 in]
                            n145 = call "Image_resize.vi"("String"=w202, "stripped path"=w191, "Picture in"=w210) -> ("2D Picture"=→"poor runtimes":picture)  [unwired: 8 in]
                            n146 = call "Image_resize.vi"("String"=w200, "stripped path"=w191, "Picture in"=w209) -> ("2D Picture"=→"Session Particle Quality Breakdown":picture)  [unwired: 8 in]
                            n147 = call "Image_resize.vi"("String"=w199, "stripped path"=w191, "Picture in"=w208) -> ("2D Picture"=→"Session Duration Breakdown":picture)  [unwired: 8 in]
                            n148 = call "Image_resize.vi"("String"=w204, "stripped path"=w191, "Picture in"=w213) -> ("2D Picture"=→"avg runtime":picture)  [unwired: 8 in]
                            n149 = control-ref of="poor rates"() -> (w211:refnum<vi>)
                            n150 = call "Image_resize.vi"("String"=w196, "stripped path"=w191, "Picture in"=w197) -> ("2D Picture"=→"optimal count":picture)  [unwired: 8 in]
                            n151 = call "Image_resize.vi"("String"=w193, "stripped path"=w191, "Picture in"=w212) -> ("2D Picture"=→"poor counts":picture)  [unwired: 8 in]
                            n152 = call "Image_resize.vi"("String"=w206, "stripped path"=w191, "Picture in"=w215) -> ("2D Picture"=→"avg rate":picture)  [unwired: 8 in]
                            n153 = call <vilib>:"Check if File or Folder Exists.vi"("path"=w175) -> ("file or folder exists?"=w174:bool)  [unwired: 8 in, 2 out]
                            n154 = case shown="True" w174 {
                              tunnel: w173 -> [_ w244]
                              tunnel: w172 -> [_ w243]
                              tunnel: w171 -> [_ w242]
                              tunnel: w170 -> [_ w241]
                              frame False {
                                n155 = property on="Tab Control 2" class="TabCtl (strict)"() -> ("Pages"=w233:refnum<vi>[])  [unwired: 2 in, 2 out]
                                n156 = for {
                                tunnel: w233 -> [w236] mode=indexing
                                tunnel: bool[] [TRUE, TRUE, TRUE, FALSE] -> [w235] mode=indexing
                                n157 = property class="Page"(reference=w236, "PageVis"=w235) -> ()  [unwired: 1 in, 2 out]
                                }
                              }
                              frame True {
                                n158 = flat-sequence {
                                tunnel: w244 -> [w247]
                                tunnel: w243 -> [w248]
                                tunnel: w242 -> [w246]
                                tunnel: w241 -> [w245]
                                tunnel: [w248] -> w240
                                tunnel: [w247] -> w239
                                tunnel: [w246] -> w238
                                tunnel: [w245] -> w237
                                tunnel: w240 -> [w265]
                                tunnel: w239 -> [w264]
                                tunnel: w238 -> [w263]
                                tunnel: w237 -> [w262]
                                frame #0 {
                                n159 = control-ref of="2D runtime"() -> (w253:refnum<vi>)
                                n160 = control-ref of="2D rates"() -> (w252:refnum<vi>)
                                n161 = property on="Tab Control 2" class="TabCtl (strict)"() -> ("Pages"=w250:refnum<vi>[])  [unwired: 2 in, 2 out]
                                n162 = control-ref of="2D particle distribution"() -> (w251:refnum<vi>)
                                n163 = call "Image_resize.vi"("String"=w247, "stripped path"=w248, "Picture in"=w253) -> ("2D Picture"=→"2D runtime":picture)  [unwired: 8 in]
                                n164 = for {
                                tunnel: w250 -> [w258] mode=indexing
                                tunnel: bool[] [TRUE, TRUE, TRUE, TRUE] -> [w257] mode=indexing
                                n165 = property class="Page"(reference=w258, "PageVis"=w257) -> ()  [unwired: 1 in, 2 out]
                                }
                                n166 = call "Image_resize.vi"("String"=w246, "stripped path"=w248, "Picture in"=w252) -> ("2D Picture"=→"2D rates":picture)  [unwired: 8 in]
                                n167 = call "Image_resize.vi"("String"=w245, "stripped path"=w248, "Picture in"=w251) -> ("2D Picture"=→"2D particle distribution":picture)  [unwired: 8 in]
                                }
                                frame #1 {
                                n168 = Build Path(base path=w265, name or relative path=w263) -> (appended path=w260:path)
                                n169 = Build Path(base path=w265, name or relative path=w264) -> (appended path=w261:path)
                                n170 = Build Path(base path=w265, name or relative path=w262) -> (appended path=w259:path)
                                n171 = Delete(path (use dialog)=w261) -> ()  [unwired: 4 in, 3 out]
                                n172 = Delete(path (use dialog)=w260) -> ()  [unwired: 4 in, 3 out]
                                n173 = Delete(path (use dialog)=w259) -> ()  [unwired: 4 in, 3 out]
                                }
                                }
                              }
                            }
                            n174 = call "Image_resize.vi"("String"=w205, "stripped path"=w191, "Picture in"=w214) -> ("2D Picture"=→"avg count":picture)  [unwired: 8 in]
                            n175 = call "Image_resize.vi"("String"=w194, "stripped path"=w191, "Picture in"=w211) -> ("2D Picture"=→"poor rates":picture)  [unwired: 8 in]
                          }
                        }
                      }
                    }
                  }
                }
              }
            }
          }
          event "Minimum Mass (kg)": Value Change {
            # "Increment in powers of 10, not addition"
            n176 = event-data() -> ("OldVal"=w267:dbl, "NewVal"=w270:dbl)  [unwired: 1 in, 4 out]
            n177 = Subtract(x=w270, y=w267) -> (x-y=w269:dbl)
            n178 = Power Of 10(x=w269) -> (10^x=w268:dbl)
            n179 = Multiply(x=w267, y=w268) -> (x*y=w266:dbl)
            n180 = local write "Minimum Mass (kg)"(w266) -> ()
          }
          event "Maxiumum Mass (kg)": Value Change {
            # "Increment in powers of 10, not addition"
            n181 = event-data() -> ("OldVal"=w271:dbl, "NewVal"=w272:dbl)  [unwired: 1 in, 4 out]
            n182 = Subtract(x=w272, y=w271) -> (x-y=w275:dbl)
            n183 = Power Of 10(x=w275) -> (10^x=w274:dbl)
            n184 = Multiply(x=w271, y=w274) -> (x*y=w273:dbl)
            n185 = local write "Maxiumum Mass (kg)"(w273) -> ()
          }
          event "Dust Material": Value Change {
            n186 = event-data() -> ()  [unwired: 1 in, 6 out]
            n187 = flat-sequence {
              frame #0 {
                n188 = property on="Batches list" class="LstBox (strict)"("Item Names"=string[] []) -> ()  [unwired: 2 in, 2 out]
              }
              frame #1 {
                # "Here the string after the name (after the { ) is split by the batch delimiter ( ` ), then the names are added to the list ( | )"
                # "When a material is selected, the batches for the dust must be displayed in the listbox for choosing"
                n189 = local read "Material Name List"() -> (w290:string[])
                n190 = local read "Dust Material"() -> (w289:string)
                n191 = local read "Batch List by Material"() -> (w281:string[])
                n192 = Search 1D Array(1D array=w290, element=w289) -> (index of element=w277:i32)  [unwired: 1 in]
                n193 = Subtract(x=w277, y=1) -> (x-y=w279:i32)
                n194 = Index Array(array=w281, index=w279) -> (element=w287:string)
                n195 = Search/Split String(string=w287, search string/char (-)="{") -> (match + rest of string=w285:string)  [unwired: 1 in, 2 out]
                n196 = String Subset(string=w285, offset (0)=1) -> (substring=w284:string)  [unwired: 1 in]
                n197 = Spreadsheet String To Array(delimiter (Tab)="`", format string="%s", spreadsheet string=w284, array type (2D Dbl)=w281) -> (array=w280:string[])
                n198 = for {
                  tunnel: w280 -> [w297] mode=indexing
                  n199 = Search/Split String(string=w297, search string/char (-)="|") -> (match + rest of string=w294:string)  [unwired: 1 in, 2 out]
                  n200 = property on="Batches list" class="LstBox (strict)"() -> ("Item Names"=w292:string[])  [unwired: 2 in, 2 out]
                  n201 = String Subset(string=w294, offset (0)=1) -> (substring=w293:string)  [unwired: 1 in]
                  n202 = Insert Into Array(array=w292, new element=w293) -> (w291:string[])  [unwired: 1 in]
                  n203 = property on="Batches list" class="LstBox (strict)"("Item Names"=w291) -> ()  [unwired: 2 in, 2 out]
                }
              }
              frame #2 {
                n204 = local write "Dust ID"("" ("Dust ID")) -> ()
                n205 = property on="Confirm Selection" class="Bool (strict)"("Visible"=FALSE) -> ()  [unwired: 2 in, 2 out]
                n206 = property on="Batches list" class="LstBox (strict)"("Visible"=FALSE) -> ()  [unwired: 2 in, 2 out]
                n207 = property on="List Batches" class="Bool (strict)"("Visible"=TRUE) -> ()  [unwired: 2 in, 2 out]
              }
            }
          }
          event "Experiment Group": Value Change {
            n208 = event-data() -> ()  [unwired: 1 in, 6 out]
            n209 = flat-sequence {
              frame #0 {
                n210 = property on="Experiment Listbox" class="LstBox (strict)"("Item Names"=string[] ["All"]) -> ()  [unwired: 2 in, 2 out]
              }
              frame #1 {
                # "When an experiment group is selected, the experiments must be selected  for the listbox to display"
                n211 = local read "Experiment Group Names List"() -> (w315:string[])
                n212 = local read "Exerimement List by Group"() -> (w306:string[])
                n213 = local read "Experiment Group"() -> (w316:string)
                n214 = Search 1D Array(1D array=w315, element=w316) -> (index of element=w305:i32)  [unwired: 1 in]
                n215 = Subtract(x=w305, y=1) -> (x-y=w303:i32)
                n216 = Index Array(array=w306, index=w303) -> (element=w313:string)
                n217 = Search/Split String(string=w313, search string/char (-)="{") -> (match + rest of string=w312:string)  [unwired: 1 in, 2 out]
                n218 = String Subset(string=w312, offset (0)=1) -> (substring=w310:string)  [unwired: 1 in]
                n219 = Spreadsheet String To Array(delimiter (Tab)="`", format string="%s", spreadsheet string=w310, array type (2D Dbl)=w306) -> (array=w307:string[])
                n220 = for {
                  tunnel: w307 -> [w327] mode=indexing
                  # "For each of the experiments in the group, add the expeirment tag to the listbox"
                  n221 = Search/Split String(string=w327, search string/char (-)="|") -> (match + rest of string=w324:string)  [unwired: 1 in, 2 out]
                  n222 = String Subset(string=w324, offset (0)=1) -> (substring=w323:string)  [unwired: 1 in]
                  n223 = Search/Split String(string=w323, search string/char (-)="|") -> (match + rest of string=w321:string)  [unwired: 1 in, 2 out]
                  n224 = String Subset(string=w321, offset (0)=1) -> (substring=w317:string)  [unwired: 1 in]
                  n225 = property on="Experiment Listbox" class="LstBox (strict)"() -> ("Item Names"=w319:string[])  [unwired: 2 in, 2 out]
                  n226 = Insert Into Array(array=w319, new element=w317) -> (w318:string[])  [unwired: 1 in]
                  n227 = property on="Experiment Listbox" class="LstBox (strict)"("Item Names"=w318) -> ()  [unwired: 2 in, 2 out]
                }
              }
              frame #2 {
                n228 = property on="Show expeirments" class="Bool (strict)"("Visible"=TRUE) -> ()  [unwired: 2 in, 2 out]
                n229 = property on="Confirm Experiments" class="Bool (strict)"("Visible"=FALSE) -> ()  [unwired: 2 in, 2 out]
                n230 = local write "Experiment ID"("" ("Experiment ID")) -> ()
                n231 = property on="Experiment Listbox" class="LstBox (strict)"("Visible"=FALSE) -> ()  [unwired: 2 in, 2 out]
              }
            }
          }
          event "Confirm Experiments": Value Change {
            n232 = event-data() -> ()  [unwired: 1 in, 6 out]
            n233 = flat-sequence {
              frame #0 {
                n234 = local write "List of experiments"(string[] [] ("List of experiments")) -> ()
                n235 = local write "Experiment ID"("") -> ()
              }
              frame #1 {
                # "When the listbox selects the names of the experiments the user wants, the IDs for those indices must be added to the string that gets passed to the rate_results.py prorgam through the experiment ID string"
                n236 = local read "Experiment Group"() -> (w347:string)
                n237 = local read "Experiment Group Names List"() -> (w348:string[])
                n238 = Search 1D Array(1D array=w348, element=w347) -> (index of element=w345:i32)  [unwired: 1 in]
                n239 = local read "Exerimement List by Group"() -> (w343:string[])
                n240 = Subtract(x=w345, y=1) -> (x-y=w344:i32)
                n241 = Index Array(array=w343, index=w344) -> (element=w342:string)
                n242 = Search/Split String(string=w342, search string/char (-)="{") -> (match + rest of string=w340:string)  [unwired: 1 in, 2 out]
                n243 = local read "List of experiments"() -> (w335:string[])
                n244 = String Subset(string=w340, offset (0)=1) -> (substring=w338:string)  [unwired: 1 in]
                n245 = Spreadsheet String To Array(delimiter (Tab)="`", format string="%s", spreadsheet string=w338, array type (2D Dbl)=w335) -> (array=w334:string[])
                n246 = local write "List of experiments"(w334) -> ()
              }
              frame #2 {
                w350 = 0
                # "If the listbox didn't select the \"All\" option, the program adds all the expeirment IDs associated with the selected listbox indices to a concatenated string, Experiment ID"
                n247 = local read "Experiment Listbox"() -> (w352:i32[])
                n248 = Index Array(array=w352, index=w350) -> (element=w351:i32)
                n249 = Not Equal?(x=w351, y=w350) -> (x != y?=w349:bool)
                n250 = case shown="False" w349 {
                  frame False {
                    n251 = local read "List of experiments"() -> (w356:string[])
                    n252 = Array Size(array=w356) -> (size(s)=w355:i32)
                    n253 = Subtract(x=w355, y=1) -> (x-y=w353:i32)
                    n254 = for {
                      N: w353 -> [_]
                      i -> [w357]
                      n255 = local read "List of experiments"() -> (w365:string[])
                      n256 = Index Array(array=w365, index=w357) -> (element=w364:string)
                      n257 = local read "Experiment ID"() -> (w362:string)
                      n258 = Search/Split String(string=w364, search string/char (-)="|") -> (substring before match=w361:string)  [unwired: 1 in, 2 out]
                      n259 = Concatenate Strings(w362, w361) -> (w359:string)
                      n260 = Concatenate Strings(w359, ",") -> (w358:string)
                      n261 = local write "Experiment ID"(w358) -> ()
                    }
                  }
                  frame True {
                    n262 = local read "Experiment Listbox"() -> (w366:i32[])
                    n263 = for {
                      tunnel: w366 -> [w369] mode=indexing
                      n264 = local read "List of experiments"() -> (w370:string[])
                      n265 = Subtract(x=w369, y=1) -> (x-y=w367:i32)
                      n266 = Index Array(array=w370, index=w367) -> (element=w377:string)
                      n267 = Search/Split String(string=w377, search string/char (-)="|") -> (substring before match=w371:string)  [unwired: 1 in, 2 out]
                      n268 = local read "Experiment ID"() -> (w374:string)
                      n269 = Concatenate Strings(w374, w371) -> (w372:string)
                      n270 = Concatenate Strings(w372, ",") -> (w375:string)
                      n271 = local write "Experiment ID"(w375) -> ()
                    }
                  }
                }
              }
              frame #3 {
                n272 = local read "Experiment Group"() -> (w386:string)
                n273 = local read "Experiment ID"() -> (w384:string)
                n274 = property on="Show expeirments" class="Bool (strict)"("Visible"=TRUE) -> ()  [unwired: 2 in, 2 out]
                n275 = property on="Confirm Experiments" class="Bool (strict)"("Visible"=FALSE) -> ()  [unwired: 2 in, 2 out]
                n276 = property on="Experiment Listbox" class="LstBox (strict)"("Visible"=FALSE) -> ()  [unwired: 2 in, 2 out]
                n277 = Equal?(x=w386, y="All") -> (x = y?=w382:bool)
                n278 = Select(t="All", s=w382, f=w384) -> (s? t:f=w381:string)
                n279 = local write "Experiment ID"(w381) -> ()
              }
            }
          }
          event "Show expeirments": Value Change {
            # "Update what should be visible"
            n280 = event-data() -> ()  [unwired: 1 in, 6 out]
            n281 = property on="Experiment Listbox" class="LstBox (strict)"("Visible"=TRUE) -> ()  [unwired: 2 in, 2 out]
            n282 = property on="Show expeirments" class="Bool (strict)"("Visible"=FALSE) -> ()  [unwired: 2 in, 2 out]
            n283 = property on="Confirm Experiments" class="Bool (strict)"("Visible"=TRUE) -> ()  [unwired: 2 in, 2 out]
          }
          event "List Batches": Value Change {
            # "Update what should be visible"
            n284 = event-data() -> ()  [unwired: 1 in, 6 out]
            n285 = property on="Batches list" class="LstBox (strict)"("Visible"=TRUE) -> ()  [unwired: 2 in, 2 out]
            n286 = property on="List Batches" class="Bool (strict)"("Visible"=FALSE) -> ()  [unwired: 2 in, 2 out]
            n287 = property on="Confirm Selection" class="Bool (strict)"("Visible"=TRUE) -> ()  [unwired: 2 in, 2 out]
          }
          event "Confirm Selection": Value Change {
            n288 = event-data() -> ()  [unwired: 1 in, 6 out]
            n289 = flat-sequence {
              frame #0 {
                n290 = local write "List of material IDs"(string[] [] ("List of material IDs")) -> ()
                n291 = local write "Dust ID"("") -> ()
              }
              frame #1 {
                # "When the listbox selects the names of the batches the user wants, the IDs for those indices must be added to the string that gets passed to the rate_results.py prorgam through the Dust ID string"
                n292 = local read "Material Name List"() -> (w410:string[])
                n293 = local read "Batch List by Material"() -> (w412:string[])
                n294 = local read "Dust Material"() -> (w411:string)
                n295 = Search 1D Array(1D array=w410, element=w411) -> (index of element=w400:i32)  [unwired: 1 in]
                n296 = Subtract(x=w400, y=1) -> (x-y=w398:i32)
                n297 = Index Array(array=w412, index=w398) -> (element=w409:string)
                n298 = local read "List of material IDs"() -> (w402:string[])
                n299 = Search/Split String(string=w409, search string/char (-)="{") -> (match + rest of string=w407:string)  [unwired: 1 in, 2 out]
                n300 = String Subset(string=w407, offset (0)=1) -> (substring=w404:string)  [unwired: 1 in]
                n301 = Spreadsheet String To Array(delimiter (Tab)="`", format string="%s", spreadsheet string=w404, array type (2D Dbl)=w402) -> (array=w401:string[])
                n302 = local write "List of material IDs"(w401) -> ()
              }
              frame #2 {
                # "If the listbox didn't select the \"All\" option, the program adds all the Dust IDs associated with the selected listbox indices to a concatenated string, Dust ID"
                n303 = local read "Batches list"() -> (w417:i32[])
                n304 = Index Array(array=w417, index=0) -> (element=w415:i32)
                n305 = Equal To 0?(x=w415) -> (x = 0?=w414:bool)
                n306 = Not(x=w414) -> (.not. x?=w413:bool)
                n307 = case shown="False" w413 {
                  frame False {
                    n308 = local read "List of material IDs"() -> (w421:string[])
                    n309 = Array Size(array=w421) -> (size(s)=w420:i32)
                    n310 = Subtract(x=w420, y=1) -> (x-y=w418:i32)
                    n311 = for {
                      N: w418 -> [_]
                      i -> [w423]
                      n312 = local read "List of material IDs"() -> (w427:string[])
                      n313 = Add(x=w423, y=1) -> (x+y=w422:i32)
                      n314 = Index Array(array=w427, index=w422) -> (element=w432:string)
                      n315 = local read "Dust ID"() -> (w426:string)
                      n316 = Search/Split String(string=w432, search string/char (-)="|") -> (substring before match=w430:string)  [unwired: 1 in, 2 out]
                      n317 = Concatenate Strings(w426, w430) -> (w428:string)
                      n318 = Concatenate Strings(w428, ",") -> (w425:string)
                      n319 = local write "Dust ID"(w425) -> ()
                    }
                  }
                  frame True {
                    n320 = local read "Batches list"() -> (w433:i32[])
                    n321 = for {
                      tunnel: w433 -> [w442] mode=indexing
                      n322 = local read "List of material IDs"() -> (w441:string[])
                      n323 = Index Array(array=w441, index=w442) -> (element=w440:string)
                      n324 = Search/Split String(string=w440, search string/char (-)="|") -> (substring before match=w434:string)  [unwired: 1 in, 2 out]
                      n325 = local read "Dust ID"() -> (w438:string)
                      n326 = Concatenate Strings(w438, w434) -> (w436:string)
                      n327 = Concatenate Strings(w436, ",") -> (w435:string)
                      n328 = local write "Dust ID"(w435) -> ()
                    }
                  }
                }
              }
              frame #3 {
                n329 = local read "Dust Material"() -> (w445:string)
                n330 = local read "Dust ID"() -> (w444:string)
                n331 = Equal?(x=w445, y="Any Material") -> (x = y?=w446:bool)
                n332 = Select(t="All", s=w446, f=w444) -> (s? t:f=w443:string)
                n333 = local write "Dust ID"(w443) -> ()
              }
            }
            n334 = property on="Batches list" class="LstBox (strict)"("Visible"=FALSE) -> ()  [unwired: 2 in, 2 out]
            n335 = property on="Confirm Selection" class="Bool (strict)"("Visible"=FALSE) -> ()  [unwired: 2 in, 2 out]
            n336 = property on="List Batches" class="Bool (strict)"("Visible"=TRUE) -> ()  [unwired: 2 in, 2 out]
          }
          event "End Program": Value Change {
            # "Shuts down the while loop"
            n337 = event-data() -> ()  [unwired: 1 in, 6 out]
          }
          event "Lower Integer Timestamp", "Upper Integer Timestamp": Value Change {
            # "Any update to the integer timestamp updates the clock timestamp"
            n338 = event-data() -> ()  [unwired: 1 in, 6 out]
            n339 = local read "Upper Integer Timestamp"() -> (w458:i64)
            n340 = local read "Lower Integer Timestamp"() -> (w460:i64)
            n341 = Divide(x=w458, y=1000) -> (x/y=w454:dbl)
            n342 = Divide(x=w460, y=1000) -> (x/y=w452:dbl)
            n343 = Add(x=w454, y=2082844800.0) -> (x+y=w453:dbl)
            n344 = Add(x=w452, y=2082844800.0) -> (x+y=w450:dbl)
            n345 = To Time Stamp(1:w453) -> (0:w457:timestamp)
            n346 = To Time Stamp(1:w450) -> (0:w456:timestamp)
            n347 = property on="Upper Timestamp" class="AbsTime (strict)"("Val(Sgnl)"=w457) -> ()  [unwired: 2 in, 2 out]
            n348 = property on="Lower Timestamp" class="AbsTime (strict)"("Val(Sgnl)"=w456) -> ()  [unwired: 2 in, 2 out]
          }
          event "Upper Timestamp", "Lower Timestamp": Value Change {
            # "Any change to the clock timestamp updates the integer timestamp"
            n349 = event-data() -> ()  [unwired: 1 in, 6 out]
            n350 = local read "Lower Timestamp"() -> (w463:timestamp)
            n351 = local read "Upper Timestamp"() -> (w462:timestamp)
            n352 = Subtract(x=w463, y=2082844800.0) -> (x-y=w470:timestamp)
            n353 = Subtract(x=w462, y=2082844800.0) -> (x-y=w469:timestamp)
            n354 = To Quad Integer(1:w470) -> (0:w468:i64)
            n355 = To Quad Integer(1:w469) -> (0:w466:i64)
            n356 = Multiply(x=w468, y=1000) -> (x*y=w467:i64)
            n357 = Multiply(x=w466, y=1000) -> (x*y=w465:i64)
            n358 = local write "Lower Integer Timestamp"(w467) -> ()
            n359 = local write "Upper Integer Timestamp"(w465) -> ()
          }
        }
      }
      n360 = local write "Calculating Sessions"(FALSE ("Calculating Sessions")) -> ()
      n361 = Get Date/Time In Seconds() -> (seconds since 1Jan1904=w93:timestamp)
      n362 = local write "Finished Sessions"(TRUE ("Finished Sessions")) -> ()
      n363 = property on="Upper Timestamp" class="AbsTime (strict)"("Val(Sgnl)"=w93) -> ()  [unwired: 2 in, 2 out]
      n364 = local write "Authentication Failure"(FALSE ("Authentication Failure")) -> ()
    }
    frame #4 {
      # "This boolean controls whether or not the program relies on the saved data or pulls from the database. While the database is still not updated, this should be false as the program cannot access data. Once updated, this should be flipped to true"
      # "If the files exist, delete them"
      n365 = local read "Working Directory"() -> (w479:path)
      n366 = Unbundle(w480) -> (w474:string)  [unwired: 12 out]
      n367 = local write "Finished Sessions"(FALSE ("Finished Sessions")) -> ()
      n368 = Build Path(base path=w479, name or relative path=w474) -> (appended path=w481:path)
      n369 = local write "Cleaning Up"(TRUE ("Cleaning Up")) -> ()
      n370 = call <vilib>:"Check if File or Folder Exists.vi"("path"=w481) -> ("file or folder exists?"=w482:bool)  [unwired: 8 in, 2 out]
      n371 = Build Path(base path=w479, name or relative path="temp_data.pkl") -> (appended path=w483:path)
      n372 = call <vilib>:"Check if File or Folder Exists.vi"("path"=w483) -> ("file or folder exists?"=w477:bool)  [unwired: 8 in, 2 out]
      n373 = And(x=FALSE, y=w477) -> (x .and. y?=w475:bool)
      n374 = case shown="True" w475 {
        tunnel: w483 -> [_ w514]
        frame False {
        }
        frame True {
          n375 = Delete(path (use dialog)=w514) -> ()  [unwired: 4 in, 3 out]
        }
      }
      n376 = case shown="True" w482 {
        tunnel: w480 -> [_ w513]
        tunnel: w479 -> [_ w499]
        frame False {
        }
        frame True {
          n377 = Unbundle(w513) -> (w498:string, w497:string, w496:string, w495:string, w494:string, w493:string, w492:string, w491:string, w490:string, w489:string, w488:string, w487:string, w486:string)
          n378 = Build Path(base path=w499, name or relative path=w489) -> (appended path=w509:path)
          n379 = Build Path(base path=w499, name or relative path=w488) -> (appended path=w508:path)
          n380 = Build Path(base path=w499, name or relative path=w487) -> (appended path=w507:path)
          n381 = Build Path(base path=w499, name or relative path=w486) -> (appended path=w506:path)
          n382 = Build Path(base path=w499, name or relative path=w492) -> (appended path=w502:path)
          n383 = Build Path(base path=w499, name or relative path=w491) -> (appended path=w501:path)
          n384 = Build Path(base path=w499, name or relative path=w490) -> (appended path=w500:path)
          n385 = Build Path(base path=w499, name or relative path=w495) -> (appended path=w505:path)
          n386 = Build Path(base path=w499, name or relative path=w494) -> (appended path=w504:path)
          n387 = Build Path(base path=w499, name or relative path=w493) -> (appended path=w503:path)
          n388 = Build Path(base path=w499, name or relative path=w498) -> (appended path=w512:path)
          n389 = Build Path(base path=w499, name or relative path=w497) -> (appended path=w511:path)
          n390 = Build Path(base path=w499, name or relative path=w496) -> (appended path=w510:path)
          n391 = Delete(path (use dialog)=w509) -> ()  [unwired: 4 in, 3 out]
          n392 = Delete(path (use dialog)=w508) -> ()  [unwired: 4 in, 3 out]
          n393 = Delete(path (use dialog)=w507) -> ()  [unwired: 4 in, 3 out]
          n394 = Delete(path (use dialog)=w506) -> ()  [unwired: 4 in, 3 out]
          n395 = Delete(path (use dialog)=w502) -> ()  [unwired: 4 in, 3 out]
          n396 = Delete(path (use dialog)=w501) -> ()  [unwired: 4 in, 3 out]
          n397 = Delete(path (use dialog)=w500) -> ()  [unwired: 4 in, 3 out]
          n398 = Delete(path (use dialog)=w505) -> ()  [unwired: 4 in, 3 out]
          n399 = Delete(path (use dialog)=w504) -> ()  [unwired: 4 in, 3 out]
          n400 = Delete(path (use dialog)=w503) -> ()  [unwired: 4 in, 3 out]
          n401 = Delete(path (use dialog)=w512) -> ()  [unwired: 4 in, 3 out]
          n402 = Delete(path (use dialog)=w511) -> ()  [unwired: 4 in, 3 out]
          n403 = Delete(path (use dialog)=w510) -> ()  [unwired: 4 in, 3 out]
        }
      }
    }
  }
